vi "Beampointing_Multi_Pico3_HTT.vi"() -> ()   [LabVIEW 2020]
uses:
  Shared/GUI_Template/GUI_master/tcp_new_data_event.ctl
  Shared/GUI_Template/GUI_master/tcp new data cluster.ctl
  Ctrs/beam detection.ctl
  GUI_Beampointing_single_TRA/Ctrs/move.ctl
  General GUIs/Device GUIs/GUI_Cameras/Controls/Crosshair type def.ctl
  <vilib>/Utility/error.llb/DialogType.ctl
  <vilib>/Utility/file.llb/Read From Spreadsheet File (string).vi
  <userlib>/_OpenG.lib/array/array.llb/Filter 1D Array with Scalar (String)__ogtk.vi
  <userlib>/_OpenG.lib/array/array.llb/Filter 1D Array (String)__ogtk.vi
  <vilib>/Utility/file.llb/Write To Spreadsheet File (string).vi
  <vilib>/Analysis/NI_AALBase.lvlib
panel:
  out "x-y*floor(x/y)":dbl
  out "error out":errorcluster
  out "config path":string
  out "Array 3":bool[](array[boolean])
  out "Array 2":u16[](array[numeric])
  out "Array":u16[](array[numeric])
  out "Moving Y":string
  out "Moving X":string
  out "particles":T1(array[cluster])
  out "millisecond timer value":u32
  out "appended path":path
  out "millisecond timer 2":u32
  in  "GUIdevice 98":string="PicoPad_LCave"
  in  "Position.Axis 111::98":dbl=77.0 caption="Motor Axis 1" min=-999999.0 max=999999.0 format="%#_6f"
  in  "Position.Axis 112::98":dbl=77.0 caption="Motor Axis 1" min=-999999.0 max=999999.0 format="%#_6f"
  in  "Position.Axis 113::98":dbl=77.0 caption="Motor Axis 1" min=-999999.0 max=999999.0 format="%#_6f"
  in  "Position.Axis 121::98":dbl=77.0 caption="Motor Axis 1" min=-999999.0 max=999999.0 format="%#_6f"
  in  "Position.Axis 122::98":dbl=77.0 caption="Motor Axis 1" min=-999999.0 max=999999.0 format="%#_6f"
  in  "Position.Axis 123::98":dbl=77.0 caption="Motor Axis 1" min=-999999.0 max=999999.0 format="%#_6f"
  in  "Position.Axis 131::98":dbl=77.0 caption="Motor Axis 1" min=-999999.0 max=999999.0 format="%#_6f"
  in  "Position.Axis 132::98":dbl=77.0 caption="Motor Axis 1" min=-999999.0 max=999999.0 format="%#_6f"
  in  "Position.Axis 133::98":dbl=77.0 caption="Motor Axis 1" min=-999999.0 max=999999.0 format="%#_6f"
  in  "Position.Axis 141::98":dbl=77.0 caption="Motor Axis 1" min=-999999.0 max=999999.0 format="%#_6f"
  in  "Position.Axis 142::98":dbl=77.0 caption="Motor Axis 1" min=-999999.0 max=999999.0 format="%#_6f"
  in  "Position.Axis 143::98":dbl=77.0 caption="Motor Axis 1" min=-999999.0 max=999999.0 format="%#_6f"
  in  "Position.Axis 211::98":dbl=77.0 caption="Motor Axis 1" min=-999999.0 max=999999.0 format="%#_6f"
  in  "Position.Axis 212::98":dbl=77.0 caption="Motor Axis 1" min=-999999.0 max=999999.0 format="%#_6f"
  in  "Position.Axis 213::98":dbl=77.0 caption="Motor Axis 1" min=-999999.0 max=999999.0 format="%#_6f"
  in  "Position.Axis 221::98":dbl=77.0 caption="Motor Axis 1" min=-999999.0 max=999999.0 format="%#_6f"
  in  "Position.Axis 222::98":dbl=77.0 caption="Motor Axis 1" min=-999999.0 max=999999.0 format="%#_6f"
  in  "Position.Axis 223::98":dbl=77.0 caption="Motor Axis 1" min=-999999.0 max=999999.0 format="%#_6f"
  in  "Position.Axis 231::98":dbl=77.0 caption="Motor Axis 1" min=-999999.0 max=999999.0 format="%#_6f"
  in  "Position.Axis 232::98":dbl=77.0 caption="Motor Axis 1" min=-999999.0 max=999999.0 format="%#_6f"
  in  "Position.Axis 233::98":dbl=77.0 caption="Motor Axis 1" min=-999999.0 max=999999.0 format="%#_6f"
  in  "Position.Axis 241::98":dbl=77.0 caption="Motor Axis 1" min=-999999.0 max=999999.0 format="%#_6f"
  in  "Position.Axis 242::98":dbl=77.0 caption="Motor Axis 1" min=-999999.0 max=999999.0 format="%#_6f"
  in  "Position.Axis 243::98":dbl=77.0 caption="Motor Axis 1" min=-999999.0 max=999999.0 format="%#_6f"
  in  "Position.Axis 311::98":dbl=77.0 caption="Motor Axis 1" min=-999999.0 max=999999.0 format="%#_6f"
  in  "Position.Axis 312::98":dbl=77.0 caption="Motor Axis 1" min=-999999.0 max=999999.0 format="%#_6f"
  in  "Position.Axis 313::98":dbl=77.0 caption="Motor Axis 1" min=-999999.0 max=999999.0 format="%#_6f"
  in  "Position.Axis 321::98":dbl=77.0 caption="Motor Axis 1" min=-999999.0 max=999999.0 format="%#_6f"
  in  "Position.Axis 322::98":dbl=77.0 caption="Motor Axis 1" min=-999999.0 max=999999.0 format="%#_6f"
  in  "Position.Axis 323::98":dbl=77.0 caption="Motor Axis 1" min=-999999.0 max=999999.0 format="%#_6f"
  in  "Position.Axis 331::98":dbl=77.0 caption="Motor Axis 1" min=-999999.0 max=999999.0 format="%#_6f"
  in  "Position.Axis 332::98":dbl=77.0 caption="Motor Axis 1" min=-999999.0 max=999999.0 format="%#_6f"
  in  "Position.Axis 333::98":dbl=77.0 caption="Motor Axis 1" min=-999999.0 max=999999.0 format="%#_6f"
  in  "Position.Axis 341::98":dbl=77.0 caption="Motor Axis 1" min=-999999.0 max=999999.0 format="%#_6f"
  in  "Position.Axis 342::98":dbl=77.0 caption="Motor Axis 1" min=-999999.0 max=999999.0 format="%#_6f"
  in  "Position.Axis 343::98":dbl=77.0 caption="Motor Axis 1" min=-999999.0 max=999999.0 format="%#_6f"
  in  "Position.Axis 411::98":dbl=77.0 caption="Motor Axis 1" min=-999999.0 max=999999.0 format="%#_6f"
  in  "Position.Axis 412::98":dbl=77.0 caption="Motor Axis 1" min=-999999.0 max=999999.0 format="%#_6f"
  in  "Position.Axis 413::98":dbl=77.0 caption="Motor Axis 1" min=-999999.0 max=999999.0 format="%#_6f"
  in  "Position.Axis 421::98":dbl=77.0 caption="Motor Axis 1" min=-999999.0 max=999999.0 format="%#_6f"
  in  "Position.Axis 422::98":dbl=77.0 caption="Motor Axis 1" min=-999999.0 max=999999.0 format="%#_6f"
  in  "Position.Axis 423::98":dbl=77.0 caption="Motor Axis 1" min=-999999.0 max=999999.0 format="%#_6f"
  in  "Position.Axis 431::98":dbl=77.0 caption="Motor Axis 1" min=-999999.0 max=999999.0 format="%#_6f"
  in  "Position.Axis 432::98":dbl=77.0 caption="Motor Axis 1" min=-999999.0 max=999999.0 format="%#_6f"
  in  "Position.Axis 433::98":dbl=77.0 caption="Motor Axis 1" min=-999999.0 max=999999.0 format="%#_6f"
  in  "Position.Axis 441::98":dbl=77.0 caption="Motor Axis 1" min=-999999.0 max=999999.0 format="%#_6f"
  in  "Position.Axis 442::98":dbl=77.0 caption="Motor Axis 1" min=-999999.0 max=999999.0 format="%#_6f"
  in  "Position.Axis 443::98":dbl=77.0 caption="Motor Axis 1" min=-999999.0 max=999999.0 format="%#_6f"
  in  "Position.Axis 511::98":dbl=77.0 caption="Motor Axis 1" min=-999999.0 max=999999.0 format="%#_6f"
  in  "Position.Axis 512::98":dbl=77.0 caption="Motor Axis 1" min=-999999.0 max=999999.0 format="%#_6f"
  in  "Position.Axis 513::98":dbl=77.0 caption="Motor Axis 1" min=-999999.0 max=999999.0 format="%#_6f"
  in  "Position.Axis 521::98":dbl=77.0 caption="Motor Axis 1" min=-999999.0 max=999999.0 format="%#_6f"
  in  "Position.Axis 522::98":dbl=77.0 caption="Motor Axis 1" min=-999999.0 max=999999.0 format="%#_6f"
  in  "Position.Axis 523::98":dbl=77.0 caption="Motor Axis 1" min=-999999.0 max=999999.0 format="%#_6f"
  in  "Position.Axis 531::98":dbl=77.0 caption="Motor Axis 1" min=-999999.0 max=999999.0 format="%#_6f"
  in  "Position.Axis 532::98":dbl=77.0 caption="Motor Axis 1" min=-999999.0 max=999999.0 format="%#_6f"
  in  "Position.Axis 533::98":dbl=77.0 caption="Motor Axis 1" min=-999999.0 max=999999.0 format="%#_6f"
  in  "Position.Axis 541::98":dbl=77.0 caption="Motor Axis 1" min=-999999.0 max=999999.0 format="%#_6f"
  in  "Position.Axis 542::98":dbl=77.0 caption="Motor Axis 1" min=-999999.0 max=999999.0 format="%#_6f"
  in  "Position.Axis 543::98":dbl=77.0 caption="Motor Axis 1" min=-999999.0 max=999999.0 format="%#_6f"
  in  "Numeric":dbl
  out "Current State":string
  in  "output cluster 2":T5 {"detection para"."smal para"."Measurement Parameter" items=["Center of Mass X", "Center of Mass Y", "First Pixel X", "First Pixel Y", "Bounding Rect Left", "Bounding Rect Top", "Bounding Rect Right", "Bounding Rect Bottom", "Max Feret Diameter Start X", "Max Feret Diameter Start Y", "Max Feret Diameter End X", "Max Feret Diameter End Y", "Max Horiz. Segment Length Left", "Max Horiz. Segment Length Right", "Max Horiz. Segment Length Row", "-", "Bounding Rect Width", "Bounding Rect Height", "Bounding Rect Diagonal", "Perimeter", "Convex Hull Perimeter", "Holes' Perimeter", "Max Feret Diameter", "Equivalent Ellipse Major Axis", "Equivalent Ellipse Minor Axis", "Equivalent Ellipse Minor Axis (Feret)", "Equivalent Rect Long Side", "Equivalent Rect Short Side", "Equivalent Rect Diagonal", "Equivalent Rect Short Side (Feret)", "Average Horiz. Segment Length", "Average Vert. Segment Length", "Hydraulic Radius", "Waddel Disk Diameter", "-", "Area", "Holes' Area", "Particle & Holes' Area", "Convex Hull Area", "Image Area", "-", "Number of Holes", "Number of Horiz. Segments", "Number of Vert. Segments", "-", "Orientation", "Max Feret Diameter Orientation", "-", "% Area/Image Area", "% Area/(Particle & Holes' Area)", "Ratio of Equivalent Ellipse Axes", "Ratio of Equivalent Rect Sides", "-", "Elongation Factor", "Compactness Factor", "Heywood Circularity Factor", "Type Factor", "-", "Sum X", "Sum Y", "Sum XX", "Sum XY", "Sum YY", "Sum XXX", "Sum XXY", "Sum XYY", "Sum YYY", "-", "Moment of Inertia XX", "Moment of Inertia XY", "Moment of Inertia YY", "Moment of Inertia XXX", "Moment of Inertia XXY", "Moment of Inertia XYY", "Moment of Inertia YYY", "Norm. Moment of Inertia XX", "Norm. Moment of Inertia XY", "Norm. Moment of Inertia YY", "Norm. Moment of Inertia XXX", "Norm. Moment of Inertia XXY", "Norm. Moment of Inertia XYY", "Norm. Moment of Inertia YYY", "Hu Moment 1", "Hu Moment 2", "Hu Moment 3", "Hu Moment 4", "Hu Moment 5", "Hu Moment 6", "Hu Moment 7"]; "detection para"."smal para"."Range Lower Value" format="%.2f"; "detection para"."smal para"."Range Upper Value" format="%.2f"; "detection para"."detection method" items=["clustering", "entropy", "metric", "moments", "inter-class variance"]; "detection para"."Filter" items=["No Filter", "Median Filter", "Low Pass Filter"]}
  out "CCDs":string[](array[string])
  in  "GUIdevice 12":string
  in  "GUIdevice 11":string
  in  "GUIdevice 10":string
  in  "GUIdevice 9":string
  out "error out 2":errorcluster
  in  "active cams":string[](array[string])
  in  "Motor Y":dbl[][](array[numeric])
  in  "Motor X":dbl[][](array[numeric])
  out "Names":string[](array[string])
  in  "Offset X stats":dbl[][](array[numeric])
  in  "Offset Y stats":dbl[][](array[numeric])
  out "Box":T6(array[cluster])
  in  "Tab Control 2":enum32{"Config ", "Main", "History"}(tab)=enum."Main"
  out "Waveform Chart":u32(graph)
  in  "associated motors":T7 {"Motor CCD 12" items=["d1-frontend", "d2-amp2in", "d3-amp2out", "d4-amp3in", "d5-amp4in", "d6-amp4out", "s-input1", "s-input2", "d7-prepulse", "p1-probe", "Gaia S", "Gaia N", "s1-amp2in", "s2-amp2out", "s3-amp3in", "S4C4", "s4-sdelayout", "d9-compressor-out", "Gaia Scatter", "d8-telescope-in", "d1-frontend", "d2-amp2in", "d3-amp2out", "d4-amp3in", "d5-amp4in", "d6-amp4out", "s-input1", "s-input2", "d7-prepulse", "p1-probe", "Gaia S", "Gaia N", "s1-amp2in", "s2-amp2out", "s3-amp3in", "S4C4", "s4-sdelayout", "d9-compressor-out", "Gaia Scatter", "d8-telescope-in"]; "Motor CCD 11" items=["d1-frontend", "d2-amp2in", "d3-amp2out", "d4-amp3in", "d5-amp4in", "d6-amp4out", "s-input1", "s-input2", "d7-prepulse", "p1-probe", "Gaia S", "Gaia N", "s1-amp2in", "s2-amp2out", "s3-amp3in", "S4C4", "s4-sdelayout", "d9-compressor-out", "Gaia Scatter", "d8-telescope-in", "d1-frontend", "d2-amp2in", "d3-amp2out", "d4-amp3in", "d5-amp4in", "d6-amp4out", "s-input1", "s-input2", "d7-prepulse", "p1-probe", "Gaia S", "Gaia N", "s1-amp2in", "s2-amp2out", "s3-amp3in", "S4C4", "s4-sdelayout", "d9-compressor-out", "Gaia Scatter", "d8-telescope-in"]; "Motor CCD 10" items=["d1-frontend", "d2-amp2in", "d3-amp2out", "d4-amp3in", "d5-amp4in", "d6-amp4out", "s-input1", "s-input2", "d7-prepulse", "p1-probe", "Gaia S", "Gaia N", "s1-amp2in", "s2-amp2out", "s3-amp3in", "S4C4", "s4-sdelayout", "d9-compressor-out", "Gaia Scatter", "d8-telescope-in", "d1-frontend", "d2-amp2in", "d3-amp2out", "d4-amp3in", "d5-amp4in", "d6-amp4out", "s-input1", "s-input2", "d7-prepulse", "p1-probe", "Gaia S", "Gaia N", "s1-amp2in", "s2-amp2out", "s3-amp3in", "S4C4", "s4-sdelayout", "d9-compressor-out", "Gaia Scatter", "d8-telescope-in"]; "Motor CCD 9" items=["d1-frontend", "d2-amp2in", "d3-amp2out", "d4-amp3in", "d5-amp4in", "d6-amp4out", "s-input1", "s-input2", "d7-prepulse", "p1-probe", "Gaia S", "Gaia N", "s1-amp2in", "s2-amp2out", "s3-amp3in", "S4C4", "s4-sdelayout", "d9-compressor-out", "Gaia Scatter", "d8-telescope-in", "d1-frontend", "d2-amp2in", "d3-amp2out", "d4-amp3in", "d5-amp4in", "d6-amp4out", "s-input1", "s-input2", "d7-prepulse", "p1-probe", "Gaia S", "Gaia N", "s1-amp2in", "s2-amp2out", "s3-amp3in", "S4C4", "s4-sdelayout", "d9-compressor-out", "Gaia Scatter", "d8-telescope-in"]; "Motor CCD 8" items=["d1-frontend", "d2-amp2in", "d3-amp2out", "d4-amp3in", "d5-amp4in", "d6-amp4out", "s-input1", "s-input2", "d7-prepulse", "p1-probe", "Gaia S", "Gaia N", "s1-amp2in", "s2-amp2out", "s3-amp3in", "S4C4", "s4-sdelayout", "d9-compressor-out", "Gaia Scatter", "d8-telescope-in", "d1-frontend", "d2-amp2in", "d3-amp2out", "d4-amp3in", "d5-amp4in", "d6-amp4out", "s-input1", "s-input2", "d7-prepulse", "p1-probe", "Gaia S", "Gaia N", "s1-amp2in", "s2-amp2out", "s3-amp3in", "S4C4", "s4-sdelayout", "d9-compressor-out", "Gaia Scatter", "d8-telescope-in"]; "Motor CCD 7" items=["d1-frontend", "d2-amp2in", "d3-amp2out", "d4-amp3in", "d5-amp4in", "d6-amp4out", "s-input1", "s-input2", "d7-prepulse", "p1-probe", "Gaia S", "Gaia N", "s1-amp2in", "s2-amp2out", "s3-amp3in", "S4C4", "s4-sdelayout", "d9-compressor-out", "Gaia Scatter", "d8-telescope-in", "d1-frontend", "d2-amp2in", "d3-amp2out", "d4-amp3in", "d5-amp4in", "d6-amp4out", "s-input1", "s-input2", "d7-prepulse", "p1-probe", "Gaia S", "Gaia N", "s1-amp2in", "s2-amp2out", "s3-amp3in", "S4C4", "s4-sdelayout", "d9-compressor-out", "Gaia Scatter", "d8-telescope-in"]; "Motor CCD 6" items=["d1-frontend", "d2-amp2in", "d3-amp2out", "d4-amp3in", "d5-amp4in", "d6-amp4out", "s-input1", "s-input2", "d7-prepulse", "p1-probe", "Gaia S", "Gaia N", "s1-amp2in", "s2-amp2out", "s3-amp3in", "S4C4", "s4-sdelayout", "d9-compressor-out", "Gaia Scatter", "d8-telescope-in", "d1-frontend", "d2-amp2in", "d3-amp2out", "d4-amp3in", "d5-amp4in", "d6-amp4out", "s-input1", "s-input2", "d7-prepulse", "p1-probe", "Gaia S", "Gaia N", "s1-amp2in", "s2-amp2out", "s3-amp3in", "S4C4", "s4-sdelayout", "d9-compressor-out", "Gaia Scatter", "d8-telescope-in"]; "Motor CCD 5" items=["d1-frontend", "d2-amp2in", "d3-amp2out", "d4-amp3in", "d5-amp4in", "d6-amp4out", "s-input1", "s-input2", "d7-prepulse", "p1-probe", "Gaia S", "Gaia N", "s1-amp2in", "s2-amp2out", "s3-amp3in", "S4C4", "s4-sdelayout", "d9-compressor-out", "Gaia Scatter", "d8-telescope-in", "d1-frontend", "d2-amp2in", "d3-amp2out", "d4-amp3in", "d5-amp4in", "d6-amp4out", "s-input1", "s-input2", "d7-prepulse", "p1-probe", "Gaia S", "Gaia N", "s1-amp2in", "s2-amp2out", "s3-amp3in", "S4C4", "s4-sdelayout", "d9-compressor-out", "Gaia Scatter", "d8-telescope-in"]; "Motor CCD 4" items=["d1-frontend", "d2-amp2in", "d3-amp2out", "d4-amp3in", "d5-amp4in", "d6-amp4out", "s-input1", "s-input2", "d7-prepulse", "p1-probe", "Gaia S", "Gaia N", "s1-amp2in", "s2-amp2out", "s3-amp3in", "S4C4", "s4-sdelayout", "d9-compressor-out", "Gaia Scatter", "d8-telescope-in", "d1-frontend", "d2-amp2in", "d3-amp2out", "d4-amp3in", "d5-amp4in", "d6-amp4out", "s-input1", "s-input2", "d7-prepulse", "p1-probe", "Gaia S", "Gaia N", "s1-amp2in", "s2-amp2out", "s3-amp3in", "S4C4", "s4-sdelayout", "d9-compressor-out", "Gaia Scatter", "d8-telescope-in"]; "Motor CCD 3" items=["d1-frontend", "d2-amp2in", "d3-amp2out", "d4-amp3in", "d5-amp4in", "d6-amp4out", "s-input1", "s-input2", "d7-prepulse", "p1-probe", "Gaia S", "Gaia N", "s1-amp2in", "s2-amp2out", "s3-amp3in", "S4C4", "s4-sdelayout", "d9-compressor-out", "Gaia Scatter", "d8-telescope-in", "d1-frontend", "d2-amp2in", "d3-amp2out", "d4-amp3in", "d5-amp4in", "d6-amp4out", "s-input1", "s-input2", "d7-prepulse", "p1-probe", "Gaia S", "Gaia N", "s1-amp2in", "s2-amp2out", "s3-amp3in", "S4C4", "s4-sdelayout", "d9-compressor-out", "Gaia Scatter", "d8-telescope-in"]; "Motor CCD 2" items=["d1-frontend", "d2-amp2in", "d3-amp2out", "d4-amp3in", "d5-amp4in", "d6-amp4out", "s-input1", "s-input2", "d7-prepulse", "p1-probe", "Gaia S", "Gaia N", "s1-amp2in", "s2-amp2out", "s3-amp3in", "S4C4", "s4-sdelayout", "d9-compressor-out", "Gaia Scatter", "d8-telescope-in", "d1-frontend", "d2-amp2in", "d3-amp2out", "d4-amp3in", "d5-amp4in", "d6-amp4out", "s-input1", "s-input2", "d7-prepulse", "p1-probe", "Gaia S", "Gaia N", "s1-amp2in", "s2-amp2out", "s3-amp3in", "S4C4", "s4-sdelayout", "d9-compressor-out", "Gaia Scatter", "d8-telescope-in"]; "Motor CCD 1" items=["d1-frontend", "d2-amp2in", "d3-amp2out", "d4-amp3in", "d5-amp4in", "d6-amp4out", "s-input1", "s-input2", "d7-prepulse", "p1-probe", "Gaia S", "Gaia N", "s1-amp2in", "s2-amp2out", "s3-amp3in", "S4C4", "s4-sdelayout", "d9-compressor-out", "Gaia Scatter", "d8-telescope-in", "d1-frontend", "d2-amp2in", "d3-amp2out", "d4-amp3in", "d5-amp4in", "d6-amp4out", "s-input1", "s-input2", "d7-prepulse", "p1-probe", "Gaia S", "Gaia N", "s1-amp2in", "s2-amp2out", "s3-amp3in", "S4C4", "s4-sdelayout", "d9-compressor-out", "Gaia Scatter", "d8-telescope-in"]}
  out "Cameras":T8
  out "Status":cluster{i32, i32, "Centroid X":dbl[][]}(graph)
  in  "Exposure:12":dbl=0.095 min=0.0001 max=1.0 format="%#_6f"
  in  "Triggerdelay::12":dbl=0.003 min=0.0 max=0.09 format="%#_6f"
  in  "Exposure::11":dbl=0.095 min=0.0001 max=1.0 format="%#_6f"
  in  "Triggerdelay::11":dbl=0.003 min=0.0 max=0.09 format="%#_6f"
  in  "Exposure::10":dbl=0.095 min=0.0001 max=1.0 format="%#_6f"
  in  "Triggerdelay::10":dbl=0.003 min=0.0 max=0.09 format="%#_6f"
  in  "Exposure::9":dbl=0.095 min=0.0001 max=1.0 format="%#_6f"
  in  "Triggerdelay::9":dbl=0.003 min=0.0 max=0.09 format="%#_6f"
  in  "Trigger::9":bool
  in  "Trigger::10":bool caption="Trigger:10"
  in  "Trigger::11":bool
  in  "Trigger::12":bool
  in  "Target.Y::9":dbl=45.0 caption="T9y" min=0.0 max=2000.0 format="%#_6f"
  in  "Target.X::9":dbl=47.0 caption="Tx9" min=0.0 max=2000.0 format="%#_6f"
  in  "Target.Y::10":dbl=45.0 caption="T10y" min=0.0 max=2000.0 format="%#_6f"
  in  "Target.X::10":dbl=47.0 caption="T10x" min=0.0 max=2000.0 format="%#_6f"
  in  "Target.Y::11":dbl=45.0 caption="T11y" min=0.0 max=2000.0 format="%#_6f"
  in  "Target.X::11":dbl=47.0 caption="T11x" min=0.0 max=2000.0 format="%#_6f"
  in  "Target.Y::12":dbl=45.0 caption="T12y" min=0.0 max=2000.0 format="%#_6f"
  in  "Target.X::12":dbl=47.0 caption="T12x" min=0.0 max=2000.0 format="%#_6f"
  in  "Exposure::8":dbl=0.095 min=0.0001 max=1.0 format="%#_6f"
  in  "Triggerdelay::8":dbl=0.003 min=0.0 max=0.09 format="%#_6f"
  in  "Trigger::8":bool
  in  "Target.Y::8":dbl=45.0 caption="T8y" min=0.0 max=2000.0 format="%#_6f"
  in  "Target.X::8":dbl=47.0 caption="T8x" min=0.0 max=2000.0 format="%#_6f"
  in  "Target.Y::7":dbl=45.0 caption="T7x" min=0.0 max=2000.0 format="%#_6f"
  in  "Target.X::7":dbl=47.0 caption="T7y" min=0.0 max=2000.0 format="%#_6f"
  in  "Target.Y::6":dbl=45.0 caption="T6y" min=1.0 max=600.0 format="%#_6f"
  in  "Target.X::6":dbl=47.0 caption="T6x" min=1.0 max=800.0 format="%#_6f"
  in  "Target.Y::5":dbl=45.0 caption="T5y" min=0.0 max=2000.0 format="%#_6f"
  in  "Target.X::5":dbl=47.0 caption="T5x" min=0.0 max=2000.0 format="%#_6f"
  in  "Target.Y::4":dbl=45.0 caption="T4y" min=1.0 max=600.0 format="%#_6f"
  in  "Target.X::4":dbl=47.0 caption="T4x" min=1.0 max=800.0 format="%#_6f"
  in  "Target.Y::3":dbl=163.0 caption="T3y" min=0.0 max=2000.0 format="%#_6f"
  in  "Target.X::3":dbl=152.0 caption="T3x" min=0.0 max=2000.0 format="%#_6f"
  in  "Target.Y::2":dbl=74.0 caption="T2y" min=0.0 max=2000.0 format="%#_6f"
  in  "Target.X::2":dbl=75.0 caption="T2x" min=0.0 max=2000.0 format="%#_6f"
  in  "Target.Y::1":dbl=61.0 caption="T1y" min=0.0 max=2000.0 format="%#_6f"
  in  "Target.X::1":dbl=77.0 caption="T1x" min=0.0 max=2000.0 format="%#_6f"
  in  "Exposure::7":dbl=0.095 min=0.0001 max=1.0 format="%#_6f"
  in  "Triggerdelay::7":dbl=0.003 min=0.0 max=50000.0 format="%#_6f"
  in  "Trigger::7":bool
  in  "Exposure::6":dbl=0.095 min=0.0001 max=1.0 format="%#_6f"
  in  "Triggerdelay::6":dbl=0.003 min=0.0 max=0.09 format="%#_6f"
  in  "Trigger::6":bool
  in  "Exposure::5":dbl=0.095 min=1e-05 max=2.0 format="%#_6f"
  in  "Triggerdelay::5":dbl=0.003 min=0.0 max=100000.0 format="%#_6f"
  in  "Trigger::5":bool
  in  "Exposure::4":dbl=0.095 min=0.0001 max=1.0 format="%#_6f"
  in  "Triggerdelay::4":dbl=0.003 min=0.0 max=0.09 format="%#_6f"
  in  "Trigger::4":bool
  in  "Exposure::3":dbl=0.095 min=1.0 max=999999.0 format="%#_6f"
  in  "Triggerdelay::3":dbl=0.003 min=0.0 max=99999.0 format="%#_6f"
  in  "Trigger::3":bool
  in  "Exposure::2":dbl=0.095 min=0.0001 max=1000001.0 format="%#_6f"
  in  "Triggerdelay::2":dbl=0.003 min=0.0 max=100000.0 format="%#_6f"
  in  "Trigger::2":bool
  out "image::1":T9(plugin-control) caption="BellaCam46_2_Scatter_In_1"
  out "image::2":T9(plugin-control) caption="BellaCam32_3"
  out "image::3":T9(plugin-control)
  out "image::4":T9(plugin-control)
  out "image::5":T9(plugin-control)
  out "image::6":T9(plugin-control)
  out "image::7":T9(plugin-control)
  out "image::8":T9(plugin-control)
  in  "Exposure::1":dbl=0.095 caption="exposure" min=0.0 max=1.0 format="%#_6f"
  in  "Triggerdelay::1":dbl=0.003 caption="trig delay" min=0.0 max=1.0 format="%#_6f"
  in  "Trigger::1":bool
  in  "UDP error message":string
  out "required Y":bool[](array[boolean])
  out "required X":bool[](array[boolean])
  out "detected":bool[](array[boolean])
  out "name array":string[](array[string])
  out "image::9":T9(plugin-control)
  out "image::10":T9(plugin-control)
  out "image::11":T9(plugin-control)
  out "image::12":T9(plugin-control)
  out "speedmode X":bool[](array[boolean])
  out "speedmode Y":bool[](array[boolean])
  out "CCD 9":cluster{timestamp[], dbl[]}[](graph)
  out "CCD 10":cluster{timestamp[], dbl[]}[](graph)
  out "CCD 11":cluster{timestamp[], dbl[]}[](graph)
  out "CCD 12":cluster{timestamp[], dbl[]}[](graph)
  out "CCD 5":cluster{timestamp[], dbl[]}[](graph)
  out "CCD 6":cluster{timestamp[], dbl[]}[](graph)
  out "CCD 7":cluster{timestamp[], dbl[]}[](graph)
  out "CCD 8":cluster{timestamp[], dbl[]}[](graph)
  out "CCD 2":cluster{timestamp[], dbl[]}[](graph)
  out "CCD 1":cluster{timestamp[], dbl[]}[](graph)
  out "CCD 3":cluster{timestamp[], dbl[]}[](graph)
  out "CCD 4":cluster{timestamp[], dbl[]}[](graph)
  out "History index":i32
  in  "History Size":i32=500
  out "Particle Reports (Pixels)":T10(array[cluster])
  in  "Feedback Global":bool
  in  "detection para":T3[](array[typedef])=[{"Filter"=1, "Filter Para"={"X Size"=5, "Y Size"=5, "% Tolerance"=1}, "detection method"=4, "smal para"=[{"Measurement Parameter"=35, "Range Lower Value"=0.0, "Range Upper Value"=0.0, "Range"=TRUE, "Measurement Type"=FALSE}], "Remove small Objects"=TRUE, "Restrict to round Objects"=FALSE}, {"Filter"=1, "Filter Para"={"X Size"=5, "Y Size"=5, "% Tolerance"=1}, "detection method"=4, "smal para"=[{"Measurement Parameter"=35, "Range Lower Value"=0.0, "Range Upper Value"=500.0, "Range"=FALSE, "Measurement Type"=FALSE}], "Remove small Objects"=TRUE, "Restrict to round Objects"=FALSE}, {"Filter"=1, "Filter Para"={"X Size"=5, "Y Size"=5, "% Tolerance"=1}, "detection method"=4, "smal para"=[{"Measurement Parameter"=35, "Range Lower Value"=0.0, "Range Upper Value"=500.0, "Range"=TRUE, "Measurement Type"=FALSE}], "Remove small Objects"=TRUE, "Restrict to round Objects"=FALSE}, {"Filter"=1, "Filter Para"={"X Size"=5, "Y Size"=5, "% Tolerance"=1}, "detection method"=4, "smal para"=[{"Measurement Parameter"=35, "Range Lower Value"=0.0, "Range Upper Value"=500.0, "Range"=TRUE, "Measurement Type"=FALSE}], "Remove small Objects"=TRUE, "Restrict to round Objects"=FALSE}, {"Filter"=1, "Filter Para"={"X Size"=5, "Y Size"=5, "% Tolerance"=1}, "detection method"=4, "smal para"=[{"Measurement Parameter"=35, "Range Lower Value"=0.0, "Range Upper Value"=500.0, "Range"=TRUE, "Measurement Type"=FALSE}], "Remove small Objects"=TRUE, "Restrict to round Objects"=FALSE}, {"Filter"=1, "Filter Para"={"X Size"=5, "Y Size"=5, "% Tolerance"=1}, "detection method"=4, "smal para"=[{"Measurement Parameter"=35, "Range Lower Value"=0.0, "Range Upper Value"=500.0, "Range"=TRUE, "Measurement Type"=FALSE}], "Remove small Objects"=TRUE, "Restrict to round Objects"=FALSE}, {"Filter"=1, "Filter Para"={"X Size"=5, "Y Size"=5, "% Tolerance"=1}, "detection method"=4, "smal para"=[{"Measurement Parameter"=35, "Range Lower Value"=0.0, "Range Upper Value"=500.0, "Range"=TRUE, "Measurement Type"=FALSE}], "Remove small Objects"=TRUE, "Restrict to round Objects"=FALSE}, {"Filter"=1, "Filter Para"={"X Size"=5, "Y Size"=5, "% Tolerance"=1}, "detection method"=3, "smal para"=[{"Measurement Parameter"=35, "Range Lower Value"=0.0, "Range Upper Value"=0.0, "Range"=FALSE, "Measurement Type"=FALSE}], "Remove small Objects"=TRUE, "Restrict to round Objects"=FALSE}, {"Filter"=1, "Filter Para"={"X Size"=5, "Y Size"=5, "% Tolerance"=1}, "detection method"=4, "smal para"=[{"Measurement Parameter"=35, "Range Lower Value"=0.0, "Range Upper Value"=0.0, "Range"=FALSE, "Measurement Type"=FALSE}], "Remove small Objects"=TRUE, "Restrict to round Objects"=FALSE}, {"Filter"=1, "Filter Para"={"X Size"=5, "Y Size"=5, "% Tolerance"=1}, "detection method"=4, "smal para"=[{"Measurement Parameter"=35, "Range Lower Value"=0.0, "Range Upper Value"=500.0, "Range"=TRUE, "Measurement Type"=FALSE}], "Remove small Objects"=TRUE, "Restrict to round Objects"=FALSE}, {"Filter"=1, "Filter Para"={"X Size"=5, "Y Size"=5, "% Tolerance"=1}, "detection method"=4, "smal para"=[{"Measurement Parameter"=35, "Range Lower Value"=0.0, "Range Upper Value"=500.0, "Range"=TRUE, "Measurement Type"=FALSE}], "Remove small Objects"=TRUE, "Restrict to round Objects"=FALSE}, {"Filter"=1, "Filter Para"={"X Size"=5, "Y Size"=5, "% Tolerance"=1}, "detection method"=4, "smal para"=[{"Measurement Parameter"=35, "Range Lower Value"=0.0, "Range Upper Value"=500.0, "Range"=TRUE, "Measurement Type"=FALSE}], "Remove small Objects"=TRUE, "Restrict to round Objects"=FALSE}] {"smal para"."Measurement Parameter" items=["Center of Mass X", "Center of Mass Y", "First Pixel X", "First Pixel Y", "Bounding Rect Left", "Bounding Rect Top", "Bounding Rect Right", "Bounding Rect Bottom", "Max Feret Diameter Start X", "Max Feret Diameter Start Y", "Max Feret Diameter End X", "Max Feret Diameter End Y", "Max Horiz. Segment Length Left", "Max Horiz. Segment Length Right", "Max Horiz. Segment Length Row", "-", "Bounding Rect Width", "Bounding Rect Height", "Bounding Rect Diagonal", "Perimeter", "Convex Hull Perimeter", "Holes' Perimeter", "Max Feret Diameter", "Equivalent Ellipse Major Axis", "Equivalent Ellipse Minor Axis", "Equivalent Ellipse Minor Axis (Feret)", "Equivalent Rect Long Side", "Equivalent Rect Short Side", "Equivalent Rect Diagonal", "Equivalent Rect Short Side (Feret)", "Average Horiz. Segment Length", "Average Vert. Segment Length", "Hydraulic Radius", "Waddel Disk Diameter", "-", "Area", "Holes' Area", "Particle & Holes' Area", "Convex Hull Area", "Image Area", "-", "Number of Holes", "Number of Horiz. Segments", "Number of Vert. Segments", "-", "Orientation", "Max Feret Diameter Orientation", "-", "% Area/Image Area", "% Area/(Particle & Holes' Area)", "Ratio of Equivalent Ellipse Axes", "Ratio of Equivalent Rect Sides", "-", "Elongation Factor", "Compactness Factor", "Heywood Circularity Factor", "Type Factor", "-", "Sum X", "Sum Y", "Sum XX", "Sum XY", "Sum YY", "Sum XXX", "Sum XXY", "Sum XYY", "Sum YYY", "-", "Moment of Inertia XX", "Moment of Inertia XY", "Moment of Inertia YY", "Moment of Inertia XXX", "Moment of Inertia XXY", "Moment of Inertia XYY", "Moment of Inertia YYY", "Norm. Moment of Inertia XX", "Norm. Moment of Inertia XY", "Norm. Moment of Inertia YY", "Norm. Moment of Inertia XXX", "Norm. Moment of Inertia XXY", "Norm. Moment of Inertia XYY", "Norm. Moment of Inertia YYY", "Hu Moment 1", "Hu Moment 2", "Hu Moment 3", "Hu Moment 4", "Hu Moment 5", "Hu Moment 6", "Hu Moment 7"]; "smal para"."Range Lower Value" format="%.2f"; "smal para"."Range Upper Value" format="%.2f"; "detection method" items=["clustering", "entropy", "metric", "moments", "inter-class variance"]; "Filter" items=["No Filter", "Median Filter", "Low Pass Filter"]}
  in  "GUIdevice 8":string
  in  "Tab Control":T11(tab)
  in  "Center":bool
  in  "Save Stats":bool
  in  "Save Config":bool
  in  "Load Config":bool
  in  "update speed [ms]":i32=2000
  in  "Img to avg":i32=15 min=3 max=200
  in  "Reset History":bool
  in  "save path":path=path "W:/BP_DATA"
  in  "autodetect":bool
  in  "Detection Rate":dbl=0.8 min=0.001 max=1.0
  in  "new tdms":bool
  in  "Speedmode @":dbl=3.0 min=1.0 max=20.0
  in  "Align":bool
  in  "deivice ini":bool
  in  "beam detection para":T3={"Filter"=1, "Filter Para"={"X Size"=5, "Y Size"=5, "% Tolerance"=1}, "detection method"=4, "smal para"=[{"Measurement Parameter"=35, "Range Lower Value"=0.0, "Range Upper Value"=500.0, "Range"=FALSE, "Measurement Type"=FALSE}], "Remove small Objects"=TRUE, "Restrict to round Objects"=FALSE} {"smal para"."Measurement Parameter" items=["Center of Mass X", "Center of Mass Y", "First Pixel X", "First Pixel Y", "Bounding Rect Left", "Bounding Rect Top", "Bounding Rect Right", "Bounding Rect Bottom", "Max Feret Diameter Start X", "Max Feret Diameter Start Y", "Max Feret Diameter End X", "Max Feret Diameter End Y", "Max Horiz. Segment Length Left", "Max Horiz. Segment Length Right", "Max Horiz. Segment Length Row", "-", "Bounding Rect Width", "Bounding Rect Height", "Bounding Rect Diagonal", "Perimeter", "Convex Hull Perimeter", "Holes' Perimeter", "Max Feret Diameter", "Equivalent Ellipse Major Axis", "Equivalent Ellipse Minor Axis", "Equivalent Ellipse Minor Axis (Feret)", "Equivalent Rect Long Side", "Equivalent Rect Short Side", "Equivalent Rect Diagonal", "Equivalent Rect Short Side (Feret)", "Average Horiz. Segment Length", "Average Vert. Segment Length", "Hydraulic Radius", "Waddel Disk Diameter", "-", "Area", "Holes' Area", "Particle & Holes' Area", "Convex Hull Area", "Image Area", "-", "Number of Holes", "Number of Horiz. Segments", "Number of Vert. Segments", "-", "Orientation", "Max Feret Diameter Orientation", "-", "% Area/Image Area", "% Area/(Particle & Holes' Area)", "Ratio of Equivalent Ellipse Axes", "Ratio of Equivalent Rect Sides", "-", "Elongation Factor", "Compactness Factor", "Heywood Circularity Factor", "Type Factor", "-", "Sum X", "Sum Y", "Sum XX", "Sum XY", "Sum YY", "Sum XXX", "Sum XXY", "Sum XYY", "Sum YYY", "-", "Moment of Inertia XX", "Moment of Inertia XY", "Moment of Inertia YY", "Moment of Inertia XXX", "Moment of Inertia XXY", "Moment of Inertia XYY", "Moment of Inertia YYY", "Norm. Moment of Inertia XX", "Norm. Moment of Inertia XY", "Norm. Moment of Inertia YY", "Norm. Moment of Inertia XXX", "Norm. Moment of Inertia XXY", "Norm. Moment of Inertia XYY", "Norm. Moment of Inertia YYY", "Hu Moment 1", "Hu Moment 2", "Hu Moment 3", "Hu Moment 4", "Hu Moment 5", "Hu Moment 6", "Hu Moment 7"]; "smal para"."Range Lower Value" format="%.2f"; "smal para"."Range Upper Value" format="%.2f"; "detection method" items=["clustering", "entropy", "metric", "moments", "inter-class variance"]; "Filter" items=["No Filter", "Median Filter", "Low Pass Filter"]}
  in  "move config":T2={"Tolerance [%]"=0.1, "Stepsize"=0.0001, "Invert Axis"=TRUE, "Invert Direction X"=FALSE, "Invert Direction Y"=TRUE, "enable feedback"=FALSE, "Set Centriod Target"=FALSE}
  in  "ActiveMotor":u16(ring)=7 items=["d1-frontend", "d2-amp2in", "d3-amp2out", "d4-amp3in", "d5-amp4in", "d6-amp4out", "s-input1", "s-input2", "d7-prepulse", "p1-probe", "Gaia S", "Gaia N", "s1-amp2in", "s2-amp2out", "s3-amp3in", "S4C4", "s4-sdelayout", "d9-compressor-out", "Gaia Scatter", "d8-telescope-in"]
  in  "ActiveMotorName::99":string
  in  "RelativeMove.Axis 1.CCW::99":bool caption="RelativeMove.Axis 1.CCW::1"
  in  "RelativeMove.Axis 1.CW::99":bool caption="RelativeMove.Axis 1.CW::1"
  in  "RelativeMove.Axis 2.CCW::99":bool caption="RelativeMove.Axis. 2.CCW::1"
  in  "RelativeMove.Axis 2.CW::99":bool caption="RelativeMove.Axis 2.CW::1"
  in  "RelativeSettings.Axis 1.Position::99":dbl caption="Axis 1 Position" min=-999999.0 max=999999.0 format="%_4p"
  in  "RelativeSettings.Axis 2.Position::99":dbl caption="Axis 2 Position" min=-999999.0 max=999999.0 format="%_4p"
  in  "RelativeSettings.Axis 2.StepSize::99":dbl=50.0 caption="Axis 2 StepSize" min=0.0 max=999999.0 format="%_4p"
  in  "RelativeSettings.Axis 1.StepSize::99":dbl=50.0 caption="Axis 1 Stepsize" min=0.0 max=999999.0 format="%_4p"
  out "Arguments Y":string
  in  "active axis refs 2":T12(array[cluster])
  in  "active Axis ref":cluster{"Ref X":refnum<vi>, "Ref Y":refnum<vi>}
  in  "CCDs":u16(ring) items=["BellaCam46_2_Scatter_In_1", "BellaCam32_3", "", "", "", "", "", "", "", "", "", ""]
  out "motor refs":refnum<vi>[](array[refnum])
  in  "Position.Axis 511::99":dbl=77.0 caption="Motor Axis 1" min=-999999.0 max=999999.0 format="%#_6f"
  in  "Position.Axis 512::99":dbl=77.0 caption="Motor Axis 1" min=-999999.0 max=999999.0 format="%#_6f"
  in  "Position.Axis 513::99":dbl=77.0 caption="Motor Axis 1" min=-999999.0 max=999999.0 format="%#_6f"
  in  "Position.Axis 521::99":dbl=77.0 caption="Motor Axis 1" min=-999999.0 max=999999.0 format="%#_6f"
  in  "Position.Axis 522::99":dbl=77.0 caption="Motor Axis 1" min=-999999.0 max=999999.0 format="%#_6f"
  in  "Position.Axis 523::99":dbl=77.0 caption="Motor Axis 1" min=-999999.0 max=999999.0 format="%#_6f"
  in  "Position.Axis 531::99":dbl=77.0 caption="Motor Axis 1" min=-999999.0 max=999999.0 format="%#_6f"
  in  "Position.Axis 532::99":dbl=77.0 caption="Motor Axis 1" min=-999999.0 max=999999.0 format="%#_6f"
  in  "Position.Axis 533::99":dbl=77.0 caption="Motor Axis 1" min=-999999.0 max=999999.0 format="%#_6f"
  in  "Position.Axis 541::99":dbl=77.0 caption="Motor Axis 1" min=-999999.0 max=999999.0 format="%#_6f"
  in  "Position.Axis 542::99":dbl=77.0 caption="Motor Axis 1" min=-999999.0 max=999999.0 format="%#_6f"
  in  "Position.Axis 543::99":dbl=77.0 caption="Motor Axis 1" min=-999999.0 max=999999.0 format="%#_6f"
  in  "Position.Axis 411::99":dbl=77.0 caption="Motor Axis 1" min=-999999.0 max=999999.0 format="%#_6f"
  in  "Position.Axis 412::99":dbl=77.0 caption="Motor Axis 1" min=-999999.0 max=999999.0 format="%#_6f"
  in  "Position.Axis 413::99":dbl=77.0 caption="Motor Axis 1" min=-999999.0 max=999999.0 format="%#_6f"
  in  "Position.Axis 421::99":dbl=77.0 caption="Motor Axis 1" min=-999999.0 max=999999.0 format="%#_6f"
  in  "Position.Axis 422::99":dbl=77.0 caption="Motor Axis 1" min=-999999.0 max=999999.0 format="%#_6f"
  in  "Position.Axis 423::99":dbl=77.0 caption="Motor Axis 1" min=-999999.0 max=999999.0 format="%#_6f"
  in  "Position.Axis 431::99":dbl=77.0 caption="Motor Axis 1" min=-999999.0 max=999999.0 format="%#_6f"
  in  "Position.Axis 432::99":dbl=77.0 caption="Motor Axis 1" min=-999999.0 max=999999.0 format="%#_6f"
  in  "Position.Axis 433::99":dbl=77.0 caption="Motor Axis 1" min=-999999.0 max=999999.0 format="%#_6f"
  in  "Position.Axis 441::99":dbl=77.0 caption="Motor Axis 1" min=-999999.0 max=999999.0 format="%#_6f"
  in  "Position.Axis 442::99":dbl=77.0 caption="Motor Axis 1" min=-999999.0 max=999999.0 format="%#_6f"
  in  "Position.Axis 443::99":dbl=77.0 caption="Motor Axis 1" min=-999999.0 max=999999.0 format="%#_6f"
  in  "Position.Axis 311::99":dbl=77.0 caption="Motor Axis 1" min=-999999.0 max=999999.0 format="%#_6f"
  in  "Position.Axis 312::99":dbl=77.0 caption="Motor Axis 1" min=-999999.0 max=999999.0 format="%#_6f"
  in  "Position.Axis 313::99":dbl=77.0 caption="Motor Axis 1" min=-999999.0 max=999999.0 format="%#_6f"
  in  "Position.Axis 321::99":dbl=77.0 caption="Motor Axis 1" min=-999999.0 max=999999.0 format="%#_6f"
  in  "Position.Axis 322::99":dbl=77.0 caption="Motor Axis 1" min=-999999.0 max=999999.0 format="%#_6f"
  in  "Position.Axis 323::99":dbl=77.0 caption="Motor Axis 1" min=-999999.0 max=999999.0 format="%#_6f"
  in  "Position.Axis 331::99":dbl=77.0 caption="Motor Axis 1" min=-999999.0 max=999999.0 format="%#_6f"
  in  "Position.Axis 332::99":dbl=77.0 caption="Motor Axis 1" min=-999999.0 max=999999.0 format="%#_6f"
  in  "Position.Axis 333::99":dbl=77.0 caption="Motor Axis 1" min=-999999.0 max=999999.0 format="%#_6f"
  in  "Position.Axis 341::99":dbl=77.0 caption="Motor Axis 1" min=-999999.0 max=999999.0 format="%#_6f"
  in  "Position.Axis 342::99":dbl=77.0 caption="Motor Axis 1" min=-999999.0 max=999999.0 format="%#_6f"
  in  "Position.Axis 343::99":dbl=77.0 caption="Motor Axis 1" min=-999999.0 max=999999.0 format="%#_6f"
  in  "Position.Axis 241::99":dbl=77.0 caption="Motor Axis 1" min=-999999.0 max=999999.0 format="%#_6f"
  in  "Position.Axis 242::99":dbl=77.0 caption="Motor Axis 1" min=-999999.0 max=999999.0 format="%#_6f"
  in  "Position.Axis 243::99":dbl=77.0 caption="Motor Axis 1" min=-999999.0 max=999999.0 format="%#_6f"
  in  "Position.Axis 231::99":dbl=77.0 caption="Motor Axis 1" min=-999999.0 max=999999.0 format="%#_6f"
  in  "Position.Axis 232::99":dbl=77.0 caption="Motor Axis 1" min=-999999.0 max=999999.0 format="%#_6f"
  in  "Position.Axis 233::99":dbl=77.0 caption="Motor Axis 1" min=-999999.0 max=999999.0 format="%#_6f"
  in  "Position.Axis 221::99":dbl=77.0 caption="Motor Axis 1" min=-999999.0 max=999999.0 format="%#_6f"
  in  "Position.Axis 222::99":dbl=77.0 caption="Motor Axis 1" min=-999999.0 max=999999.0 format="%#_6f"
  in  "Position.Axis 223::99":dbl=77.0 caption="Motor Axis 1" min=-999999.0 max=999999.0 format="%#_6f"
  in  "Position.Axis 211::99":dbl=77.0 caption="Motor Axis 1" min=-999999.0 max=999999.0 format="%#_6f"
  in  "Position.Axis 212::99":dbl=77.0 caption="Motor Axis 1" min=-999999.0 max=999999.0 format="%#_6f"
  in  "Position.Axis 213::99":dbl=77.0 caption="Motor Axis 1" min=-999999.0 max=999999.0 format="%#_6f"
  in  "Position.Axis 141::99":dbl=77.0 caption="Motor Axis 1" min=-999999.0 max=999999.0 format="%#_6f"
  in  "Position.Axis 142::99":dbl=77.0 caption="Motor Axis 1" min=-999999.0 max=999999.0 format="%#_6f"
  in  "Position.Axis 143::99":dbl=77.0 caption="Motor Axis 1" min=-999999.0 max=999999.0 format="%#_6f"
  in  "Position.Axis 131::99":dbl=77.0 caption="Motor Axis 1" min=-999999.0 max=999999.0 format="%#_6f"
  in  "Position.Axis 132::99":dbl=77.0 caption="Motor Axis 1" min=-999999.0 max=999999.0 format="%#_6f"
  in  "Position.Axis 133::99":dbl=77.0 caption="Motor Axis 1" min=-999999.0 max=999999.0 format="%#_6f"
  in  "Position.Axis 121::99":dbl=77.0 caption="Motor Axis 1" min=-999999.0 max=999999.0 format="%#_6f"
  in  "Position.Axis 122::99":dbl=77.0 caption="Motor Axis 1" min=-999999.0 max=999999.0 format="%#_6f"
  in  "Position.Axis 123::99":dbl=77.0 caption="Motor Axis 1" min=-999999.0 max=999999.0 format="%#_6f"
  in  "Position.Axis 113::99":dbl=77.0 caption="Motor Axis 1" min=-999999.0 max=999999.0 format="%#_6f"
  in  "Position.Axis 112::99":dbl=77.0 caption="Motor Axis 1" min=-999999.0 max=999999.0 format="%#_6f"
  in  "Position.Axis 111::99":dbl=77.0 caption="Motor Axis 1" min=-999999.0 max=999999.0 format="%#_6f"
  out "Arguments X":string
  in  "GUIdevice 99":string="PicoPad_LCave"
  in  "move properties":T2[](array[typedef])=[{"Tolerance [%]"=0.1, "Stepsize"=0.0001, "Invert Axis"=TRUE, "Invert Direction X"=FALSE, "Invert Direction Y"=TRUE, "enable feedback"=FALSE, "Set Centriod Target"=FALSE}, {"Tolerance [%]"=0.1, "Stepsize"=0.0001, "Invert Axis"=TRUE, "Invert Direction X"=FALSE, "Invert Direction Y"=TRUE, "enable feedback"=FALSE, "Set Centriod Target"=FALSE}, {"Tolerance [%]"=0.1, "Stepsize"=0.0001, "Invert Axis"=TRUE, "Invert Direction X"=FALSE, "Invert Direction Y"=TRUE, "enable feedback"=FALSE, "Set Centriod Target"=FALSE}, {"Tolerance [%]"=0.1, "Stepsize"=0.0001, "Invert Axis"=TRUE, "Invert Direction X"=FALSE, "Invert Direction Y"=TRUE, "enable feedback"=FALSE, "Set Centriod Target"=FALSE}, {"Tolerance [%]"=0.1, "Stepsize"=0.0001, "Invert Axis"=TRUE, "Invert Direction X"=FALSE, "Invert Direction Y"=TRUE, "enable feedback"=FALSE, "Set Centriod Target"=FALSE}, {"Tolerance [%]"=0.1, "Stepsize"=0.0001, "Invert Axis"=TRUE, "Invert Direction X"=FALSE, "Invert Direction Y"=TRUE, "enable feedback"=FALSE, "Set Centriod Target"=FALSE}, {"Tolerance [%]"=0.1, "Stepsize"=0.0001, "Invert Axis"=TRUE, "Invert Direction X"=FALSE, "Invert Direction Y"=TRUE, "enable feedback"=FALSE, "Set Centriod Target"=FALSE}, {"Tolerance [%]"=0.1, "Stepsize"=0.0001, "Invert Axis"=TRUE, "Invert Direction X"=FALSE, "Invert Direction Y"=TRUE, "enable feedback"=FALSE, "Set Centriod Target"=FALSE}, {"Tolerance [%]"=0.1, "Stepsize"=0.0001, "Invert Axis"=TRUE, "Invert Direction X"=FALSE, "Invert Direction Y"=TRUE, "enable feedback"=FALSE, "Set Centriod Target"=FALSE}, {"Tolerance [%]"=0.1, "Stepsize"=0.0001, "Invert Axis"=TRUE, "Invert Direction X"=FALSE, "Invert Direction Y"=TRUE, "enable feedback"=FALSE, "Set Centriod Target"=FALSE}, {"Tolerance [%]"=0.1, "Stepsize"=0.0001, "Invert Axis"=TRUE, "Invert Direction X"=FALSE, "Invert Direction Y"=TRUE, "enable feedback"=FALSE, "Set Centriod Target"=FALSE}, {"Tolerance [%]"=0.1, "Stepsize"=0.0001, "Invert Axis"=TRUE, "Invert Direction X"=FALSE, "Invert Direction Y"=TRUE, "enable feedback"=FALSE, "Set Centriod Target"=FALSE}, {"Tolerance [%]"=0.1, "Stepsize"=0.0001, "Invert Axis"=TRUE, "Invert Direction X"=FALSE, "Invert Direction Y"=TRUE, "enable feedback"=FALSE, "Set Centriod Target"=FALSE}]
  in  "Time":timestamp[][](array[timestamp])
  in  "Mean Size":dbl[][](array[numeric])
  in  "Size":dbl[][](array[numeric])
  in  "active CCDs":i32(listbox)=1
  in  "Offset Y":dbl[][](array[numeric])
  in  "Offset X":dbl[][](array[numeric])
  in  "Mean Centroid X":dbl[][](array[numeric])
  in  "Mean Centroid Y":dbl[][](array[numeric])
  in  "Centroid Y":dbl[][](array[numeric])
  in  "Centroid X":dbl[][](array[numeric])
  in  "GUIdevice 7":string
  in  "GUIdevice 6":string
  in  "GUIdevice 5":string
  in  "GUIdevice 4":string
  in  "GUIdevice 3":string
  in  "GUIdevice 2":string="BellaCam46_2_Scatter_In_1"
  in  "insert tag":bool=TRUE
  in  "stop":bool
  in  "GUIdevice 1":string="BellaCam32_3"
  out "tcp data event":T13
  out "error IO 2":errorcluster
  # "x [Tolerance]"
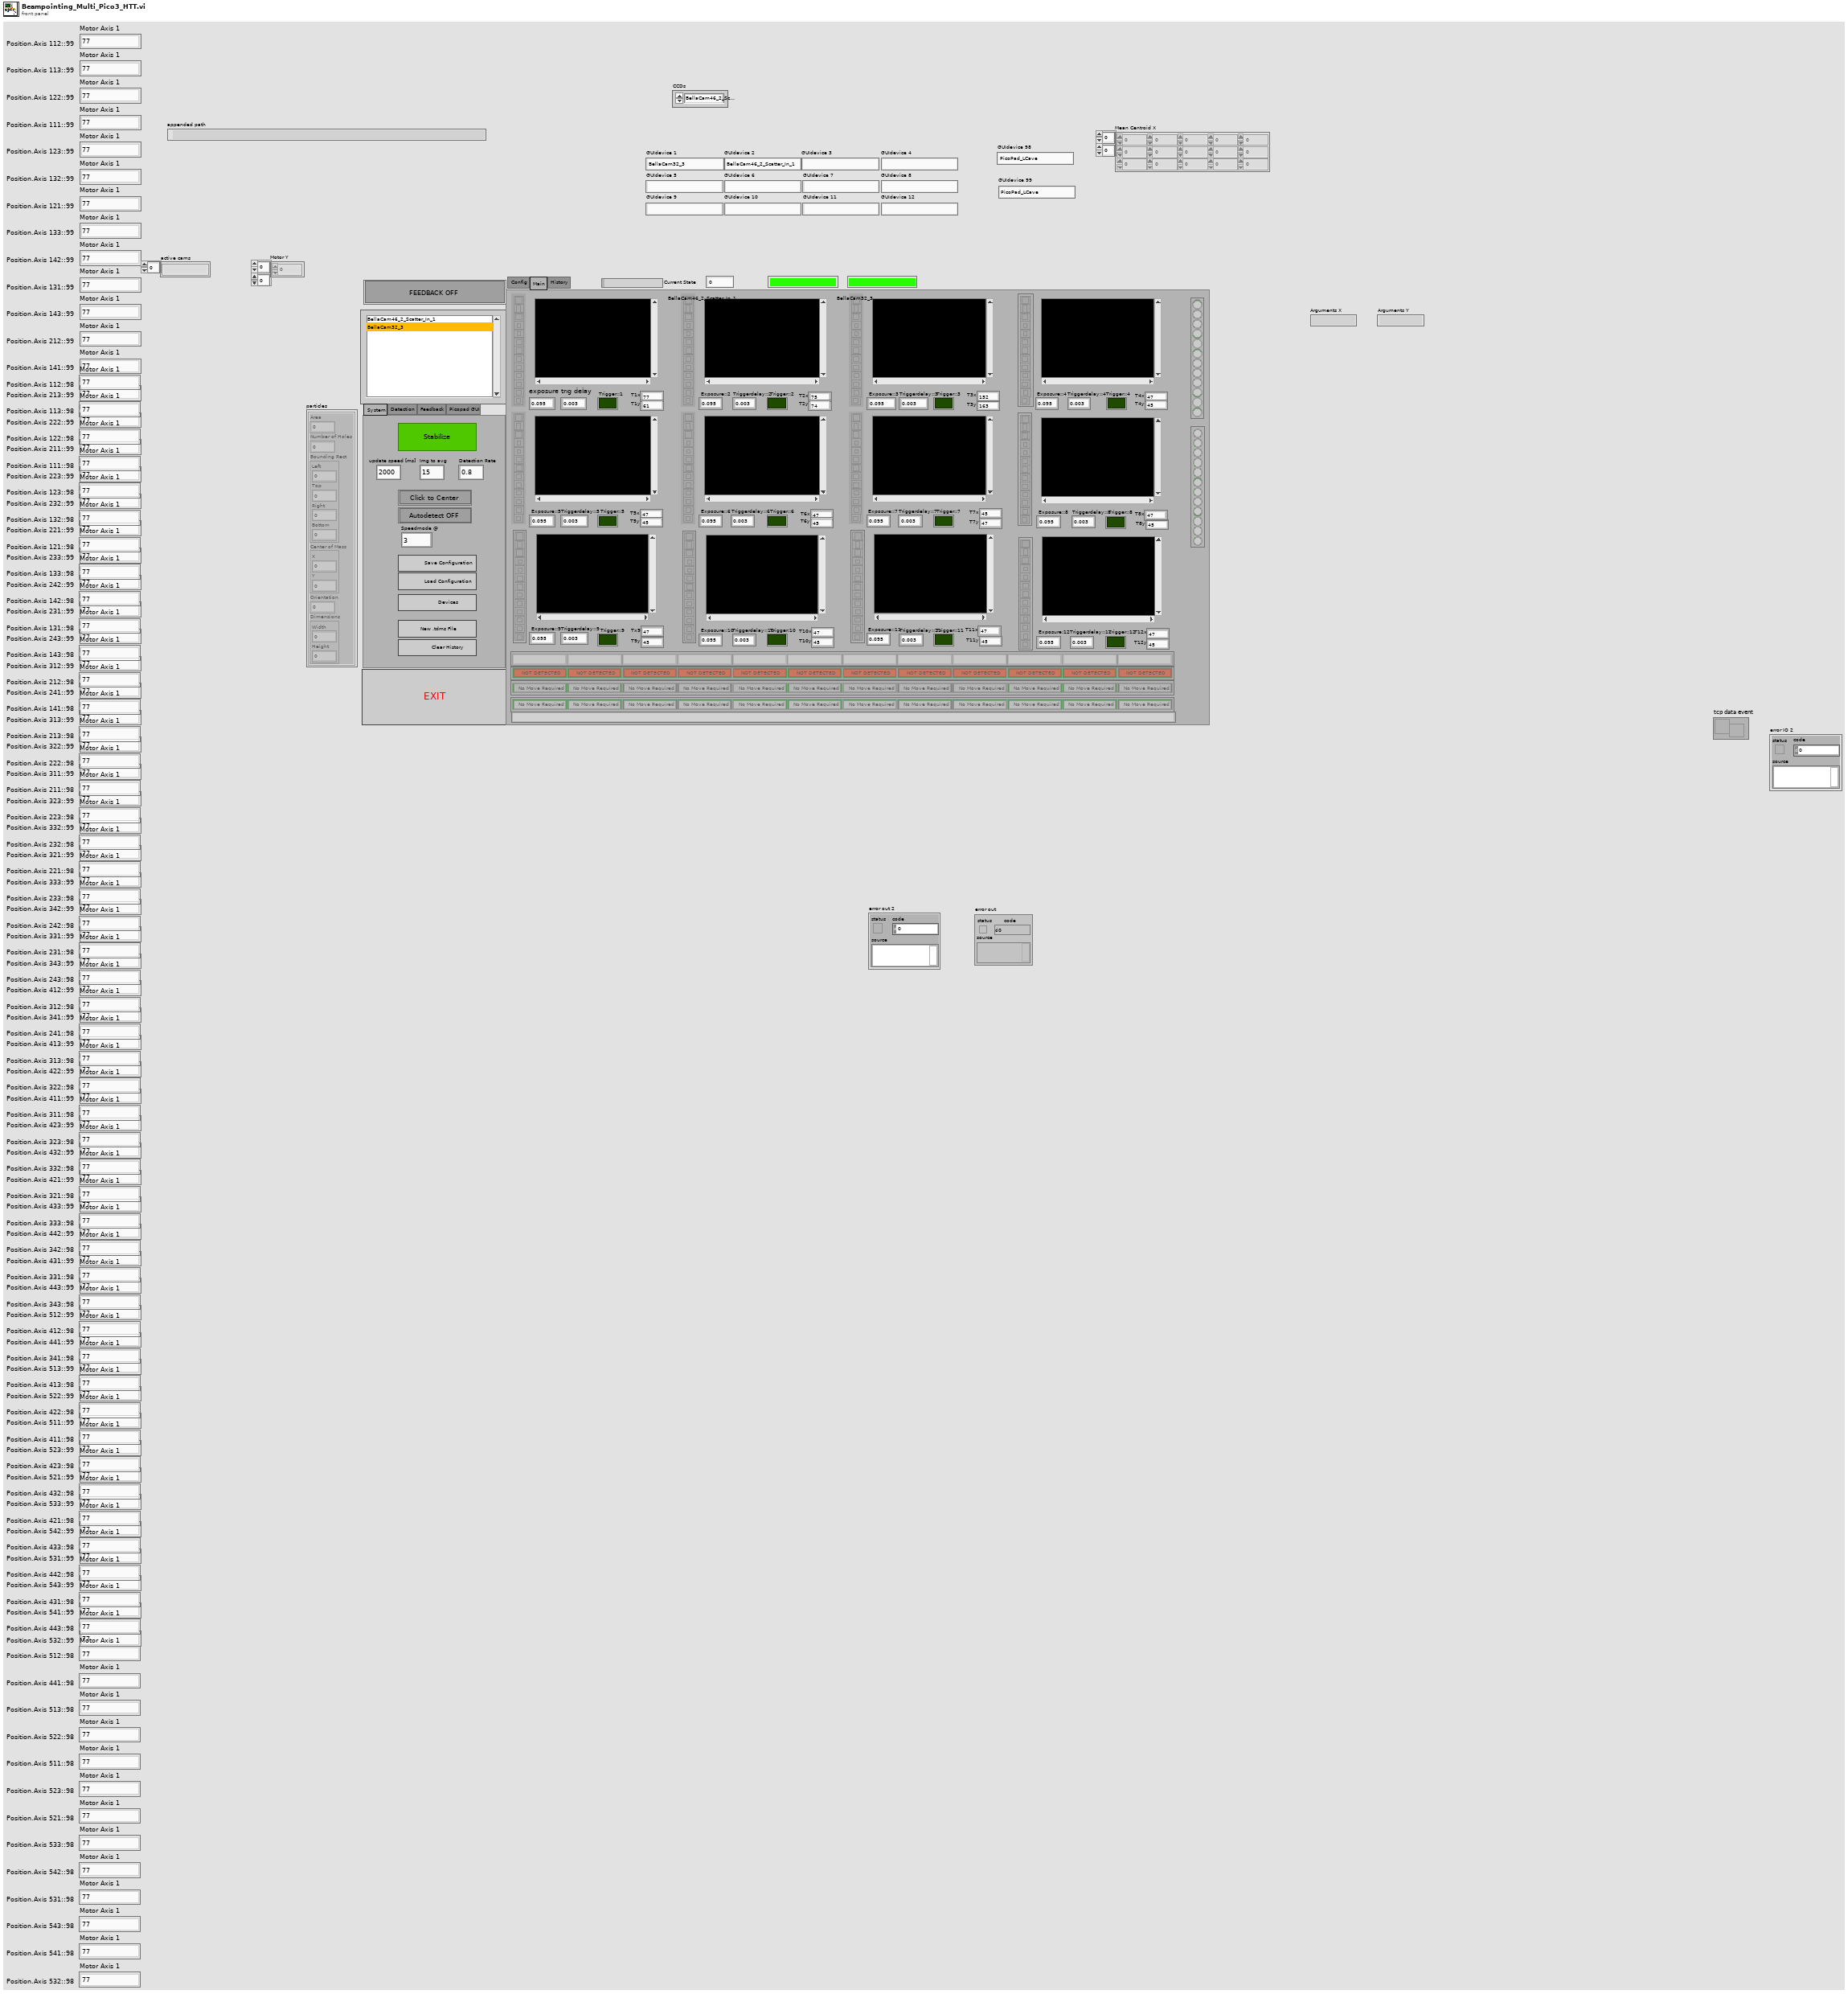
[diagram p1: front panel]
types:
  T1 = cluster{"Area":dbl, "Number of Holes":dbl, "Bounding Rect":cluster{"Left":dbl, "Top":dbl, "Right":dbl, "Bottom":dbl}, "Center of Mass":cluster{"X":dbl, "Y":dbl}, "Orientation":dbl, "Dimensions":cluster{"Width":dbl, "Height":dbl}}[]
  T2 = typedef "move.ctl" = cluster{"Tolerance [%]":dbl, "Stepsize":dbl, "Invert Axis":bool, "Invert Direction X":bool, "Invert Direction Y":bool, "enable feedback":bool, "Set Centriod Target":bool}
  T3 = typedef "beam detection.ctl" = cluster{"Filter":u16, "Filter Para":cluster{"X Size":i32, "Y Size":i32, "% Tolerance":i32}, "detection method":i32, "smal para":cluster{"Measurement Parameter":T4, "Range Lower Value":dbl, "Range Upper Value":dbl, "Range":bool, "Measurement Type":bool}[], "Remove small Objects":bool, "Restrict to round Objects":bool}
  T4 = typedef "Particle Parameters" = i32
  T5 = cluster{"CCDs":string[], "move properties":T2[], "detection para":T3[], "thresholds":cluster{"Lower value":sgl, "Upper value":sgl}[], "Value":cluster{"Motor CCD 1":u16, "Motor CCD 2":u16, "Motor CCD 3":u16, "Motor CCD 4":u16, "Motor CCD 5":u16, "Motor CCD 6":u16, "Motor CCD 7":u16, "Motor CCD 8":u16, "Motor CCD 9":u16, "Motor CCD 10":u16, "Motor CCD 11":u16, "Motor CCD 12":u16}}
  T6 = cluster{"Left":dbl, "Top":dbl, "Right":dbl, "Bottom":dbl}[]
  T7 = cluster{"Motor CCD 1":u16, "Motor CCD 2":u16, "Motor CCD 3":u16, "Motor CCD 4":u16, "Motor CCD 5":u16, "Motor CCD 6":u16, "Motor CCD 7":u16, "Motor CCD 8":u16, "Motor CCD 9":u16, "Motor CCD 10":u16, "Motor CCD 11":u16, "Motor CCD 12":u16}
  T8 = cluster{"[0]":string, "[1]":string, "[2]":string, "[3]":string, "[4]":string, "[5]":string, "[6]":string, "[7]":string, "[8]":string, "[8] 2":string, "[8] 3":string, "[8] 4":string}
  T9 = typedef "IMAQ Image.ctl" = refnum<image>
  T10 = cluster{"Area":dbl, "Number of Holes":dbl, "Bounding Rect":cluster{"Left":dbl, "Top":dbl, "Right":dbl, "Bottom":dbl}, "Center of Mass":cluster{"X":dbl, "Y":dbl}, "Orientation":dbl, "Dimensions":cluster{"Width":dbl, "Height":dbl}}[][]
  T11 = enum32{"System", "Detection", "Feedback", "Picopad GUI"}
  T12 = cluster{"Ref X":refnum<vi>, "Ref Y":refnum<vi>}[]
  T13 = typedef "tcp_new_data_event.ctl" = refnum<user-event>
  T14 = typedef "Crosshair type def.ctl" = cluster{"Draw":bool, "Target":cluster{"x":dbl, "y":dbl}, "Size":cluster{"x":dbl, "y":dbl}, "Angle":dbl, "Color":u32, "Thickness":u8, "CrosshairLabel":string}
  T15 = typedef "tcp new data cluster.ctl" = cluster{"EventEnum":enum16{"new data", "connection status update"}, "Device name":string}
  T16 = cluster{"Left":i32, "Top":i32, "Right":i32, "Bottom":i32}
  T17 = enum32{"invalid app kind", "Development System", "Run Time System", "Student Edition", "Embedded LabVIEW", "Evaluation", "Custom"}
  T18 = enum16{"open", "open or create", "create or replace", "create", "open (read-only)"}
  T19 = enum32{"Invalid", "Standard", "Closed", "Hidden", "Minimized", "Maximized"}
  T20 = enum16{"open", "replace", "create", "open or create", "replace or create", "replace or create with confirmation"}
  T21 = typedef "Image Type" = u32
  T22 = cluster{"[0]":string, "[1]":string, "[2]":string, "[3]":string, "[4]":string, "[5]":string, "[6]":string, "[7]":string, "[8]":string, "[9]":string, "[10]":string, "[11]":string}
  T23 = cluster{"Target.X::1":refnum<vi>, "Target.Y::1":refnum<vi>}
  T24 = cluster{"Target.X::2":refnum<vi>, "Target.Y::2":refnum<vi>}
  T25 = cluster{"Target.X::3":refnum<vi>, "Target.Y::3":refnum<vi>}
  T26 = cluster{"Target.X::4":refnum<vi>, "Target.Y::4":refnum<vi>}
  T27 = cluster{"Target.X::5":refnum<vi>, "Target.Y::5":refnum<vi>}
  T28 = cluster{"Target.X::6":refnum<vi>, "Target.Y::6":refnum<vi>}
  T29 = cluster{"Target.X::7":refnum<vi>, "Target.Y::7":refnum<vi>}
  T30 = cluster{"Target.X::8":refnum<vi>, "Target.Y::8":refnum<vi>}
  T31 = cluster{"Target.X::12":refnum<vi>, "Target.Y::12":refnum<vi>}
  T32 = cluster{"Target.X::9":refnum<vi>, "Target.Y::9":refnum<vi>}
  T33 = cluster{"Target.X::10":refnum<vi>, "Target.Y::10":refnum<vi>}
  T34 = cluster{"Target.X::11":refnum<vi>, "Target.Y::11":refnum<vi>}
  T35 = cluster{"Target.X::12":refnum<vi>, "Target.Y::12":refnum<vi>}[]
  T36 = cluster{"Left":dbl, "Top":dbl, "Right":dbl, "Bottom":dbl}
  T37 = cluster{"Core":cluster{"Current VI Reference":refnum<vi>, "Close Panel on Exit?":bool}, "detection para":T3[], "thresholds":cluster{"Lower value":sgl, "Upper value":sgl}[], "Centroid X":dbl[][], "Centroid Y":dbl[][], "img to avg":i32, "Mean Centroid X":dbl[][], "Mean Centroid Y":dbl[][], "Offset X":dbl[][], "Offset Y":dbl[][], "Offset X stats ":dbl[][], "Offset Y stats ":dbl[][], "Size":dbl[][], "Mean Size":dbl[][], "Time":timestamp[][], "move properties":T2[], "active axis refs 2":cluster{"Ref X":refnum<vi>, "Ref Y":refnum<vi>}[], "active ccd":i32, "Feedback global":bool, "Motor X":dbl[][], "Motor Y":dbl[][], "active cams":string[], "Data Value Reference out":refnum<k34>, "detected":bool[], "speedmode X":bool[], "speedmode Y":bool[]}
  T38 = typedef "DialogType.ctl" = u16
  T39 = cluster{"Current VI Reference":refnum<vi>, "Close Panel on Exit?":bool}
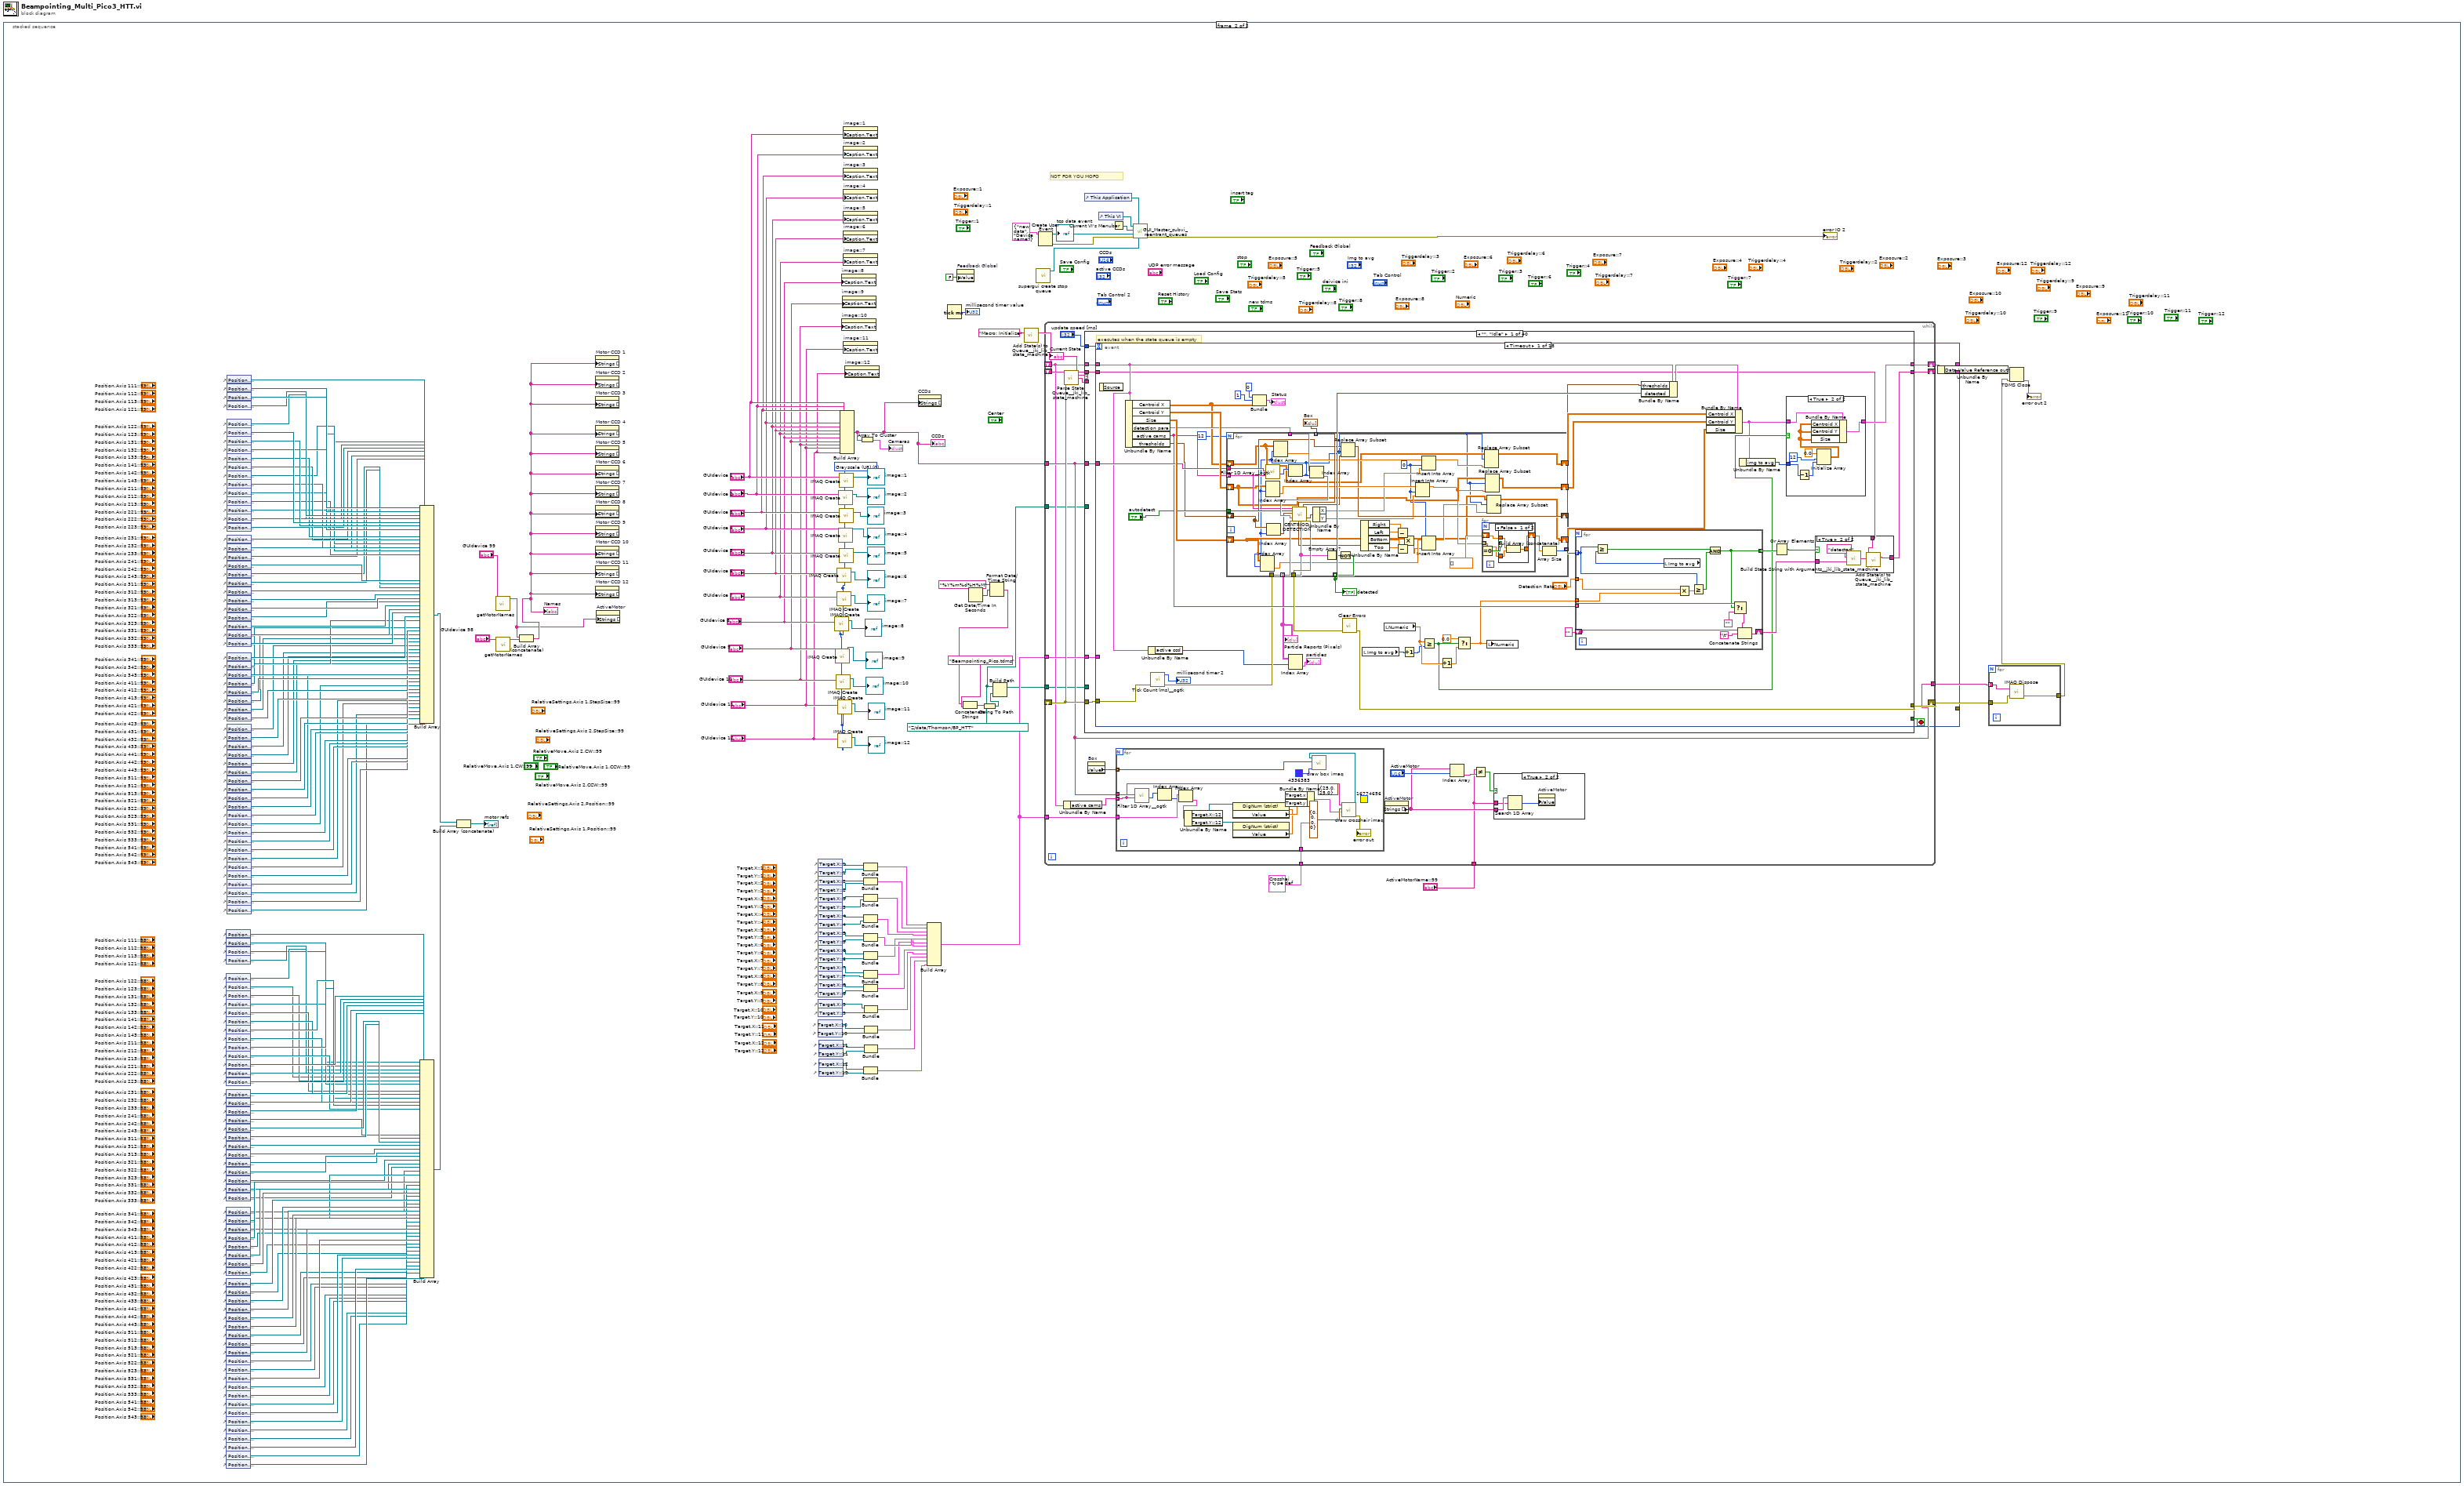
[diagram p0: block diagram]
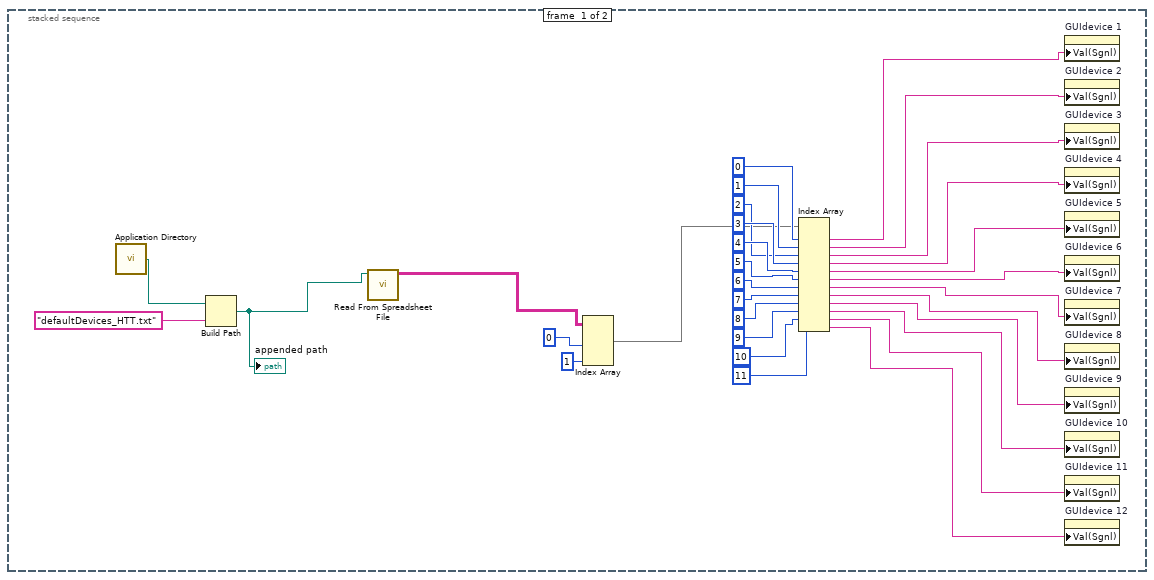
[diagram p2: hidden frame]
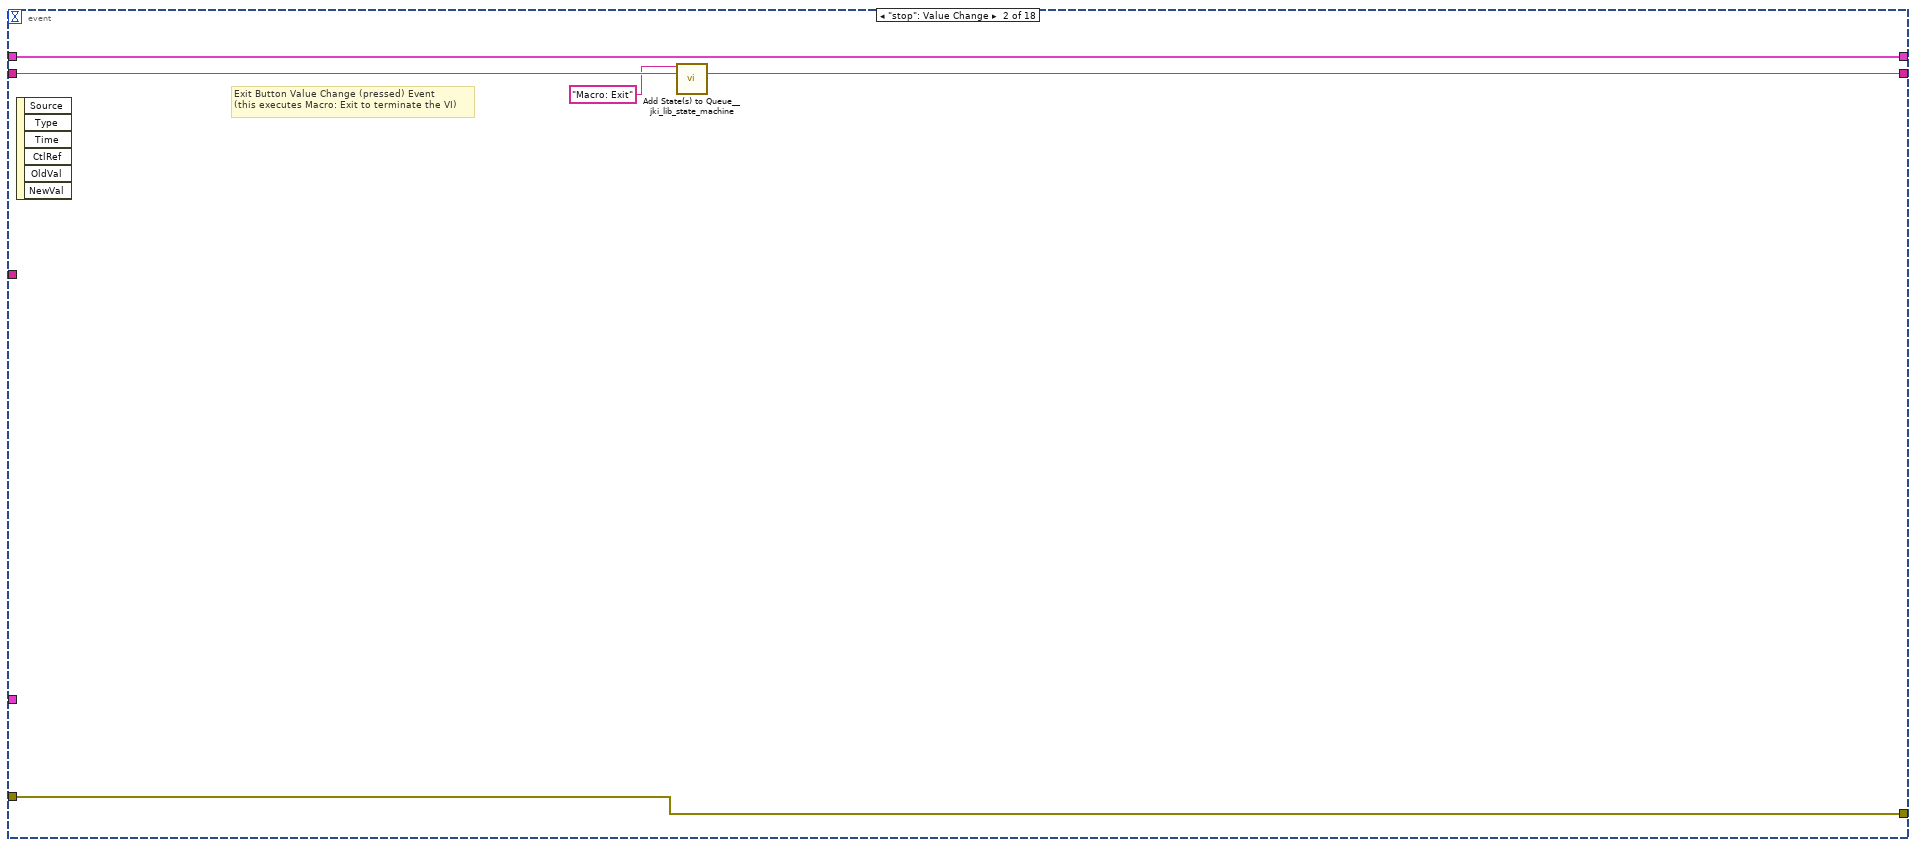
[diagram p7: hidden frame]
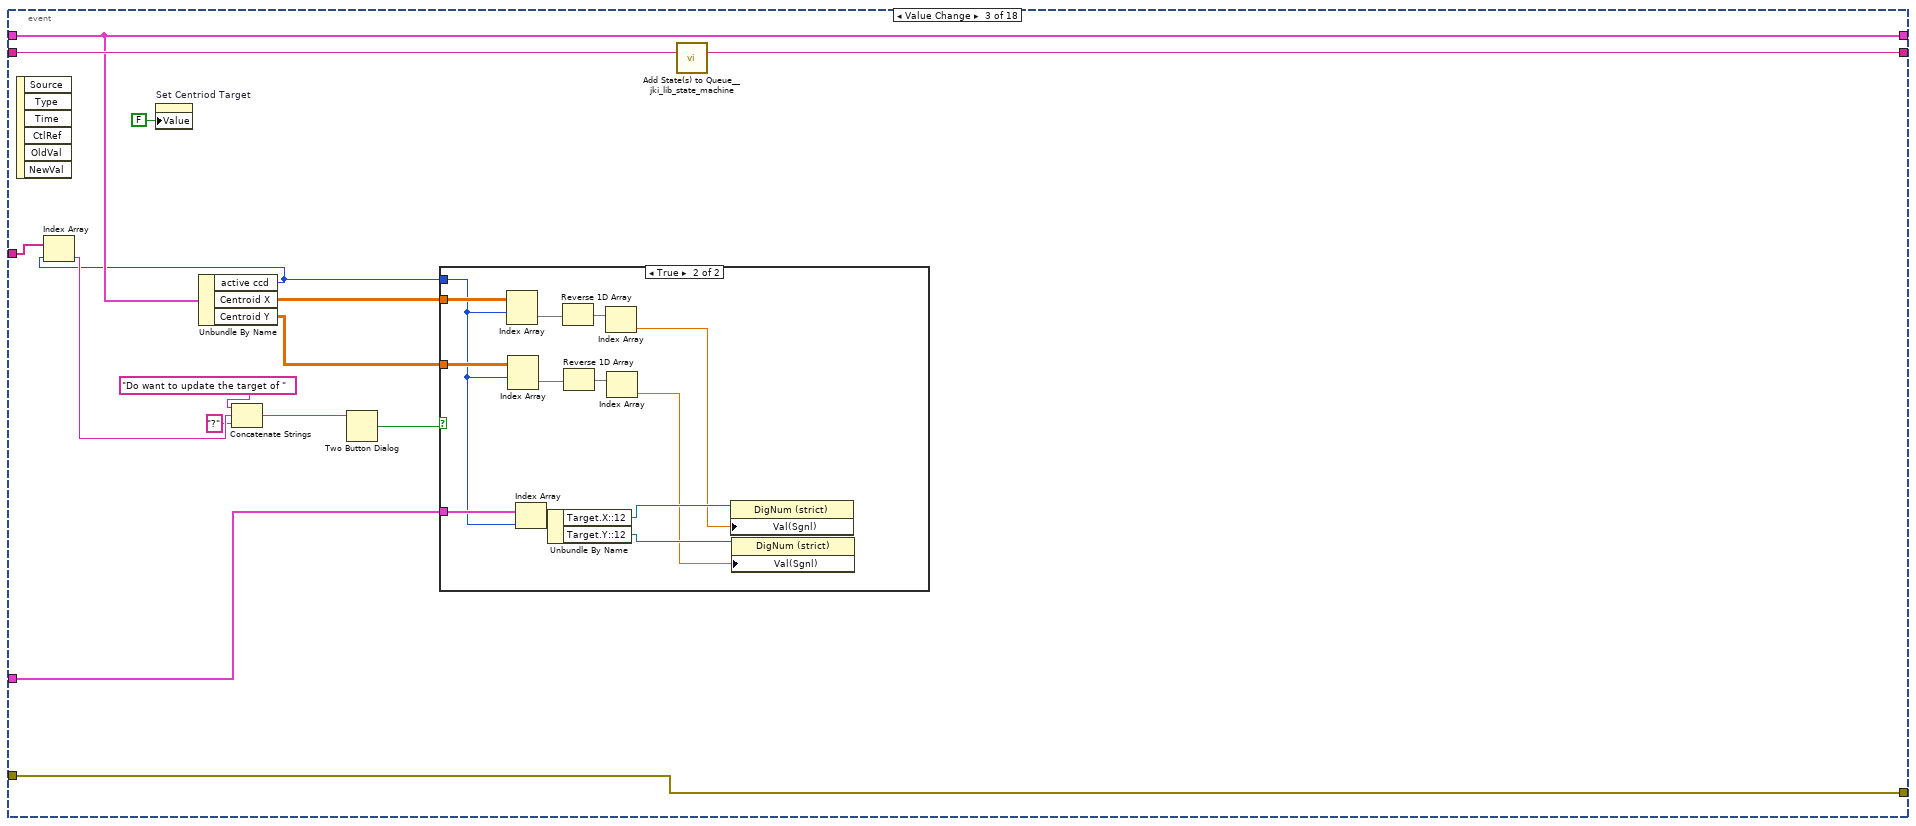
[diagram p8: hidden frame]
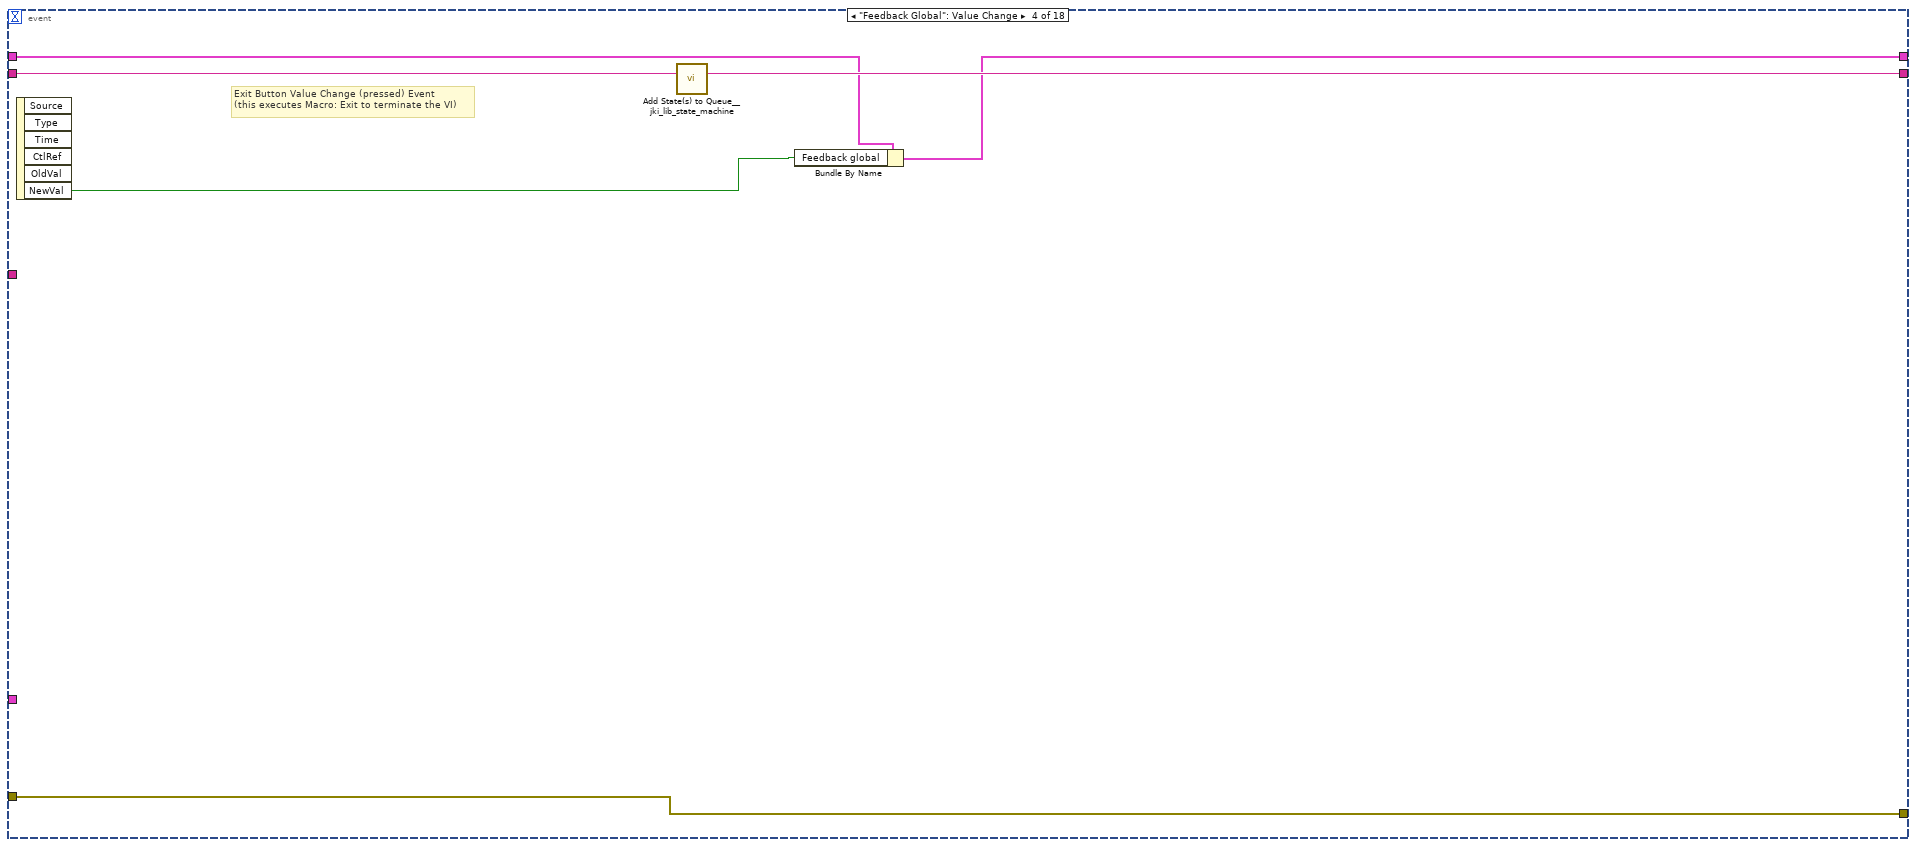
[diagram p10: hidden frame]
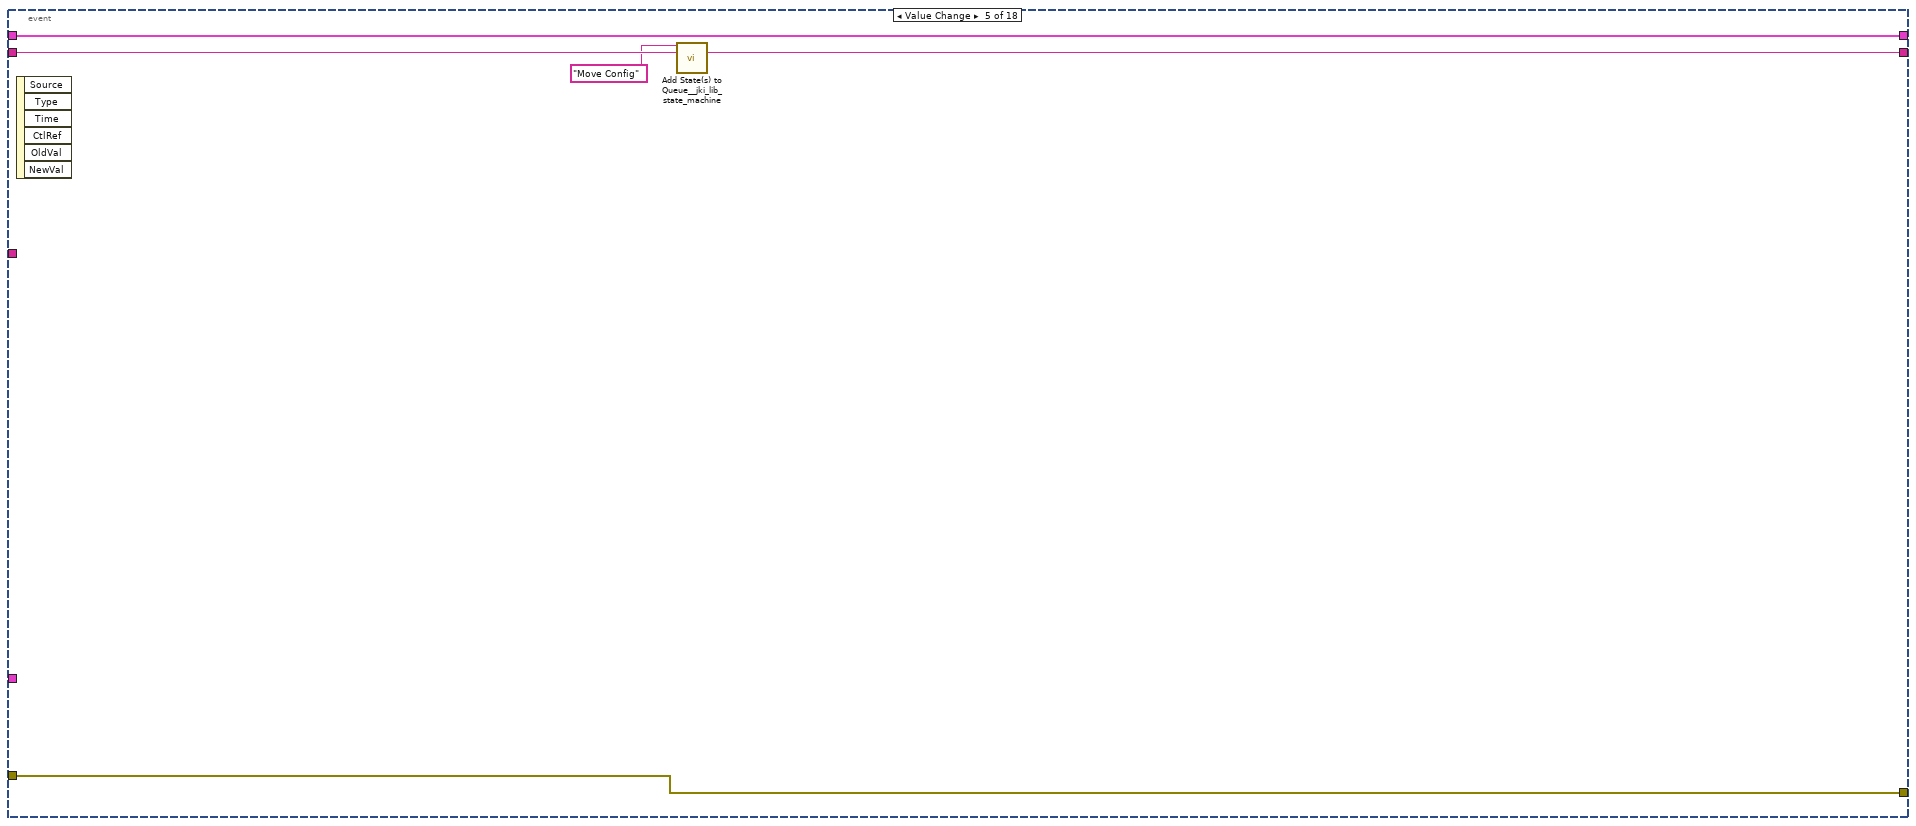
[diagram p11: hidden frame]
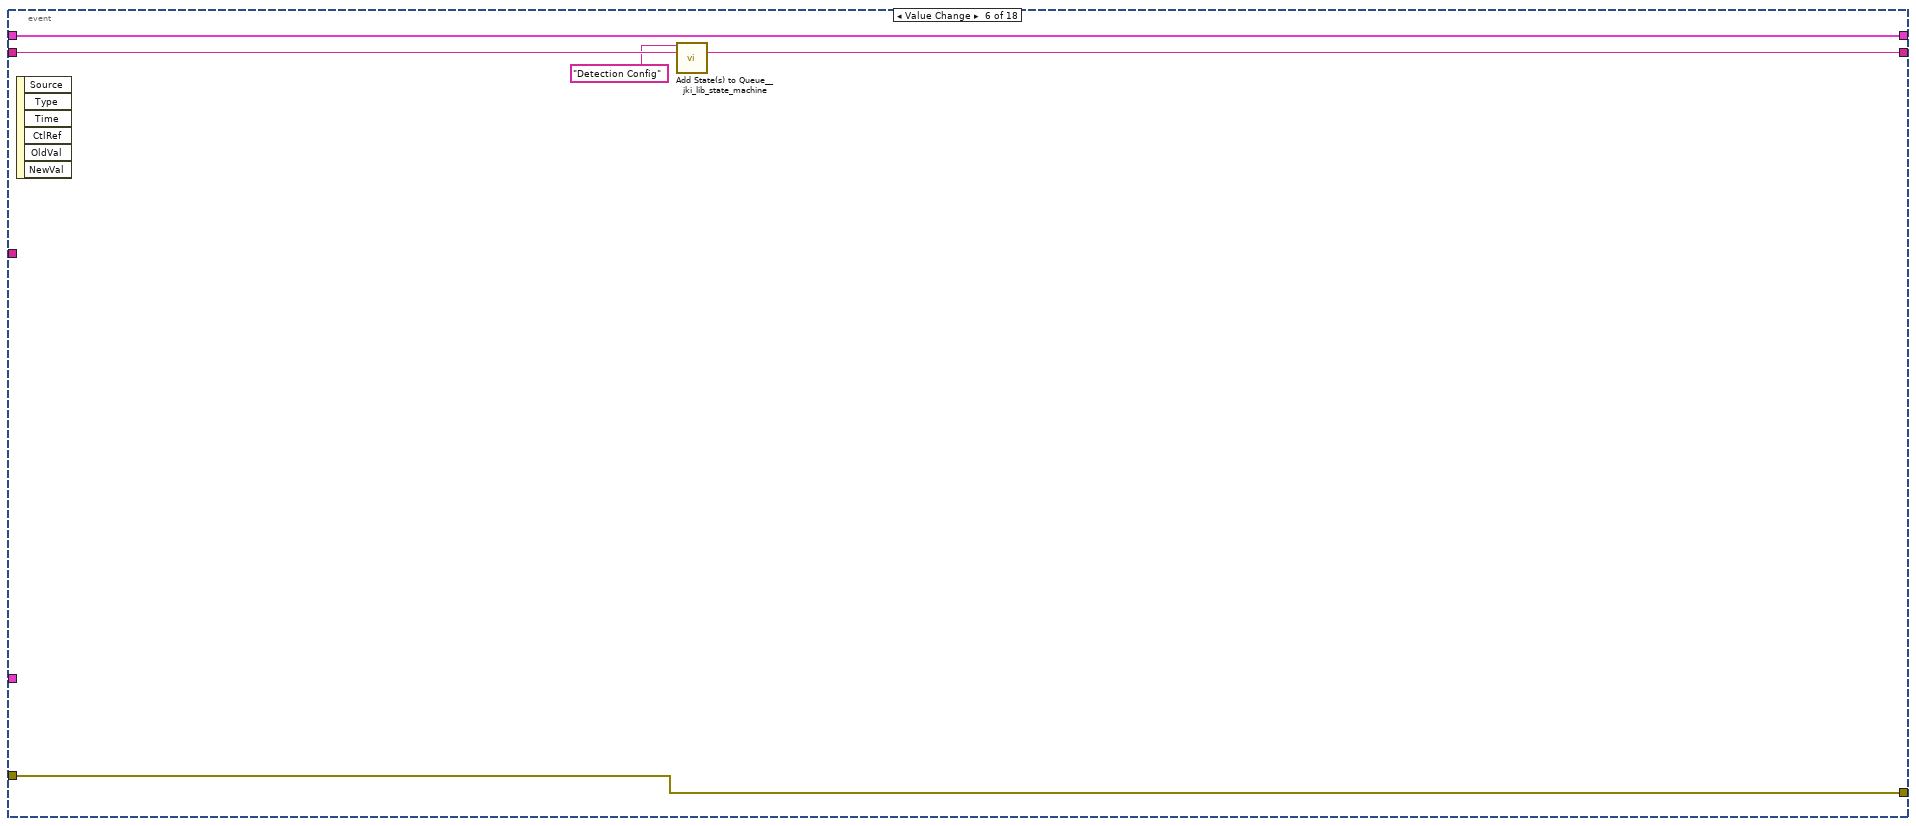
[diagram p12: hidden frame]
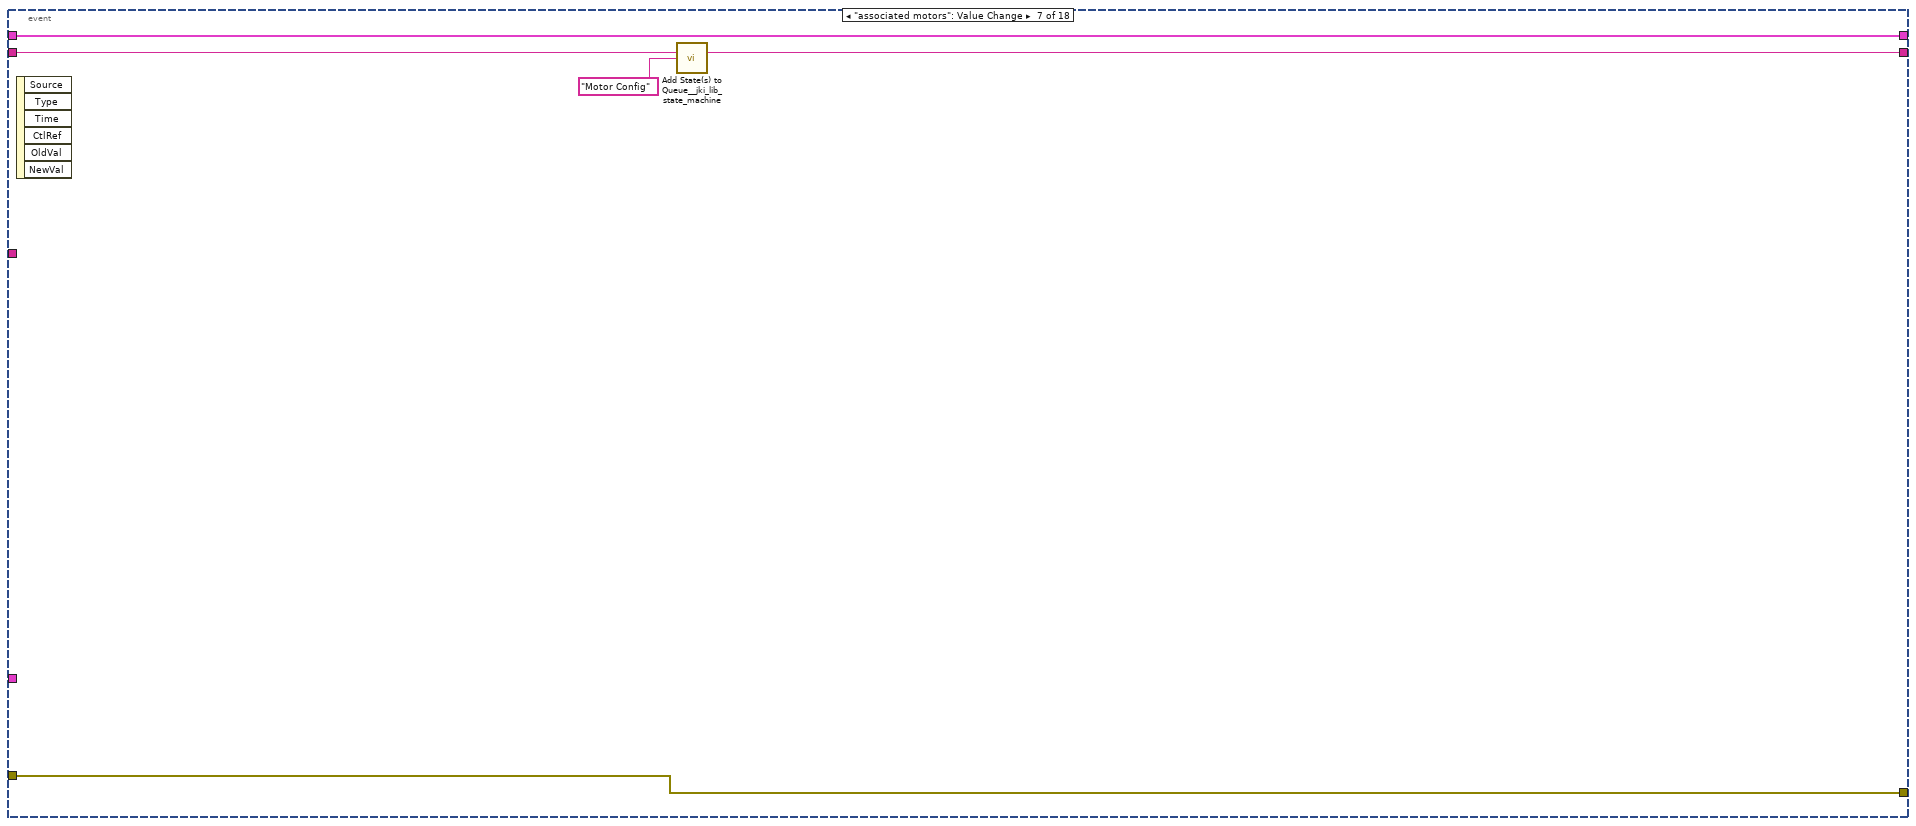
[diagram p13: hidden frame]
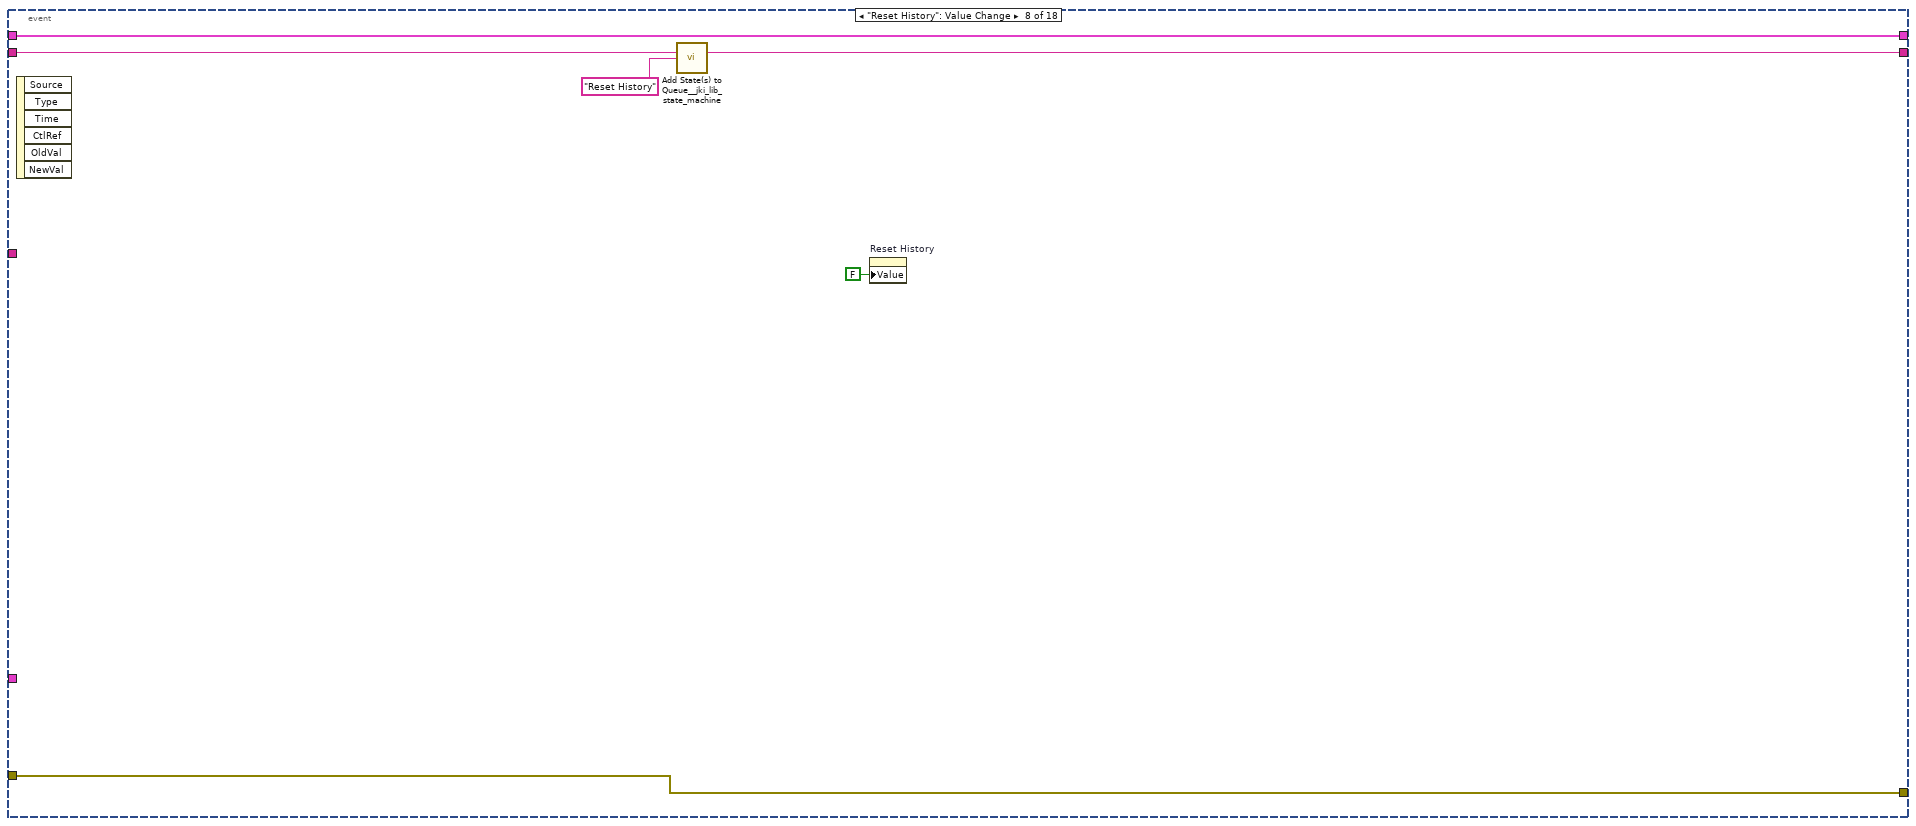
[diagram p14: hidden frame]
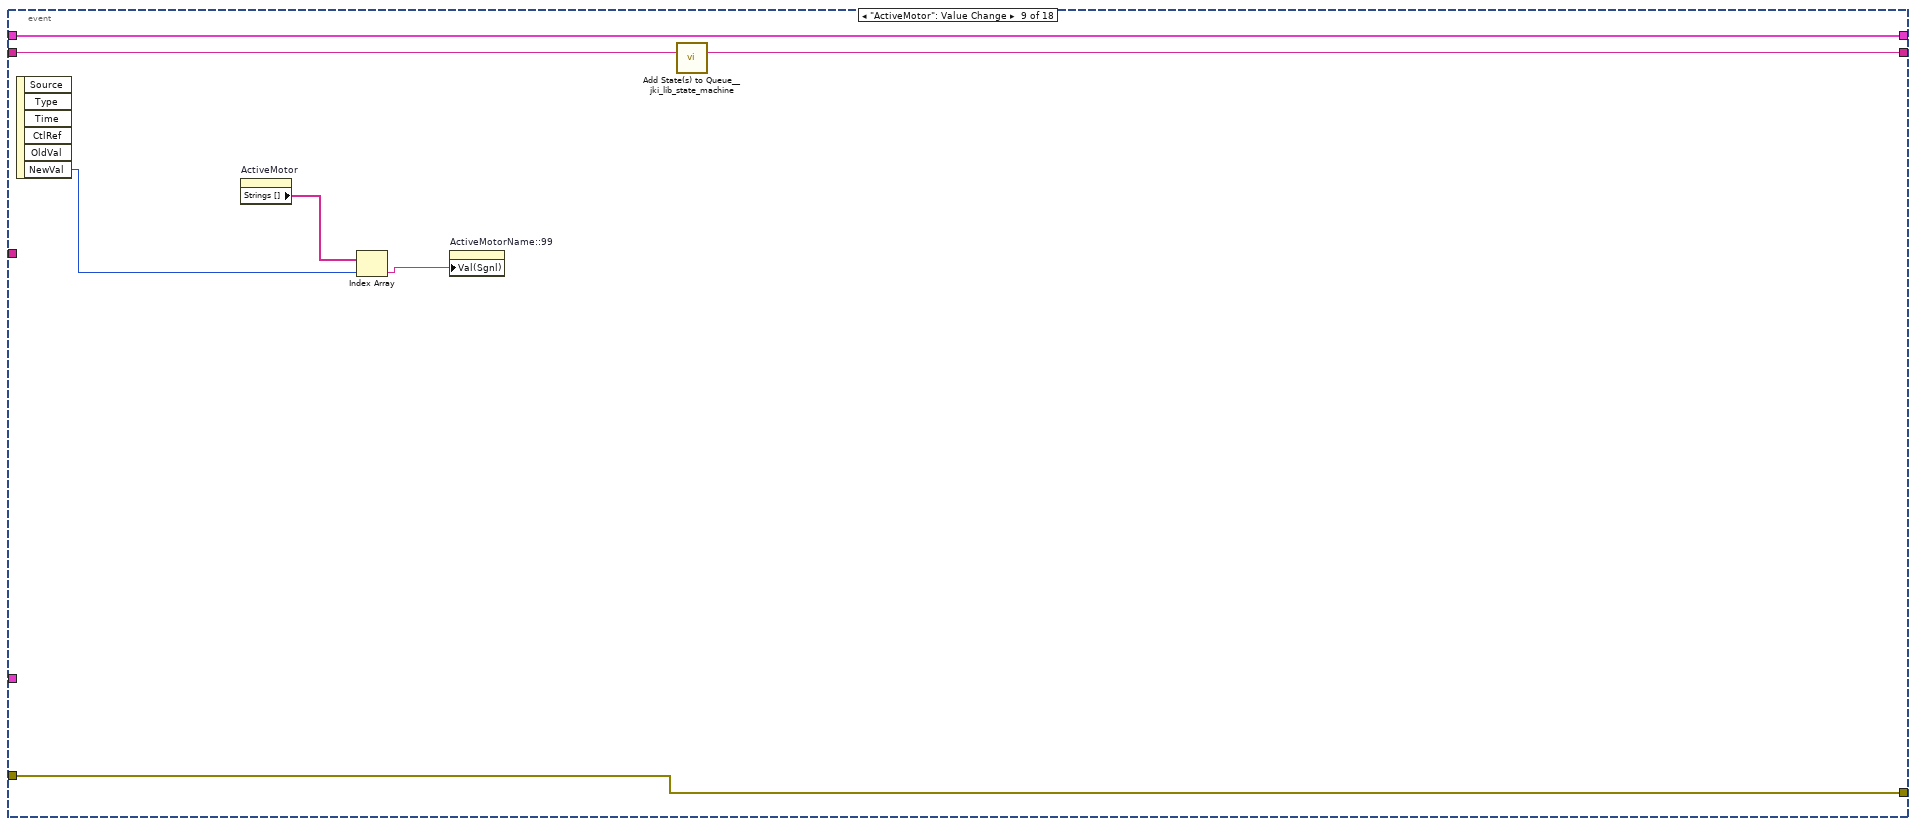
[diagram p15: hidden frame]
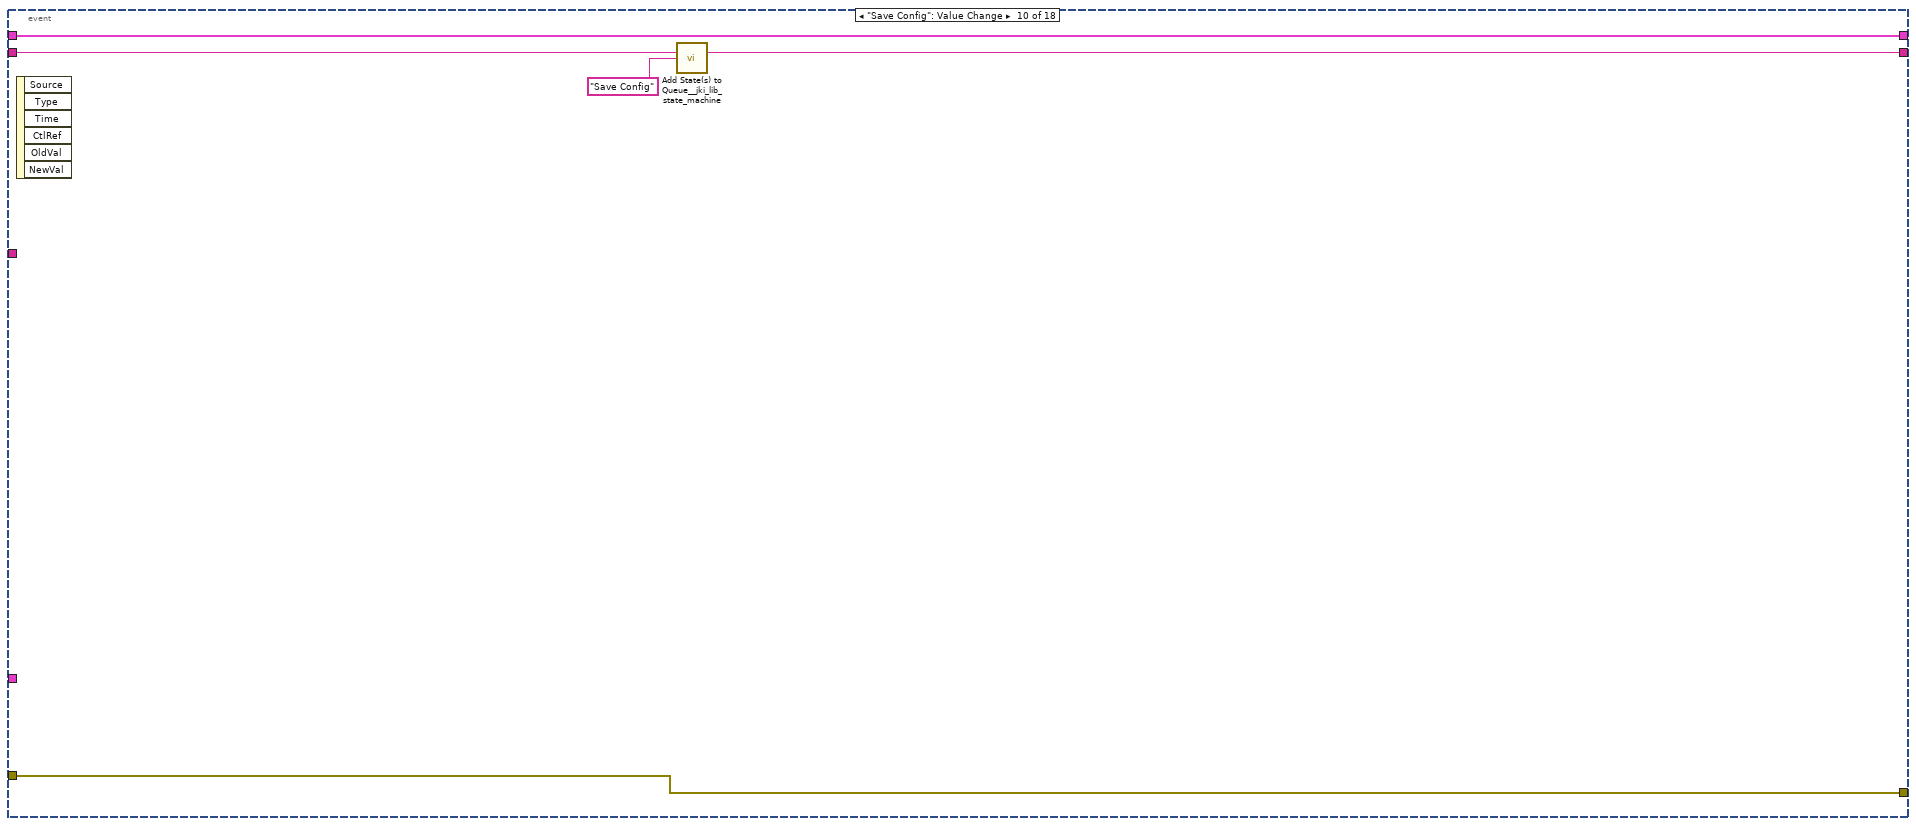
[diagram p16: hidden frame]
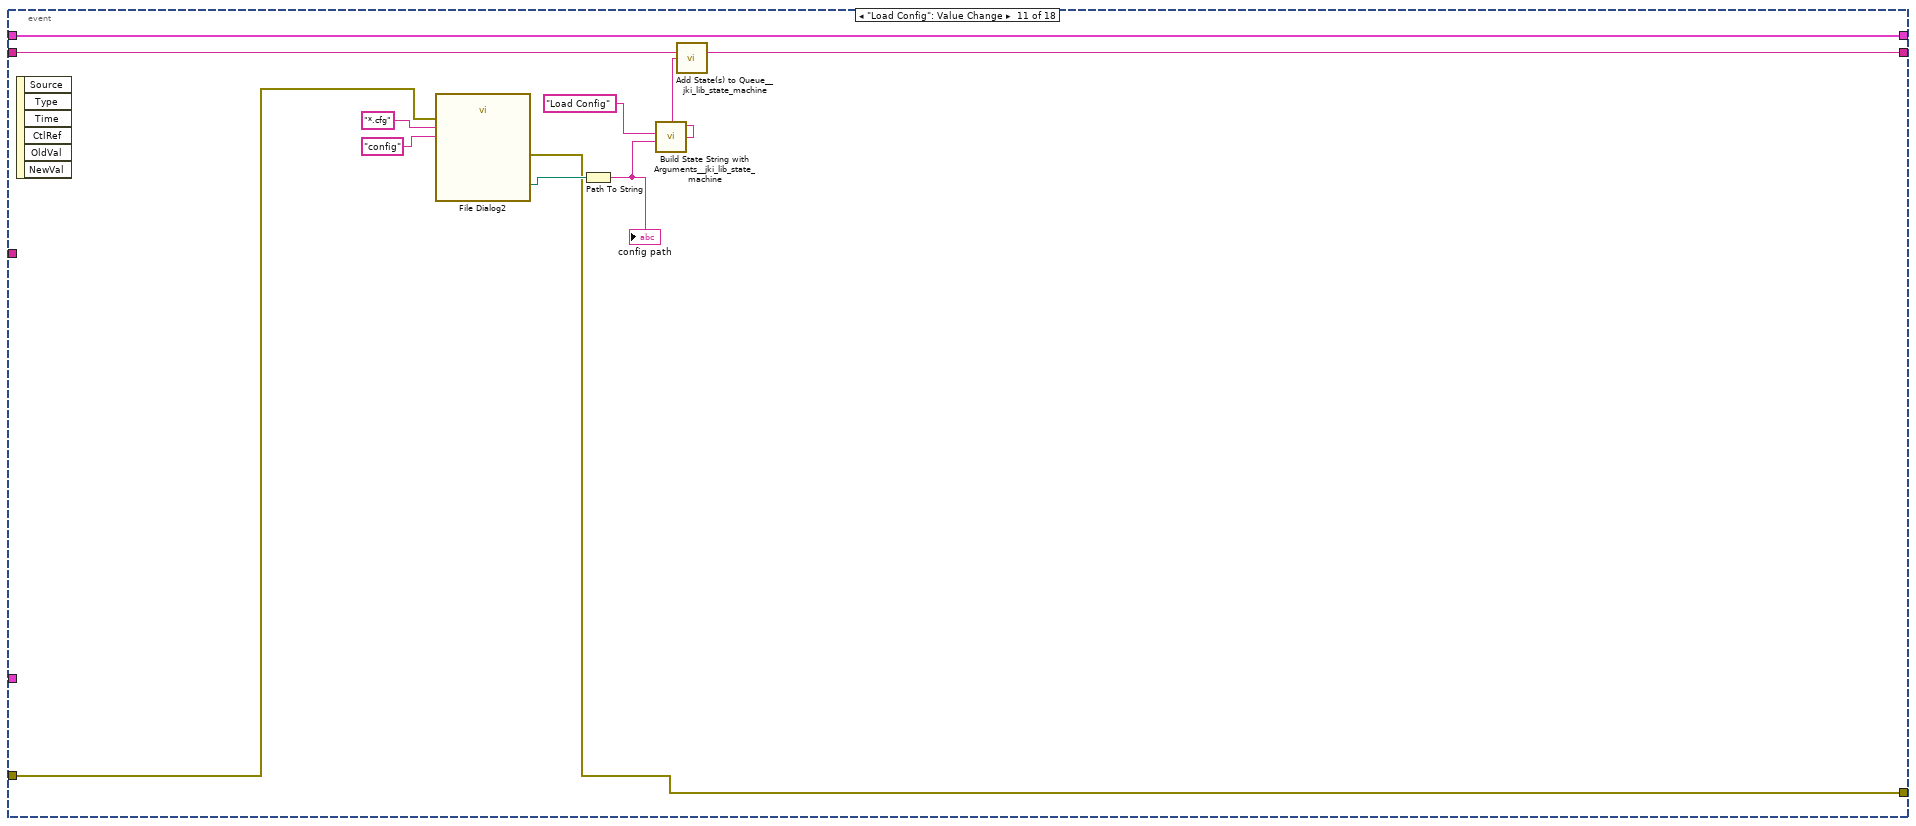
[diagram p17: hidden frame]
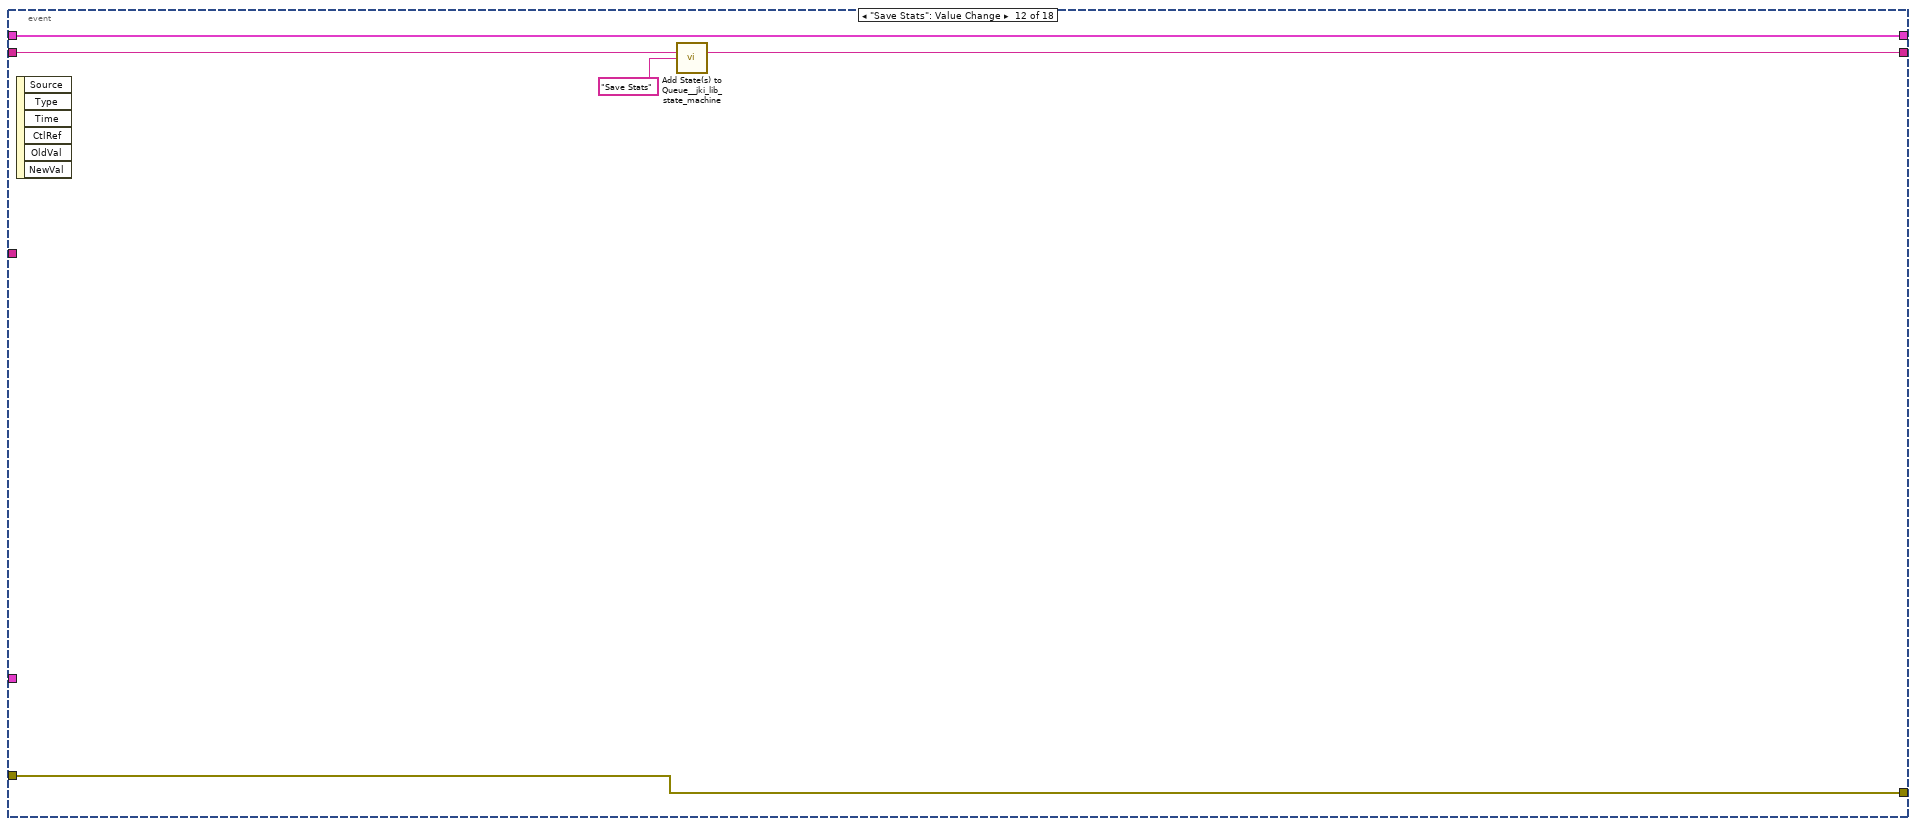
[diagram p18: hidden frame]
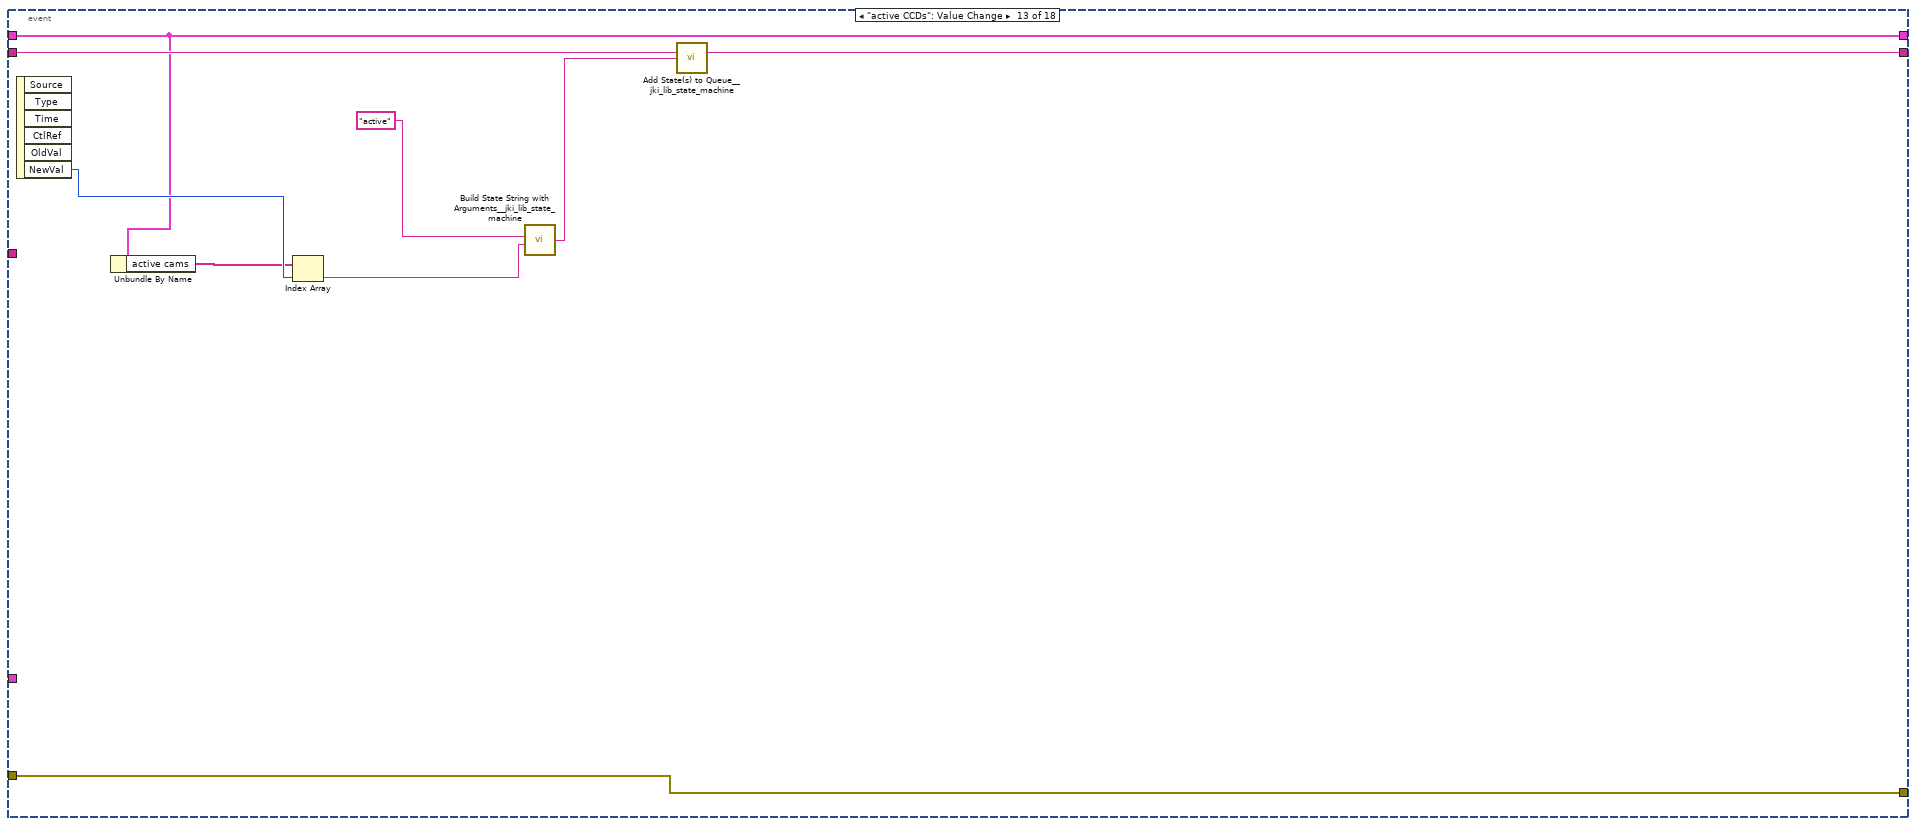
[diagram p19: hidden frame]
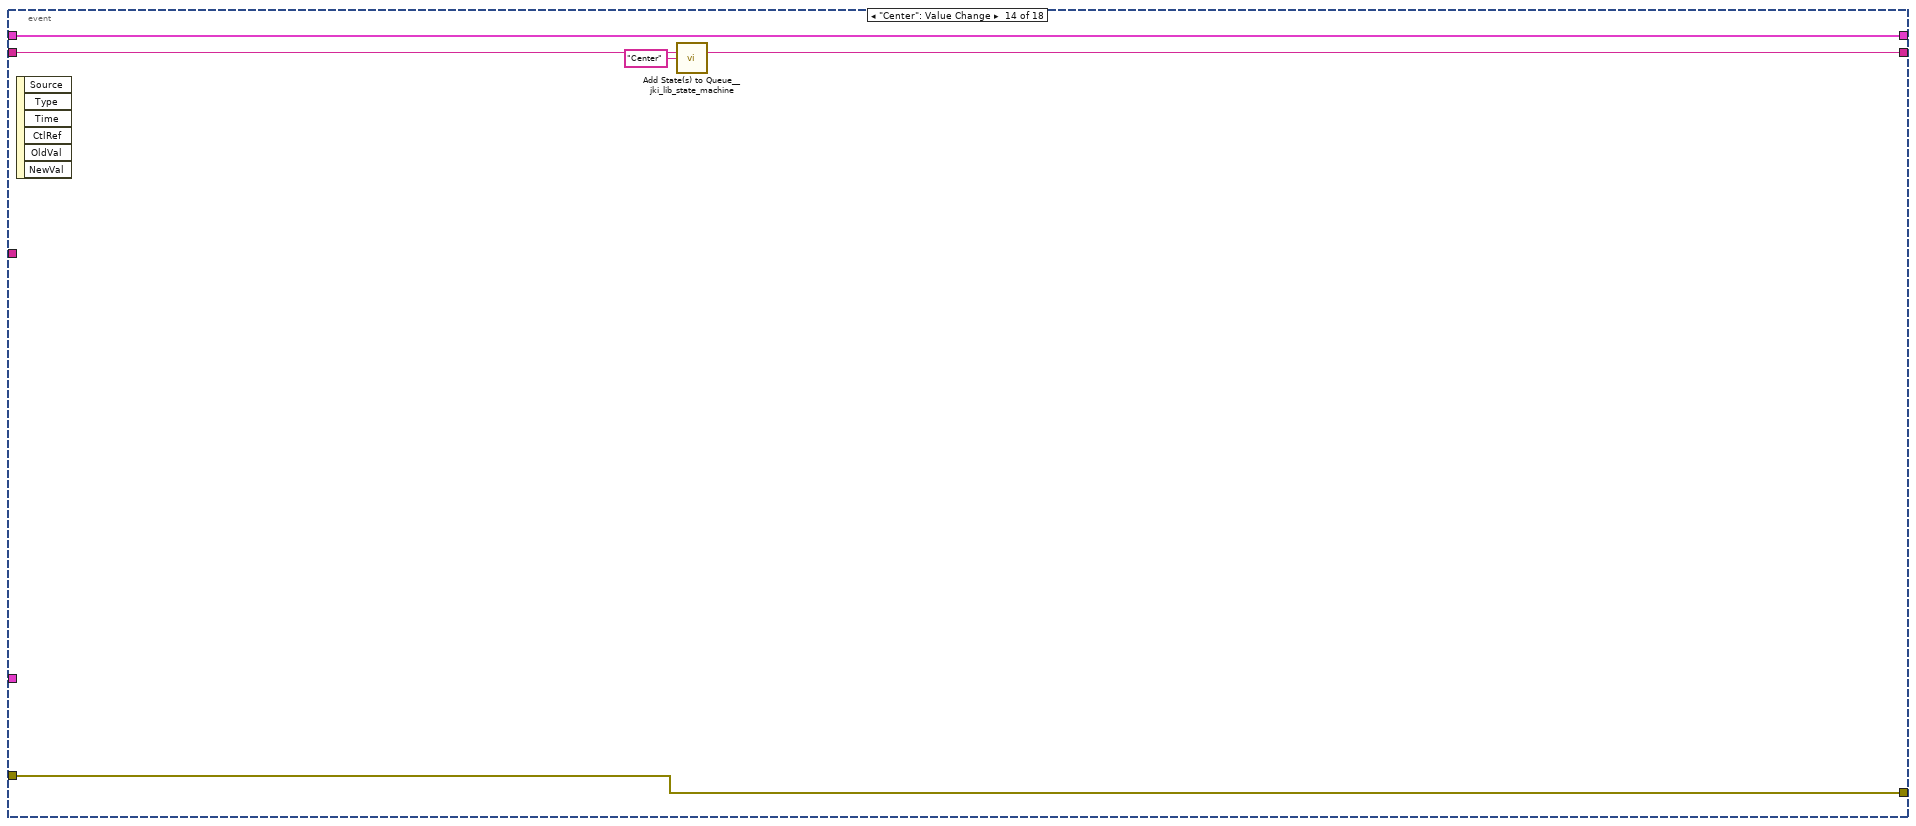
[diagram p20: hidden frame]
diagram:
  n1 = stacked-sequence {
    frame #0 {
      n2 = call <vilib>:"Application Directory.vi"() -> ("Application Directory"=w13:path)
      n3 = Build Path(base path=w13, name or relative path="defaultDevices_HTT.txt") -> (appended path=w15:path)
      "appended path" <- w15
      n4 = call-poly <vilib>:"Read From Spreadsheet File.vi"("file path (dialog if empty)"=w15) -> ("all rows"=w16:string[][])  [unwired: 6 in, 4 out]
      n5 = Index Array(array=w16, index (col) #1=0 ("disabled index (col)"), index (col) #2=1 ("index (col)")) -> (element #1=w19:string[])  [unwired: 2 in, 1 out]
      n6 = Index Array(array=w19, index #1=0 ("index"), index #2=1 ("index"), index #3=2 ("index"), index #4=3 ("index"), index #5=4 ("index"), index #6=5 ("index"), index #7=6 ("index"), index #8=7 ("index"), index #9=8 ("index"), index #10=9 ("index"), index #11=10 ("index"), index #12=11 ("index")) -> (element #1=w12:string, element #2=w11:string, element #3=w10:string, element #4=w9:string, element #5=w8:string, element #6=w7:string, element #7=w6:string, element #8=w5:string, element #9=w4:string, element #10=w3:string, element #11=w2:string, element #12=w1:string)
      n7 = property on="GUIdevice 1" class="Str"("Val(Sgnl)"=w12) -> ()  [unwired: 2 in, 2 out]
      n8 = property on="GUIdevice 2" class="Str"("Val(Sgnl)"=w11) -> ()  [unwired: 2 in, 2 out]
      n9 = property on="GUIdevice 3" class="Str"("Val(Sgnl)"=w10) -> ()  [unwired: 2 in, 2 out]
      n10 = property on="GUIdevice 4" class="Str"("Val(Sgnl)"=w9) -> ()  [unwired: 2 in, 2 out]
      n11 = property on="GUIdevice 5" class="Str"("Val(Sgnl)"=w8) -> ()  [unwired: 2 in, 2 out]
      n12 = property on="GUIdevice 6" class="Str"("Val(Sgnl)"=w7) -> ()  [unwired: 2 in, 2 out]
      n13 = property on="GUIdevice 7" class="Str"("Val(Sgnl)"=w6) -> ()  [unwired: 2 in, 2 out]
      n14 = property on="GUIdevice 8" class="Str"("Val(Sgnl)"=w5) -> ()  [unwired: 2 in, 2 out]
      n15 = property on="GUIdevice 9" class="Str"("Val(Sgnl)"=w4) -> ()  [unwired: 2 in, 2 out]
      n16 = property on="GUIdevice 10" class="Str"("Val(Sgnl)"=w3) -> ()  [unwired: 2 in, 2 out]
      n17 = property on="GUIdevice 11" class="Str"("Val(Sgnl)"=w2) -> ()  [unwired: 2 in, 2 out]
      n18 = property on="GUIdevice 12" class="Str"("Val(Sgnl)"=w1) -> ()  [unwired: 2 in, 2 out]
    }
    frame #1 {
      w35 = path "Z:/data/Thomson/BP_HTT" ("base path")
      w107 = T21 0 items=["Grayscale (U8)", "Grayscale (I16)", "Grayscale (SGL)", "Complex (CSG)", "RGB (U32)", "HSL (U32)", "RGB (U64)", "Grayscale (U16)"] ("Image Type")
      # "NOT FOR YOU MOFO"
      n19 = control-ref of="Position.Axis 111::98"() -> (w44:refnum<vi>)
      n20 = control-ref of="Position.Axis 112::98"() -> (w45:refnum<vi>)
      n21 = control-ref of="Position.Axis 113::98"() -> (w46:refnum<vi>)
      n22 = control-ref of="Position.Axis 121::98"() -> (w47:refnum<vi>)
      n23 = control-ref of="Position.Axis 122::98"() -> (w48:refnum<vi>)
      n24 = control-ref of="Position.Axis 123::98"() -> (w49:refnum<vi>)
      n25 = control-ref of="Position.Axis 131::98"() -> (w50:refnum<vi>)
      n26 = control-ref of="Position.Axis 132::98"() -> (w51:refnum<vi>)
      n27 = control-ref of="Position.Axis 133::98"() -> (w52:refnum<vi>)
      n28 = control-ref of="Position.Axis 141::98"() -> (w53:refnum<vi>)
      n29 = control-ref of="Position.Axis 142::98"() -> (w54:refnum<vi>)
      n30 = control-ref of="Position.Axis 143::98"() -> (w55:refnum<vi>)
      n31 = control-ref of="Position.Axis 211::98"() -> (w56:refnum<vi>)
      n32 = control-ref of="Position.Axis 212::98"() -> (w57:refnum<vi>)
      n33 = control-ref of="Position.Axis 213::98"() -> (w58:refnum<vi>)
      n34 = control-ref of="Position.Axis 221::98"() -> (w59:refnum<vi>)
      n35 = control-ref of="Position.Axis 222::98"() -> (w60:refnum<vi>)
      n36 = control-ref of="Position.Axis 223::98"() -> (w61:refnum<vi>)
      n37 = control-ref of="Position.Axis 231::98"() -> (w62:refnum<vi>)
      n38 = control-ref of="Position.Axis 232::98"() -> (w63:refnum<vi>)
      n39 = control-ref of="Position.Axis 233::98"() -> (w64:refnum<vi>)
      n40 = control-ref of="Position.Axis 241::98"() -> (w65:refnum<vi>)
      n41 = control-ref of="Position.Axis 242::98"() -> (w66:refnum<vi>)
      n42 = control-ref of="Position.Axis 243::98"() -> (w67:refnum<vi>)
      n43 = control-ref of="Position.Axis 311::98"() -> (w68:refnum<vi>)
      n44 = control-ref of="Position.Axis 312::98"() -> (w69:refnum<vi>)
      n45 = control-ref of="Position.Axis 313::98"() -> (w70:refnum<vi>)
      n46 = control-ref of="Position.Axis 321::98"() -> (w71:refnum<vi>)
      n47 = control-ref of="Position.Axis 322::98"() -> (w72:refnum<vi>)
      n48 = control-ref of="Position.Axis 323::98"() -> (w73:refnum<vi>)
      n49 = control-ref of="Position.Axis 331::98"() -> (w74:refnum<vi>)
      n50 = control-ref of="Position.Axis 332::98"() -> (w75:refnum<vi>)
      n51 = control-ref of="Position.Axis 333::98"() -> (w76:refnum<vi>)
      n52 = control-ref of="Position.Axis 341::98"() -> (w77:refnum<vi>)
      n53 = control-ref of="Position.Axis 342::98"() -> (w78:refnum<vi>)
      n54 = control-ref of="Position.Axis 343::98"() -> (w79:refnum<vi>)
      n55 = control-ref of="Position.Axis 411::98"() -> (w80:refnum<vi>)
      n56 = control-ref of="Position.Axis 412::98"() -> (w81:refnum<vi>)
      n57 = control-ref of="Position.Axis 413::98"() -> (w82:refnum<vi>)
      n58 = control-ref of="Position.Axis 421::98"() -> (w83:refnum<vi>)
      n59 = control-ref of="Position.Axis 422::98"() -> (w84:refnum<vi>)
      n60 = control-ref of="Position.Axis 423::98"() -> (w85:refnum<vi>)
      n61 = control-ref of="Position.Axis 431::98"() -> (w86:refnum<vi>)
      n62 = control-ref of="Position.Axis 432::98"() -> (w87:refnum<vi>)
      n63 = control-ref of="Position.Axis 433::98"() -> (w88:refnum<vi>)
      n64 = control-ref of="Position.Axis 441::98"() -> (w89:refnum<vi>)
      n65 = control-ref of="Position.Axis 442::98"() -> (w90:refnum<vi>)
      n66 = control-ref of="Position.Axis 443::98"() -> (w91:refnum<vi>)
      n67 = control-ref of="Position.Axis 511::98"() -> (w92:refnum<vi>)
      n68 = control-ref of="Position.Axis 512::98"() -> (w93:refnum<vi>)
      n69 = control-ref of="Position.Axis 513::98"() -> (w94:refnum<vi>)
      n70 = control-ref of="Position.Axis 521::98"() -> (w95:refnum<vi>)
      n71 = control-ref of="Position.Axis 522::98"() -> (w96:refnum<vi>)
      n72 = control-ref of="Position.Axis 523::98"() -> (w97:refnum<vi>)
      n73 = control-ref of="Position.Axis 531::98"() -> (w98:refnum<vi>)
      n74 = control-ref of="Position.Axis 532::98"() -> (w99:refnum<vi>)
      n75 = control-ref of="Position.Axis 533::98"() -> (w100:refnum<vi>)
      n76 = control-ref of="Position.Axis 541::98"() -> (w101:refnum<vi>)
      n77 = control-ref of="Position.Axis 542::98"() -> (w102:refnum<vi>)
      n78 = control-ref of="Position.Axis 543::98"() -> (w103:refnum<vi>)
      n79 = control-ref of="Position.Axis 111::99"() -> (w235:refnum<vi>)
      n80 = control-ref of="Position.Axis 112::99"() -> (w234:refnum<vi>)
      n81 = control-ref of="Position.Axis 113::99"() -> (w233:refnum<vi>)
      n82 = control-ref of="Position.Axis 121::99"() -> (w232:refnum<vi>)
      n83 = control-ref of="Position.Axis 122::99"() -> (w231:refnum<vi>)
      n84 = control-ref of="Position.Axis 123::99"() -> (w230:refnum<vi>)
      n85 = control-ref of="Position.Axis 131::99"() -> (w229:refnum<vi>)
      n86 = control-ref of="Position.Axis 132::99"() -> (w228:refnum<vi>)
      n87 = control-ref of="Position.Axis 133::99"() -> (w227:refnum<vi>)
      n88 = control-ref of="Position.Axis 141::99"() -> (w226:refnum<vi>)
      n89 = control-ref of="Position.Axis 142::99"() -> (w225:refnum<vi>)
      n90 = control-ref of="Position.Axis 143::99"() -> (w224:refnum<vi>)
      n91 = control-ref of="Position.Axis 211::99"() -> (w223:refnum<vi>)
      n92 = control-ref of="Position.Axis 212::99"() -> (w222:refnum<vi>)
      n93 = control-ref of="Position.Axis 213::99"() -> (w221:refnum<vi>)
      n94 = control-ref of="Position.Axis 221::99"() -> (w220:refnum<vi>)
      n95 = control-ref of="Position.Axis 222::99"() -> (w219:refnum<vi>)
      n96 = control-ref of="Position.Axis 223::99"() -> (w218:refnum<vi>)
      n97 = control-ref of="Position.Axis 231::99"() -> (w217:refnum<vi>)
      n98 = control-ref of="Position.Axis 232::99"() -> (w216:refnum<vi>)
      n99 = control-ref of="Position.Axis 233::99"() -> (w215:refnum<vi>)
      n100 = control-ref of="Position.Axis 241::99"() -> (w214:refnum<vi>)
      n101 = control-ref of="Position.Axis 242::99"() -> (w213:refnum<vi>)
      n102 = control-ref of="Position.Axis 243::99"() -> (w212:refnum<vi>)
      n103 = control-ref of="Position.Axis 311::99"() -> (w211:refnum<vi>)
      n104 = control-ref of="Position.Axis 312::99"() -> (w210:refnum<vi>)
      n105 = control-ref of="Position.Axis 313::99"() -> (w209:refnum<vi>)
      n106 = control-ref of="Position.Axis 321::99"() -> (w208:refnum<vi>)
      n107 = control-ref of="Position.Axis 322::99"() -> (w207:refnum<vi>)
      n108 = control-ref of="Position.Axis 323::99"() -> (w206:refnum<vi>)
      n109 = control-ref of="Position.Axis 331::99"() -> (w205:refnum<vi>)
      n110 = control-ref of="Position.Axis 332::99"() -> (w204:refnum<vi>)
      n111 = control-ref of="Position.Axis 333::99"() -> (w203:refnum<vi>)
      n112 = control-ref of="Position.Axis 341::99"() -> (w202:refnum<vi>)
      n113 = control-ref of="Position.Axis 342::99"() -> (w201:refnum<vi>)
      n114 = control-ref of="Position.Axis 343::99"() -> (w200:refnum<vi>)
      n115 = control-ref of="Position.Axis 411::99"() -> (w199:refnum<vi>)
      n116 = control-ref of="Position.Axis 412::99"() -> (w198:refnum<vi>)
      n117 = control-ref of="Position.Axis 413::99"() -> (w197:refnum<vi>)
      n118 = control-ref of="Position.Axis 421::99"() -> (w196:refnum<vi>)
      n119 = control-ref of="Position.Axis 422::99"() -> (w195:refnum<vi>)
      n120 = control-ref of="Position.Axis 423::99"() -> (w194:refnum<vi>)
      n121 = control-ref of="Position.Axis 431::99"() -> (w193:refnum<vi>)
      n122 = control-ref of="Position.Axis 432::99"() -> (w192:refnum<vi>)
      n123 = control-ref of="Position.Axis 433::99"() -> (w191:refnum<vi>)
      n124 = control-ref of="Position.Axis 441::99"() -> (w190:refnum<vi>)
      n125 = control-ref of="Position.Axis 442::99"() -> (w189:refnum<vi>)
      n126 = control-ref of="Position.Axis 443::99"() -> (w188:refnum<vi>)
      n127 = control-ref of="Position.Axis 511::99"() -> (w187:refnum<vi>)
      n128 = control-ref of="Position.Axis 512::99"() -> (w186:refnum<vi>)
      n129 = control-ref of="Position.Axis 513::99"() -> (w185:refnum<vi>)
      n130 = control-ref of="Position.Axis 521::99"() -> (w184:refnum<vi>)
      n131 = control-ref of="Position.Axis 522::99"() -> (w183:refnum<vi>)
      n132 = control-ref of="Position.Axis 523::99"() -> (w182:refnum<vi>)
      n133 = control-ref of="Position.Axis 531::99"() -> (w181:refnum<vi>)
      n134 = control-ref of="Position.Axis 532::99"() -> (w180:refnum<vi>)
      n135 = control-ref of="Position.Axis 533::99"() -> (w179:refnum<vi>)
      n136 = control-ref of="Position.Axis 541::99"() -> (w178:refnum<vi>)
      n137 = control-ref of="Position.Axis 542::99"() -> (w177:refnum<vi>)
      n138 = control-ref of="Position.Axis 543::99"() -> (w176:refnum<vi>)
      n139 = Build Array(w44, w45, w46, w47, w48, w49, w50, w51, w52, w53, w54, w55, w56, w57, w58, w59, w60, w61, w62, w63, w64, w65, w66, w67, w68, w69, w70, w71, w72, w73, w74, w75, w76, w77, w78, w79, w80, w81, w82, w83, w84, w85, w86, w87, w88, w89, w90, w91, w92, w93, w94, w95, w96, w97, w98, w99, w100, w101, w102, w103) -> (w41:refnum<vi>[])
      n140 = Build Array(w235, w234, w233, w232, w231, w230, w229, w228, w227, w226, w225, w224, w223, w222, w221, w220, w219, w218, w217, w216, w215, w214, w213, w212, w211, w210, w209, w208, w207, w206, w205, w204, w203, w202, w201, w200, w199, w198, w197, w196, w195, w194, w193, w192, w191, w190, w189, w188, w187, w186, w185, w184, w183, w182, w181, w180, w179, w178, w177, w176) -> (w40:refnum<vi>[])
      n141 = Build Array (concatenate)(w40, w41) -> (→"motor refs":refnum<vi>[])
      n142 = call "getMotorNames.vi"("DeviceName"="GUIdevice 99") -> ("elements"=w38:string[])  [unwired: 10 in]
      n143 = call "getMotorNames.vi"("DeviceName"="GUIdevice 98") -> ("elements"=w37:string[])  [unwired: 10 in]
      n144 = Build Array (concatenate)(w38, w37) -> (w42:string[])
      "Names" <- w42
      n145 = property on="Motor CCD 1" class="Ring (strict)"("Strings []"=w42) -> ()  [unwired: 2 in, 2 out]
      n146 = property on="Motor CCD 2" class="Ring (strict)"("Strings []"=w42) -> ()  [unwired: 2 in, 2 out]
      n147 = property on="Motor CCD 3" class="Ring (strict)"("Strings []"=w42) -> ()  [unwired: 2 in, 2 out]
      n148 = property on="Motor CCD 4" class="Ring (strict)"("Strings []"=w42) -> ()  [unwired: 2 in, 2 out]
      n149 = property on="Motor CCD 5" class="Ring (strict)"("Strings []"=w42) -> ()  [unwired: 2 in, 2 out]
      n150 = property on="Motor CCD 6" class="Ring (strict)"("Strings []"=w42) -> ()  [unwired: 2 in, 2 out]
      n151 = property on="Motor CCD 7" class="Ring (strict)"("Strings []"=w42) -> ()  [unwired: 2 in, 2 out]
      n152 = property on="Motor CCD 8" class="Ring (strict)"("Strings []"=w42) -> ()  [unwired: 2 in, 2 out]
      n153 = property on="Motor CCD 9" class="Ring (strict)"("Strings []"=w42) -> ()  [unwired: 2 in, 2 out]
      n154 = property on="Motor CCD 10" class="Ring (strict)"("Strings []"=w42) -> ()  [unwired: 2 in, 2 out]
      n155 = property on="Motor CCD 11" class="Ring (strict)"("Strings []"=w42) -> ()  [unwired: 2 in, 2 out]
      n156 = property on="Motor CCD 12" class="Ring (strict)"("Strings []"=w42) -> ()  [unwired: 2 in, 2 out]
      n157 = property on="ActiveMotor" class="Ring (strict)"("Strings []"=w38) -> ()  [unwired: 2 in, 2 out]
      n158 = control-ref of="Target.X::1"() -> (w162:refnum<vi>)
      n159 = control-ref of="Target.Y::1"() -> (w161:refnum<vi>)
      n160 = control-ref of="Target.X::2"() -> (w160:refnum<vi>)
      n161 = control-ref of="Target.Y::2"() -> (w159:refnum<vi>)
      n162 = control-ref of="Target.X::3"() -> (w158:refnum<vi>)
      n163 = control-ref of="Target.Y::3"() -> (w157:refnum<vi>)
      n164 = control-ref of="Target.X::4"() -> (w156:refnum<vi>)
      n165 = control-ref of="Target.Y::4"() -> (w155:refnum<vi>)
      n166 = control-ref of="Target.X::5"() -> (w154:refnum<vi>)
      n167 = control-ref of="Target.Y::5"() -> (w153:refnum<vi>)
      n168 = control-ref of="Target.X::6"() -> (w152:refnum<vi>)
      n169 = control-ref of="Target.Y::6"() -> (w151:refnum<vi>)
      n170 = control-ref of="Target.X::7"() -> (w150:refnum<vi>)
      n171 = control-ref of="Target.Y::7"() -> (w149:refnum<vi>)
      n172 = control-ref of="Target.X::8"() -> (w148:refnum<vi>)
      n173 = control-ref of="Target.Y::8"() -> (w147:refnum<vi>)
      n174 = control-ref of="Target.X::9"() -> (w124:refnum<vi>)
      n175 = control-ref of="Target.Y::9"() -> (w123:refnum<vi>)
      n176 = control-ref of="Target.X::10"() -> (w122:refnum<vi>)
      n177 = control-ref of="Target.Y::10"() -> (w121:refnum<vi>)
      n178 = control-ref of="Target.X::11"() -> (w120:refnum<vi>)
      n179 = control-ref of="Target.Y::11"() -> (w119:refnum<vi>)
      n180 = control-ref of="Target.X::12"() -> (w118:refnum<vi>)
      n181 = control-ref of="Target.Y::12"() -> (w117:refnum<vi>)
      n182 = call "IMAQ Create"("Image Name"="GUIdevice 8", "Image Type"=w107) -> ("New Image"=→"image::8":T9)  [unwired: 3 in, 1 out]
      n183 = call "IMAQ Create"("Image Name"="GUIdevice 9", "Image Type"=w107) -> ("New Image"=→"image::9":T9)  [unwired: 3 in, 1 out]
      n184 = call "IMAQ Create"("Image Name"="GUIdevice 10", "Image Type"=w107) -> ("New Image"=→"image::10":T9)  [unwired: 3 in, 1 out]
      n185 = call "IMAQ Create"("Image Name"="GUIdevice 6", "Image Type"=w107) -> ("New Image"=→"image::6":T9)  [unwired: 3 in, 1 out]
      n186 = call "IMAQ Create"("Image Name"="GUIdevice 7", "Image Type"=w107) -> ("New Image"=→"image::7":T9)  [unwired: 3 in, 1 out]
      n187 = call "IMAQ Create"("Image Name"="GUIdevice 11", "Image Type"=w107) -> ("New Image"=→"image::11":T9)  [unwired: 3 in, 1 out]
      n188 = call "IMAQ Create"("Image Name"="GUIdevice 12", "Image Type"=w107) -> ("New Image"=→"image::12":T9)  [unwired: 3 in, 1 out]
      n189 = call "IMAQ Create"("Image Name"="GUIdevice 2") -> ("New Image"=→"image::2":T9)  [unwired: 4 in, 1 out]
      n190 = call "IMAQ Create"("Image Name"="GUIdevice 4", "Image Type"=w107) -> ("New Image"=→"image::4":T9)  [unwired: 3 in, 1 out]
      n191 = call "IMAQ Create"("Image Name"="GUIdevice 1", "Image Type"=w107) -> ("New Image"=→"image::1":T9)  [unwired: 3 in, 1 out]
      n192 = call "IMAQ Create"("Image Name"="GUIdevice 3", "Image Type"=w107) -> ("New Image"=→"image::3":T9)  [unwired: 3 in, 1 out]
      n193 = call "IMAQ Create"("Image Name"="GUIdevice 5", "Image Type"=w107) -> ("New Image"=→"image::5":T9)  [unwired: 3 in, 1 out]
      n194 = Build Array("GUIdevice 1", "GUIdevice 2", "GUIdevice 3", "GUIdevice 4", "GUIdevice 5", "GUIdevice 6", "GUIdevice 7", "GUIdevice 8", "GUIdevice 9", "GUIdevice 10", "GUIdevice 11", "GUIdevice 12") -> (w136:string[])
      "CCDs" <- w136
      n195 = property on="image::8" class="ImageControl"("Caption.Text"="GUIdevice 8") -> ()  [unwired: 2 in, 2 out]
      n196 = property on="image::10" class="ImageControl"("Caption.Text"="GUIdevice 10") -> ()  [unwired: 2 in, 2 out]
      n197 = property on="image::9" class="ImageControl"("Caption.Text"="GUIdevice 9") -> ()  [unwired: 2 in, 2 out]
      n198 = property on="image::1" class="ImageControl"("Caption.Text"="GUIdevice 1") -> ()  [unwired: 2 in, 2 out]
      n199 = property on="image::2" class="ImageControl"("Caption.Text"="GUIdevice 2") -> ()  [unwired: 2 in, 2 out]
      n200 = property on="image::3" class="ImageControl"("Caption.Text"="GUIdevice 3") -> ()  [unwired: 2 in, 2 out]
      n201 = property on="image::4" class="ImageControl"("Caption.Text"="GUIdevice 4") -> ()  [unwired: 2 in, 2 out]
      n202 = property on="image::5" class="ImageControl"("Caption.Text"="GUIdevice 5") -> ()  [unwired: 2 in, 2 out]
      n203 = property on="image::6" class="ImageControl"("Caption.Text"="GUIdevice 6") -> ()  [unwired: 2 in, 2 out]
      n204 = property on="image::7" class="ImageControl"("Caption.Text"="GUIdevice 7") -> ()  [unwired: 2 in, 2 out]
      n205 = property on="image::11" class="ImageControl"("Caption.Text"="GUIdevice 11") -> ()  [unwired: 2 in, 2 out]
      n206 = property on="image::12" class="ImageControl"("Caption.Text"="GUIdevice 12") -> ()  [unwired: 2 in, 2 out]
      n207 = Array To Cluster(array=w136) -> (cluster=→"Cameras":T22)
      n208 = Bundle("Target.X::1"=w162, "Target.Y::1"=w161) -> (w146:T23)  [unwired: 1 in]
      n209 = Bundle("Target.X::2"=w160, "Target.Y::2"=w159) -> (w145:T24)  [unwired: 1 in]
      n210 = Bundle("Target.X::3"=w158, "Target.Y::3"=w157) -> (w144:T25)  [unwired: 1 in]
      n211 = Bundle("Target.X::4"=w156, "Target.Y::4"=w155) -> (w137:T26)  [unwired: 1 in]
      n212 = Bundle("Target.X::5"=w154, "Target.Y::5"=w153) -> (w143:T27)  [unwired: 1 in]
      n213 = Bundle("Target.X::6"=w152, "Target.Y::6"=w151) -> (w142:T28)  [unwired: 1 in]
      n214 = Bundle("Target.X::7"=w150, "Target.Y::7"=w149) -> (w141:T29)  [unwired: 1 in]
      n215 = Bundle("Target.X::8"=w148, "Target.Y::8"=w147) -> (w140:T30)  [unwired: 1 in]
      n216 = Bundle("Target.X::12"=w118, "Target.Y::12"=w117) -> (w113:T31)  [unwired: 1 in]
      n217 = Bundle("Target.X::9"=w124, "Target.Y::9"=w123) -> (w116:T32)  [unwired: 1 in]
      n218 = Bundle("Target.X::10"=w122, "Target.Y::10"=w121) -> (w115:T33)  [unwired: 1 in]
      n219 = Bundle("Target.X::11"=w120, "Target.Y::11"=w119) -> (w114:T34)  [unwired: 1 in]
      n220 = property on="CCDs" class="Ring (strict)"("Strings []"=w136) -> ()  [unwired: 2 in, 2 out]
      n221 = Build Array(w146, w145, w144, w137, w143, w142, w141, w140, w116, w115, w114, w113) -> (w139:T35)
      n222 = Tick Count (ms)() -> (millisecond timer value=→"millisecond timer value":u32)
      n223 = property on="Feedback Global" class="Bool (strict)"("Value"=FALSE ("Feedback Global")) -> ()  [unwired: 2 in, 2 out]
      n224 = Get Date/Time In Seconds() -> (seconds since 1Jan1904=w126:timestamp)
      n225 = Format Date/Time String(time format string (%c)="%Y%m%d%H%M", seconds (now)=w126) -> (date/time string=w125:string)  [unwired: 1 in]
      n226 = Concatenate Strings(w125, "Beampointing_Pico.tdms" ("string")) -> (w129:string)
      n227 = String To Path(string=w129) -> (path=w128:path)
      n228 = Build Path(base path=w35, name or relative path=w128) -> (appended path=w131:path)
      n229 = call <vilib>:"Add State(s) to Queue__jki_lib_state_machine.vi"("State(s) in (\"\")"="Macro: Initialize") -> ("States Out"=w237:string)  [unwired: 14 in]
      n230 = call "supergui create stop queue.vi"() -> ("STOP Queue out"=w33:refnum<queue>)  [unwired: 11 in]
      n231 = Create User Event(user event datatype=T15 {"EventEnum"=enum."new data", "Device name"="Device name"} ("New Event")) -> (user event=w245:refnum<user-event>, error out=w247:errorcluster)  [unwired: 1 in]
      "tcp data event" <- w245
      n232 = while "JKI - String-Based Queued State Machine (Basic) v1.0" {
        shift-right: [w271] -> w135
        shift-left: _ -> [w260]
        shift-right: [w274] -> w163
        shift-left: _ -> [w270]
        shift-right: [w273] -> _
        shift-left: w237 -> [w275]
        tunnel: w139 -> [w268]
        tunnel: w136 -> [w266]
        tunnel: [w266] -> w164
        tunnel: w139 -> [w267]
        tunnel: w131 -> [w258]
        tunnel: w35 -> [w257]
        tunnel: T14 {"Draw"=TRUE, "Target"={"x"=25.0, "y"=25.0}, "Size"={"x"=25.0, "y"=25.0}, "Angle"=0.0, "Color"=8322834, "Thickness"=1, "CrosshairLabel"="xhair"} ("Crosshair") -> [w256]
        tunnel: "ActiveMotorName::99" -> [w255]
        stop <- w272 stop-if-true
        n233 = Unbundle By Name(w260) -> ("active cams"=w259:string[])
        n234 = call <vilib>:"Parse State Queue__jki_lib_state_machine.vi"("State Queue"=w275, "Error In (no error)"=w270) -> ("Remaining States"=w277:string, "Current State"=w278:string, "Arguments"=w276:string)  [unwired: 11 in]
        "Current State" <- w278
        n235 = case shown="\"\", \"Idle\"" w278 {
          selector: w278 -> [_ _ w565 _ _ _ _ _ _ _ _ _ _ _ _ _ _ _ _ _ _ _ _ _ _ _ _ _ _ _ _ _ _ _ _ _ _ _ _ _]
          tunnel: w277 -> [w307 w564 w569 w587 w594 w599 w603 w640 w658 w662 w666 w672 w683 w707 w717 w727 w731 w753 w855 w908 w921 w930 w957 w978 w982 w1001 w1140 w1294 w1385 w1451 w1489 w1509 w1524 w1613 w1665 w1675 w1682 w1715 w1741 w1768]
          tunnel: w276 -> [_ _ _ _ _ _ _ _ _ _ _ w667 w678 _ _ _ _ w748 w806 _ w918 _ _ _ _ w1003 _ w1272 w1362 _ _ _ _ _ _ _ w1679 _ _ _]
          tunnel: w260 -> [w305 w561 w567 w577 w591 w597 w600 _ w654 w659 w664 w670 w677 w704 w715 w719 w728 w745 w807 w906 w913 w926 w949 w971 w979 w985 w1134 w1287 w1378 w1448 w1460 w1506 w1521 w1587 w1662 w1672 w1678 w1703 w1738 w1759]
          tunnel: [w304 w562 w571 w585 errorcluster {"status"=FALSE, "code"=0, "source"=""} ("error out") w596 w601 w612 w651 w660 w663 w668 w680 w705 w716 w725 w729 w749 w811 w898 w919 w928 w955 w976 w980 w1005 w1164 w1292 w1383 w1449 w1487 w1507 w1522 w1572 w1663 w1673 w1680 w1685 w1739 w1766] -> w274
          tunnel: w270 -> [w303 w562 w570 w585 w590 w596 w601 w618 w656 w660 w663 w669 w681 w705 w716 w725 w729 w749 w809 w889 w919 w928 w955 w976 w980 w1005 w1164 w1292 w1383 w1449 w1487 w1507 w1522 w1608 w1663 w1673 w1680 w1701 w1739 w1766]
          tunnel: [w306 w563 w568 w586 w593 w598 w602 w639 w657 w661 w665 w671 w682 w706 w708 w726 w730 w739 w854 w907 w920 w929 w956 w977 w981 w1008 w1165 w1293 w1384 w1450 w1488 w1508 w1523 w1575 w1664 w1674 w1681 w1714 w1740 w1767] -> w273
          tunnel: [_ _ _ _ _ TRUE _ _ _ _ _ _ _ _ _ _ _ _ _ _ _ _ _ _ _ _ _ _ _ _ _ _ _ _ _ _ _ _ _ _] -> w272
          tunnel: [w300 w561 w567 w576 w591 w597 w600 w606 w654 w659 w664 w670 w677 w704 w715 w719 w728 w750 w844 w906 w912 w925 w948 w970 w979 w1030 w1133 w1287 w1378 w1447 w1460 w1506 w1521 w1587 w1661 w1672 w1677 w1704 w1738 w1758] -> w271
          tunnel: "update speed [ms]" -> [w302 _ _ _ _ _ _ _ _ _ _ _ _ _ _ _ _ _ _ _ _ _ _ _ _ _ _ _ _ _ _ _ _ _ _ _ _ _ _ _]
          tunnel: w268 -> [w299 _ _ _ _ _ _ _ _ _ _ _ _ _ _ _ _ _ _ _ _ _ _ _ _ w1028 _ _ _ _ _ _ _ _ _ _ _ _ w1722 _]
          tunnel: w266 -> [w301 _ _ _ _ _ _ w611 _ _ _ _ _ _ _ _ _ w752 w808 _ w914 _ _ _ _ w993 w1130 w1291 w1382 _ w1461 _ w1510 w1611 _ _ _ _ _ _]
          tunnel: w258 -> [_ _ _ _ _ _ _ w616 _ _ _ _ _ _ _ _ _ _ _ _ _ _ _ _ _ _ _ _ _ _ _ _ _ _ _ _ _ _ _ _]
          tunnel: w257 -> [_ _ _ _ _ _ _ _ _ _ _ _ _ _ _ _ _ _ _ _ _ _ _ _ _ _ _ _ _ _ _ _ _ _ _ _ _ w1694 _ _]
          frame "", "Idle" {
            # "executes when the state queue is empty"
            n236 = event shown="[0] Timeout" {
              selector: _ -> [_ _ _ _ _ _ _ _ _ _ _ _ _ _ _ _ _ _]
              dyn-events: _ -> [_ _ _ _ _ _ _ _ _ _ _ _ _ _ _ _ _ _]
              timeout: w302 -> [_ _ _ _ _ _ _ _ _ _ _ _ _ _ _ _ _ _]
              tunnel: w307 -> [w310 w437 w452 w471 w476 w481 w486 w492 w499 w504 w515 w520 w529 w534 w540 w546 w554 w560]
              tunnel: [w325 w436 w451 w470 w475 w480 w485 w491 w498 w503 w514 w519 w528 w533 w539 w545 w553 w559] -> w306
              tunnel: w305 -> [w315 w434 w448 w467 w473 w478 w483 w489 w496 w501 w513 w517 w522 w531 w537 w543 w551 w557]
              tunnel: [w319 w435 w450 w469 w474 w479 w484 w490 w497 w502 w505 w518 w527 w532 w538 w544 w552 w558] -> w304
              tunnel: w303 -> [w322 w435 w450 w469 w474 w479 w484 w490 w497 w502 w506 w518 w527 w532 w538 w544 w552 w558]
              tunnel: [w324 w434 w448 w466 w473 w478 w483 w489 w496 w501 w513 w517 w522 w531 w537 w543 w551 w557] -> w300
              tunnel: w301 -> [w342 _ w444 _ _ _ _ _ _ _ _ _ _ _ _ _ _ _]
              tunnel: w299 -> [_ _ w446 _ _ _ _ _ _ _ _ _ _ _ _ _ _ _]
              event Timeout {
                n237 = event-data() -> ()  [unwired: 1 in, 1 out]
                n238 = Unbundle By Name(w315) -> ("Centroid X"=w312:dbl[][], "Centroid Y"=w352:dbl[][], "Size"=w345:dbl[][], "detection para"=w341:T3[], "active cams"=w336:string[], "thresholds"=w333:cluster{"Lower value":sgl, "Upper value":sgl}[])
                n239 = Unbundle By Name(w315) -> ("active ccd"=w314:i32)
                n240 = call <userlib>:"Tick Count (ms)__ogtk.vi"("error in (no error)"=w322) -> ("error out"=w321:errorcluster, "millisecond timer value"=→"millisecond timer 2":u32)  [unwired: 9 in]
                n241 = for {
                  N: 12 ("Numeric 2") -> [_]
                  tunnel: w336 -> [w397] mode=indexing
                  tunnel: [w398] -> w350 mode=indexing
                  tunnel: w342 -> [w421]
                  tunnel: w341 -> [w419]
                  tunnel: [w417] -> w318 mode=indexing
                  tunnel: [w416] -> w316 mode=indexing
                  tunnel: [w414] -> w337 mode=indexing
                  tunnel: "autodetect" -> [w408]
                  tunnel: w321 -> [w422]
                  tunnel: [w423] -> w343
                  shift-right: [w405] -> w313
                  shift-left: w333 -> [w407]
                  shift-right: [w392] -> w351
                  shift-left: w312 -> [w394]
                  shift-right: [w388] -> w353
                  shift-left: w352 -> [w390]
                  shift-right: [w382] -> w344
                  shift-left: w345 -> [w384]
                  w386 = 0 ("index")
                  n242 = call-poly <userlib>:"Filter 1D Array__ogtk.vi"("items to filter"=w397, "array"=w421) -> ("filtered item indices"=w420:i32[])  [unwired: 4 in, 1 out]
                  n243 = Index Array(array=w420) -> (element=w383:i32)  [unwired: 1 in]
                  n244 = Index Array(array=w384, index (row)=w383) -> (element=w412:dbl[])  [unwired: 1 in]
                  n245 = Index Array(array=w390, index (row)=w383) -> (element=w413:dbl[])  [unwired: 1 in]
                  n246 = Index Array(array=w407, index=w383) -> (element=w411:cluster{"Lower value":sgl, "Upper value":sgl})
                  n247 = Index Array(array=w394, index (row)=w383) -> (element=w396:dbl[])  [unwired: 1 in]
                  n248 = Index Array(array=w419, index=w383) -> (element=w415:T3)
                  n249 = call "CENTRIOD DETECTION.vi"("Refnum in"=w397, "auto threshold"=w408, "Threshold Range In"=w411, "beam detection para"=w415, "error in (no error)"=w422) -> ("Bounding Rect"=w414:T36, "Particle Reports (Pixels)"=w416:T1, "Threshold Range Out"=w406:cluster{"Lower value":sgl, "Upper value":sgl}, "Centriod"=w424:cluster{"X":dbl, "Y":dbl}, "error out"=w423:errorcluster)  [unwired: 7 in, 3 out]
                  n250 = Unbundle By Name(w424) -> ("X"=w395:dbl, "Y"=w391:dbl)
                  n251 = Empty Array?(array=w416) -> (empty?=w418:bool)
                  n252 = Not(x=w418) -> (.not. x?=w417:bool)
                  n253 = Replace Array Subset(array=w407, new element=w406, index=w383) -> (w405:cluster{"Lower value":sgl, "Upper value":sgl}[])
                  n254 = Unbundle By Name(w414) -> ("Right"=w404:dbl, "Left"=w403:dbl, "Bottom"=w402:dbl, "Top"=w401:dbl)
                  n255 = Subtract(x=w404, y=w403) -> (x-y=w399:dbl)
                  n256 = Subtract(x=w402, y=w401) -> (x-y=w400:dbl)
                  n257 = Multiply(x=w399, y=w400) -> (x*y=w387:dbl)
                  n258 = Insert Into Array(array=w413, index=w386, new element=w391) -> (w389:dbl[])
                  n259 = Insert Into Array(array=w412, index=w386, new element=w387) -> (w385:dbl[])
                  n260 = Insert Into Array(array=w396, index=w386, new element=w395) -> (w393:dbl[])
                  n261 = for {
                    shift-right: [w425] -> w409
                    shift-left: dbl[] [] ("Array 4") -> [w428]
                    tunnel: w389 -> [w426] mode=indexing
                    n262 = Equal To 0?(x=w426) -> (x = 0?=w427:bool)
                    n263 = case shown="False" w427 {
                      tunnel: w428 -> [w431 w432]
                      tunnel: w426 -> [w430 _]
                      tunnel: [w429 w432] -> w425
                      frame False {
                        n264 = Build Array (concatenate)(w431, w430) -> (w429:dbl[])
                      }
                      frame True {
                      }
                    }
                  }
                  n265 = Replace Array Subset(array=w394, new element=w393, index (row)=w383) -> (w392:dbl[][])  [unwired: 1 in]
                  n266 = Replace Array Subset(array=w390, new element=w389, index (row)=w383) -> (w388:dbl[][])  [unwired: 1 in]
                  n267 = Replace Array Subset(array=w384, new element=w385, index (row)=w383) -> (w382:dbl[][])  [unwired: 1 in]
                  n268 = Array Size(array=w409) -> (size(s)=w398:i32)
                }
                "detected" <- w318
                "Particle Reports (Pixels)" <- w316
                "Box" <- w337
                n269 = Bundle(0, 1, "Centroid X"=w312) -> (→"Status":cluster{i32, i32, "Centroid X":dbl[][]})  [unwired: 1 in]
                n270 = Index Array(array=w316, index (row)=w314) -> (element=→"particles":T1)  [unwired: 1 in]
                n271 = call <vilib>:"Clear Errors.vi"("error in (no error)"=w343) -> ("error out"=w319:errorcluster)  [unwired: 5 in, 1 out]
                n272 = local read "Img to avg"() -> (w327:i32)
                n273 = local read "Numeric"() -> (w330:dbl)
                n274 = Increment(x=w327) -> (x+1=w326:i32)
                n275 = Greater Or Equal?(x=w330, y=w326) -> (x >= y?=w323:bool)
                n276 = Increment(x=w330) -> (x+1=w329:dbl)
                n277 = Select(t=0.0, s=w323, f=w329) -> (s? t:f=w328:dbl)
                n278 = local write "Numeric"(w328) -> ()
                n279 = for {
                  tunnel: w350 -> [w374] mode=indexing
                  tunnel: w336 -> [w381] mode=indexing
                  shift-right: [w376] -> w346
                  shift-left: "" ("GUIdevice 7") -> [w379]
                  tunnel: [w369] -> w348 mode=indexing
                  tunnel: "Detection Rate" -> [w373]
                  tunnel: w328 -> [w371]
                  n280 = local read "Img to avg"() -> (w375:i32)
                  n281 = Greater Or Equal?(x=w374, y=w375) -> (x >= y?=w370:bool)
                  n282 = Multiply(x=w373, y=w371) -> (x*y=w372:dbl)
                  n283 = Greater Or Equal?(x=w374, y=w372) -> (x >= y?=w368:bool)
                  n284 = And(x=w370, y=w368) -> (x .and. y?=w369:bool)
                  n285 = Select(t=w381, s=w369, f="") -> (s? t:f=w377:string)
                  n286 = Concatenate Strings(w379, "\t", w377) -> (w376:string)
                }
                n287 = Bundle By Name(cluster=w315, "thresholds"=w313, "detected"=w318) -> (w334:T37)
                n288 = Bundle By Name(cluster=w334, "Centroid X"=w351, "Centroid Y"=w353, "Size"=w344) -> (w309:T37)
                n289 = Unbundle By Name(w309) -> ("img to avg"=w308:i32)
                n290 = Or Array Elements(Boolean array=w348) -> (logical OR=w347:bool)
                n291 = case shown="True" w323 {
                  tunnel: w309 -> [w354 w361]
                  tunnel: [w354 w360] -> w324
                  tunnel: w308 -> [_ w356]
                  frame False {
                  }
                  frame True {
                    n292 = Decrement(x=w356) -> (x-1=w355:i32)
                    n293 = Initialize Array(0.0 ("element"), 12 ("dimension size"), w355) -> (w357:dbl[][])
                    n294 = Bundle By Name(cluster=w361, "Centroid X"=w357, "Centroid Y"=w357, "Size"=w357) -> (w360:T37)
                  }
                }
                n295 = case shown="True" w347 {
                  tunnel: w346 -> [_ w366]
                  tunnel: w310 -> [w362 w364]
                  tunnel: [w362 w363] -> w325
                  frame False {
                  }
                  frame True {
                    n296 = call <vilib>:"Build State String with Arguments__jki_lib_state_machine.vi"("Arguments (\"\")"=w366, "State"="detected") -> ("State with Arguments"=w365:string)  [unwired: 4 in]
                    n297 = call <vilib>:"Add State(s) to Queue__jki_lib_state_machine.vi"("State(s) in (\"\")"=w364, "State(s) at Back (\"\")"=w365) -> ("States Out"=w363:string)  [unwired: 13 in]
                  }
                }
              }
              event "stop": Value Change {
                # "Exit Button Value Change (pressed) Event\n(this executes Macro: Exit to terminate the VI)"
                n298 = event-data() -> ()  [unwired: 1 in, 6 out]
                n299 = call <vilib>:"Add State(s) to Queue__jki_lib_state_machine.vi"("State(s) in Front (\"\")"="Macro: Exit", "State(s) in (\"\")"=w437) -> ("States Out"=w436:string)  [unwired: 13 in]
              }
              event Value Change {
                n300 = event-data() -> ()  [unwired: 1 in, 6 out]
                n301 = property on="Set Centriod Target" class="Bool (strict)"("Value"=FALSE) -> ()  [unwired: 2 in, 2 out]
                n302 = Unbundle By Name(w448) -> ("active ccd"=w440:i32, "Centroid X"=w439:dbl[][], "Centroid Y"=w438:dbl[][])
                n303 = Index Array(array=w444, index=w440) -> (element=w443:string)
                n304 = Concatenate Strings("Do want to update the target of " ("message"), w443, "?" ("string")) -> (w441:string)
                n305 = Two Button Dialog(message=w441) -> (T button?=w447:bool)  [unwired: 2 in]
                n306 = case shown="True" w447 {
                  tunnel: w446 -> [_ w459]
                  tunnel: w440 -> [_ w458]
                  tunnel: w439 -> [_ w465]
                  tunnel: w438 -> [_ w460]
                  frame False {
                  }
                  frame True {
                    n307 = Index Array(array=w465, index (row)=w458) -> (element=w464:dbl[])  [unwired: 1 in]
                    n308 = Index Array(array=w460, index (row)=w458) -> (element=w461:dbl[])  [unwired: 1 in]
                    n309 = Index Array(array=w459, index=w458) -> (element=w457:T31)
                    n310 = Unbundle By Name(w457) -> ("Target.X::12"=w456:refnum<vi>, "Target.Y::12"=w454:refnum<vi>)
                    n311 = Reverse 1D Array(array=w464) -> (reversed array=w463:dbl[])
                    n312 = Reverse 1D Array(array=w461) -> (reversed array=w462:dbl[])
                    n313 = Index Array(array=w463) -> (element=w455:dbl)  [unwired: 1 in]
                    n314 = Index Array(array=w462) -> (element=w453:dbl)  [unwired: 1 in]
                    n315 = property class="DigNum (strict)"(reference=w456, "Val(Sgnl)"=w455) -> ()  [unwired: 1 in, 2 out]
                    n316 = property class="DigNum (strict)"(reference=w454, "Val(Sgnl)"=w453) -> ()  [unwired: 1 in, 2 out]
                  }
                }
                n317 = call <vilib>:"Add State(s) to Queue__jki_lib_state_machine.vi"("State(s) in (\"\")"=w452) -> ("States Out"=w451:string)  [unwired: 14 in]
              }
              event "Feedback Global": Value Change {
                # "Exit Button Value Change (pressed) Event\n(this executes Macro: Exit to terminate the VI)"
                n318 = event-data() -> ("NewVal"=w468:bool)  [unwired: 1 in, 5 out]
                n319 = call <vilib>:"Add State(s) to Queue__jki_lib_state_machine.vi"("State(s) in (\"\")"=w471) -> ("States Out"=w470:string)  [unwired: 14 in]
                n320 = Bundle By Name(cluster=w467, "Feedback global"=w468) -> (w466:T37)
              }
              event Value Change {
                n321 = event-data() -> ()  [unwired: 1 in, 6 out]
                n322 = call <vilib>:"Add State(s) to Queue__jki_lib_state_machine.vi"("State(s) in Front (\"\")"="Move Config", "State(s) in (\"\")"=w476) -> ("States Out"=w475:string)  [unwired: 13 in]
              }
              event Value Change {
                n323 = event-data() -> ()  [unwired: 1 in, 6 out]
                n324 = call <vilib>:"Add State(s) to Queue__jki_lib_state_machine.vi"("State(s) in Front (\"\")"="Detection Config", "State(s) in (\"\")"=w481) -> ("States Out"=w480:string)  [unwired: 13 in]
              }
              event "associated motors": Value Change {
                n325 = event-data() -> ()  [unwired: 1 in, 6 out]
                n326 = call <vilib>:"Add State(s) to Queue__jki_lib_state_machine.vi"("State(s) in (\"\")"=w486, "State(s) at Back (\"\")"="Motor Config" ("State(s) at Back (\"\")")) -> ("States Out"=w485:string)  [unwired: 13 in]
              }
              event "Reset History": Value Change {
                n327 = event-data() -> ()  [unwired: 1 in, 6 out]
                n328 = call <vilib>:"Add State(s) to Queue__jki_lib_state_machine.vi"("State(s) in (\"\")"=w492, "State(s) at Back (\"\")"="Reset History" ("State(s) at Back (\"\")")) -> ("States Out"=w491:string)  [unwired: 13 in]
                n329 = property on="Reset History" class="Bool (strict)"("Value"=FALSE ("Reset History")) -> ()  [unwired: 2 in, 2 out]
              }
              event "ActiveMotor": Value Change {
                n330 = event-data() -> ("NewVal"=w494:u16)  [unwired: 1 in, 5 out]
                n331 = property on="ActiveMotor" class="Ring (strict)"() -> ("Strings []"=w495:string[])  [unwired: 2 in, 2 out]
                n332 = Index Array(array=w495, index=w494) -> (element=w493:string)
                n333 = property on="ActiveMotorName::99" class="Str"("Val(Sgnl)"=w493) -> ()  [unwired: 2 in, 2 out]
                n334 = call <vilib>:"Add State(s) to Queue__jki_lib_state_machine.vi"("State(s) in (\"\")"=w499) -> ("States Out"=w498:string)  [unwired: 14 in]
              }
              event "Save Config": Value Change {
                n335 = event-data() -> ()  [unwired: 1 in, 6 out]
                n336 = call <vilib>:"Add State(s) to Queue__jki_lib_state_machine.vi"("State(s) in (\"\")"=w504, "State(s) at Back (\"\")"="Save Config" ("State(s) at Back (\"\")")) -> ("States Out"=w503:string)  [unwired: 13 in]
              }
              event "Load Config": Value Change {
                n337 = event-data() -> ()  [unwired: 1 in, 6 out]
                n338 = call "File Dialog2"("error in"=w506, "pattern (all files)"="*.cfg", "pattern label"="config") -> ("selected path"=w510:path, "error out"=w505:errorcluster)  [unwired: 9 in, 2 out]
                n339 = Path To String(path=w510) -> (string=w508:string)
                "config path" <- w508
                n340 = call <vilib>:"Build State String with Arguments__jki_lib_state_machine.vi"("Arguments (\"\")"=w508, "State"="Load Config" ("State(s) at Back (\"\")")) -> ("State with Arguments"=w507:string)  [unwired: 4 in]
                n341 = call <vilib>:"Add State(s) to Queue__jki_lib_state_machine.vi"("State(s) in (\"\")"=w515, "State(s) at Back (\"\")"=w507) -> ("States Out"=w514:string)  [unwired: 13 in]
              }
              event "Save Stats": Value Change {
                n342 = event-data() -> ()  [unwired: 1 in, 6 out]
                n343 = call <vilib>:"Add State(s) to Queue__jki_lib_state_machine.vi"("State(s) in (\"\")"=w520, "State(s) at Back (\"\")"="Save Stats" ("State(s) at Back (\"\")")) -> ("States Out"=w519:string)  [unwired: 13 in]
              }
              event "active CCDs": Value Change {
                n344 = event-data() -> ("NewVal"=w526:i32)  [unwired: 1 in, 5 out]
                n345 = Unbundle By Name(w522) -> ("active cams"=w521:string[])
                n346 = Index Array(array=w521, index=w526) -> (element=w524:string)
                n347 = call <vilib>:"Build State String with Arguments__jki_lib_state_machine.vi"("Arguments (\"\")"=w524, "State"="active" ("State(s) at Back (\"\")")) -> ("State with Arguments"=w523:string)  [unwired: 4 in]
                n348 = call <vilib>:"Add State(s) to Queue__jki_lib_state_machine.vi"("State(s) in (\"\")"=w529, "State(s) at Back (\"\")"=w523) -> ("States Out"=w528:string)  [unwired: 13 in]
              }
              event "Center": Value Change {
                n349 = event-data() -> ()  [unwired: 1 in, 6 out]
                n350 = call <vilib>:"Add State(s) to Queue__jki_lib_state_machine.vi"("State(s) in (\"\")"=w534, "State(s) at Back (\"\")"="Center" ("State(s) at Back (\"\")")) -> ("States Out"=w533:string)  [unwired: 13 in]
              }
              event "new tdms": Value Change {
                n351 = event-data() -> ()  [unwired: 1 in, 6 out]
                n352 = property on="new tdms" class="Bool (strict)"("Value"=FALSE ("new tdms")) -> ()  [unwired: 2 in, 2 out]
                n353 = call <vilib>:"Add State(s) to Queue__jki_lib_state_machine.vi"("State(s) in (\"\")"=w540, "State(s) at Back (\"\")"="newtdms" ("State(s) at Back (\"\")")) -> ("States Out"=w539:string)  [unwired: 13 in]
              }
              event "deivice ini": Value Change {
                n354 = event-data() -> ()  [unwired: 1 in, 6 out]
                n355 = property on="deivice ini" class="Bool (strict)"("Value"=FALSE ("new tdms")) -> ()  [unwired: 2 in, 2 out]
                n356 = call <vilib>:"Add State(s) to Queue__jki_lib_state_machine.vi"("State(s) in (\"\")"=w546, "State(s) at Back (\"\")"="Device Ini" ("State(s) at Back (\"\")")) -> ("States Out"=w545:string)  [unwired: 13 in]
              }
              event "Img to avg": Value Change {
                n357 = event-data() -> ()  [unwired: 1 in, 6 out]
                n358 = property on="Img to avg" class="DigNum (strict)"() -> ("Value"=w549:i32)  [unwired: 2 in, 2 out]
                n359 = Number To Decimal String(number=w549) -> (decimal integer string=w548:string)  [unwired: 1 in]
                n360 = call <vilib>:"Build State String with Arguments__jki_lib_state_machine.vi"("Arguments (\"\")"=w548, "State"="ImgToAvg" ("State(s) at Back (\"\")")) -> ("State with Arguments"=w547:string)  [unwired: 4 in]
                n361 = call <vilib>:"Add State(s) to Queue__jki_lib_state_machine.vi"("State(s) in (\"\")"=w554, "State(s) at Back (\"\")"=w547) -> ("States Out"=w553:string)  [unwired: 13 in]
              }
              event Panel Close? {
                # "Discard the event because we'll close the front panel ourselves in Macro: Exit"
                # "Close Panel button (pressed) Event\n(this executes Macro: Exit to terminate the VI)"
                n362 = event-data() -> ()  [unwired: 1 in, 1 out]
                n363 = call <vilib>:"Add State(s) to Queue__jki_lib_state_machine.vi"("State(s) in Front (\"\")"="Macro: Exit", "State(s) in (\"\")"=w560) -> ("States Out"=w559:string)  [unwired: 13 in]
                n364 = event-data("Discard?"=TRUE) -> ()  [unwired: 1 in, 1 out]
              }
            }
          }
          frame "---------- Core ----------" {
            # "Do not put any code in this frame.\n(it is a separator no-op)"
            n365 = call <vilib>:"Add State(s) to Queue__jki_lib_state_machine.vi"("State(s) in (\"\")"=w564) -> ("States Out"=w563:string)  [unwired: 14 in]
          }
          frame Default {
            w574 = 42 items=["No error", "Argument error", "Memory is full", "Out of zone", "End of file", "File already open", "Generic file I/O error", "File not found", "File permission error", "Disk is full", "Duplicate path", "Too many files open", "System feature not enabled", "Resource file not found", "Cannot add resource", "Resource not found", "Image not found", "Image memory error", "Pen does not exist", "Config type invalid", "Config token not found", "Config parse error", "Config memory error", "Bad external code format", "Bad external code offset", "External code not present", "Null window", "Destroy window error", "Null menu", "Print aborted", "Bad print record", "Print driver error", "Windows error during printing", "Memory error during printing", "Print dialog error", "Generic print error", "Invalid device refnum", "Device not found", "Device parameter error", "Device unit error", "Cannot open device", "Device call aborted", "Generic error", "Cancelled by user", "Object ID too low", "Object ID too high", "Object not in heap", "Unknown heap", "Unknown object (invalid DefProc)", "Unknown object (DefProc not in table)", "Message out of range", "Invalid (null) method", "Unknown message", "Manager call not supported", "Bad address", "Network operation in progress", "Network operation timed out", "Connection is busy", "Network attribute not supported", "Network error", "Address in use", "System out of memory", "Connection aborted", "Connection refused", "Not connected", "Already connected", "Connection closed", "Initialization error (interapplication manager)", "Bad occurrence", "Wait on unbound occurrence handler", "Occurrence queue overflow", "Datalog type conflict", "Unused", "Unrecognized type (interapplication manager)", "Memory corrupt", "Failed to make temporary DLL", "Old CIN version", "Drag socket not found", "Failed to load drop-object", "Failed to register OLE object", "Failed to release OLE object", "Format specifier type mismatch", "Unknown format specifier", "Too few format specifiers", "Too many format specifiers", "Scan failed", "Newer CIN version", "Error converting to variant", "Runtime menu error", "Password tampered", "Variant attribute not found", "Incompatible variant data type", "Event data is not available", "Event Store is not present", "Occurrence is not found", "Event Queue is not created", "Event info is not available", "Refnum passed is NULL", "Error retrieving Class GUID", "Error retrieving CoClass GUID", "Error retrieving TypeLib GUID.", "Bad built application magic bytes.", "Specific driver is different from the specific driver associated with the Logical Name.", "There is no session opened to the class driver.", "Max Error", "MAX - Error with config objects", "MAX - Error loading configuration", "MAX - Group not supported"]
            # "Current State"
            # "Do not delete, rename, or modify this frame.\n(this is used to capture unhandled states and typos)"
            # "Handle mistyped state name (developer tool)"
            n366 = Format Into String(format string="Software Exception: Unhandled State \"%s\"." ("message"), error in=w570, w565) -> (resulting string=w573:string, error out=w572:errorcluster)  [unwired: 1 in]
            n367 = call <vilib>:"Error Cluster From Error Code.vi"("show call chain? (False)"=TRUE, "error in (no error)"=w572, "error message (\"\")"=w573, "error code (0)"=w574) -> ("error out"=w571:errorcluster)  [unwired: 5 in]
            n368 = call <vilib>:"Add State(s) to Queue__jki_lib_state_machine.vi"("State(s) in (\"\")"=w569) -> ("States Out"=w568:string)  [unwired: 14 in]
          }
          frame "Initialize Core Data" {
            # "Do not delete, rename, or modify this frame.\n(this is used to determine panel behavior on exit)"
            # "originally closed?"
            # "exe?"
            # "If panel starts closed or is an EXE, then close it when we exit"
            n369 = property class="VI"() -> ("Front Panel.Open"=w584:bool)  [unwired: 2 in, 2 out]
            n370 = property class="App"() -> ("App.Kind"=w583:T17)  [unwired: 2 in, 2 out]
            n371 = control-ref of="Current VI Reference"() -> (w578:refnum<vi>)
            n372 = Not(x=w584) -> (.not. x?=w581:bool)
            n373 = Equal?(x=w583, y=T17."Run Time System" ("Application:Kind")) -> (x = y?=w580:bool)
            n374 = Or(x=w581, y=w580) -> (x .or. y?=w579:bool)
            n375 = Bundle By Name(cluster=w577, "Core.Current VI Reference"=w578, "Core.Close Panel on Exit?"=w579) -> (w576:T37)
            n376 = call <vilib>:"Add State(s) to Queue__jki_lib_state_machine.vi"("State(s) in (\"\")"=w587) -> ("States Out"=w586:string)  [unwired: 14 in]
          }
          frame "Error Handler" {
            w588 = T38 0 items=["no dialog", "OK message", "continue or stop message", "OK message + warnings", "continue/stop + warnings"] ("type of dialog (OK msg:1)")
            # "Unhandled Error -- Display it"
            # "Handle any errors here.\nYou can also output any states to clean-up after errors occur"
            # "Clear error"
            n377 = call <vilib>:"General Error Handler.vi"("type of dialog (OK msg:1)"=w588, "error in (no error)"=w590) -> ()  [unwired: 9 in, 5 out]
            n378 = call <vilib>:"Add State(s) to Queue__jki_lib_state_machine.vi"("State(s) in Front (\"\")"="/* Post Error States", "State(s) in (\"\")"=w594) -> ("States Out"=w593:string)  [unwired: 13 in]
          }
          frame "Exit" {
            # "Do not put any code in this frame.\n(No errors that occur here will be handled.)"
            n379 = call <vilib>:"Add State(s) to Queue__jki_lib_state_machine.vi"("State(s) in (\"\")"=w599) -> ("States Out"=w598:string)  [unwired: 14 in]
          }
          frame "---------- Data ----------" {
            # "Do not put any code in this frame.\n(It is a separator no-op. You can make a copy of this frame to create a new Data frame)"
            n380 = call <vilib>:"Add State(s) to Queue__jki_lib_state_machine.vi"("State(s) in (\"\")"=w603) -> ("States Out"=w602:string)  [unwired: 14 in]
          }
          frame "Data: Initialize" {
            w613 = bool[] [FALSE, FALSE, FALSE, FALSE, FALSE, FALSE, FALSE, FALSE, FALSE, FALSE, FALSE, TRUE]  # speedmode Y
            w614 = bool[] [FALSE, FALSE, FALSE, FALSE, FALSE, FALSE, FALSE, FALSE, FALSE, FALSE, FALSE, TRUE]  # speedmode X
            w615 = bool[] [FALSE, FALSE, FALSE, FALSE, TRUE, TRUE, TRUE, FALSE, FALSE, FALSE, FALSE, FALSE]  # detected
            w617 = cluster{"Lower value":sgl, "Upper value":sgl}[] [{"Lower value"=93.0, "Upper value"=255.0}, {"Lower value"=105.0, "Upper value"=255.0}, {"Lower value"=0.0, "Upper value"=255.0}, {"Lower value"=127.0, "Upper value"=255.0}, {"Lower value"=0.0, "Upper value"=255.0}, {"Lower value"=0.0, "Upper value"=255.0}, {"Lower value"=0.0, "Upper value"=255.0}, {"Lower value"=0.0, "Upper value"=255.0}, {"Lower value"=0.0, "Upper value"=255.0}, {"Lower value"=0.0, "Upper value"=255.0}, {"Lower value"=0.0, "Upper value"=255.0}, {"Lower value"=0.0, "Upper value"=255.0}]  # thresholds
            w625 = FALSE  # Feedback global
            w627 = 0  # active ccd
            w605 = 2  # img to avg
            w638 = T39 {"Current VI Reference"=refnum, "Close Panel on Exit?"=FALSE}  # Core
            # "Initialize the shift-register data, here.\n(data names are defined by what you wire into the bundle function)"
            n381 = disable-structure shown="Disabled" {
              disable-tunnel: w618 -> [w646 w650]
              disable-tunnel: w616 -> [w645 _]
              disable-tunnel: [w643 w650] -> w612
              disable-tunnel: w611 -> [w641 _]
              frame Disabled {
                n382 = TDMS Open(6:FALSE ("disable buffering (T)"), 7:enum16{"1.0", "2.0"}."2.0" ("file format version (2.0)"), 8:w646, 10:T18."create or replace" ("operation"), 11:w645) -> (0:w644:errorcluster, 3:w642:refnum<k34>)  [unwired: 2 in]
                n383 = call "TDMSbuffersize.vi"("error in (no error)"=w644, "group names"=w641, "Data Value Reference in"=w642) -> ("error out"=w643:errorcluster)  [unwired: 7 in, 1 out]
              }
              frame Enabled {
              }
            }
            n384 = call <vilib>:"Add State(s) to Queue__jki_lib_state_machine.vi"("State(s) in (\"\")"=w640) -> ("States Out"=w639:string)  [unwired: 14 in]
            n385 = Bundle("Core"=w638, "detection para"="detection para", "thresholds"=w617, "Centroid X"="Centroid X", "Centroid Y"="Centroid Y", "img to avg"=w605, "Mean Centroid X"="Mean Centroid X", "Mean Centroid Y"="Mean Centroid Y", "Offset X"="Offset X", "Offset Y"="Offset Y", "Offset X stats"="Offset X stats", "Offset Y stats"="Offset Y stats", "Size"="Size", "Mean Size"="Mean Size", "Time"="Time", "move properties"="move properties", "active axis refs 2"="active axis refs 2", "active ccd"=w627, "Feedback global"=w625, "Motor X"="Motor X", "Motor Y"="Motor Y", "active cams"="active cams", "Data Value Reference out"=refnum<k34> refnum, "detected"=w615, "speedmode X"=w614, "speedmode Y"=w613) -> (w607:T37)  [unwired: 1 in]
            n386 = Initialize Array(0.0 ("element"), 12 ("dimension size"), w605) -> (w608:dbl[][])
            n387 = Bundle By Name(cluster=w607, "Centroid X"=w608, "Centroid Y"=w608, "Size"=w608) -> (w606:T37)
          }
          frame "Data: Cleanup" {
            # "Cleanup any data and references, here.\n(this is called automatically, by the Macro: Exit)"
            n388 = Unbundle By Name(w654) -> ("Core.Current VI Reference"=w655:refnum<vi>)
            n389 = Close Reference(reference=w655, error in (no error)=w656) -> (error out=w652:errorcluster)
            n390 = Unbundle By Name(w654) -> ("Data Value Reference out"=w653:refnum<k34>)
            n391 = TDMS Close(8:w652, 11:w653) -> (0:w651:errorcluster)  [unwired: 1 out]
            n392 = call <vilib>:"Add State(s) to Queue__jki_lib_state_machine.vi"("State(s) in (\"\")"=w658) -> ("States Out"=w657:string)  [unwired: 14 in]
          }
          frame "---------- UI ----------" {
            # "Do not put any code in this frame.\n(It is a separator no-op. You can make a copy of this frame to create a new UI frame)"
            n393 = call <vilib>:"Add State(s) to Queue__jki_lib_state_machine.vi"("State(s) in (\"\")"=w662) -> ("States Out"=w661:string)  [unwired: 14 in]
          }
          frame "UI: Initialize" {
            # "Initialize the User Interface, here.\n(this is called automatically, by the Macro: Init)"
            n394 = call <vilib>:"Add State(s) to Queue__jki_lib_state_machine.vi"("State(s) in (\"\")"=w666) -> ("States Out"=w665:string)  [unwired: 14 in]
          }
          frame "UI: Cursor Set" {
            # "Argument"
            # "Set and Unset Cursor Busy.\n(Usage: \"UI: Cursor Set >> Busy|Idle\")"
            n395 = case shown="\"Idle\", Default" w667 {
              tunnel: w669 -> [w674 w676]
              tunnel: [w673 w675] -> w668
              frame "Idle", Default {
                n396 = call <vilib>:"Unset Busy.vi"("error in (no error)"=w674) -> ("error out"=w673:errorcluster)  [unwired: 10 in]
              }
              frame "Busy" {
                n397 = call <vilib>:"Set Busy.vi"("error in (no error)"=w676) -> ("error out"=w675:errorcluster)  [unwired: 9 in, 1 out]
              }
            }
            n398 = call <vilib>:"Add State(s) to Queue__jki_lib_state_machine.vi"("State(s) in (\"\")"=w672) -> ("States Out"=w671:string)  [unwired: 14 in]
          }
          frame "UI: Front Panel State" {
            # "Argument"
            # "Set Front Panel Open or Closed\n(Usage: \"UI: Front Panel State >> Open|Close\")"
            n399 = Unbundle By Name(w677) -> ("Core.Current VI Reference"=w679:refnum<vi>)
            n400 = case shown="\"Open\", Default" w678 {
              tunnel: w681 -> [w687 w698]
              tunnel: [w688 w699] -> w680
              tunnel: w679 -> [_ _]
              frame "Open", Default {
                n401 = property class="VI"(error in=w687) -> (reference out=w685:refnum<vi>, error out=w686:errorcluster, "Front Panel.Open"=w684:bool)  [unwired: 1 in]
                n402 = case shown="False" w684 {
                  tunnel: [w691 w694] -> w688
                  tunnel: w686 -> [w690 w694]
                  tunnel: w685 -> [w689 _]
                  frame False {
                    n403 = invoke class="VI" method="FP.Open"(reference=w689, error in=w690, "Activate"=TRUE, "State"=T19."Standard") -> (error out=w691:errorcluster)  [unwired: 1 in, 4 out]
                  }
                  frame True {
                  }
                }
              }
              frame "Close" {
                n404 = property class="VI"(error in=w698) -> (reference out=w696:refnum<vi>, error out=w697:errorcluster, "Front Panel.Open"=w695:bool)  [unwired: 1 in]
                n405 = case shown="True" w695 {
                  tunnel: [w700 w703] -> w699
                  tunnel: w697 -> [w700 w702]
                  tunnel: w696 -> [_ w701]
                  frame False {
                  }
                  frame True {
                    n406 = invoke class="VI" method="FP.Close"(reference=w701, error in=w702) -> (error out=w703:errorcluster)  [unwired: 1 in, 2 out]
                  }
                }
              }
            }
            n407 = call <vilib>:"Add State(s) to Queue__jki_lib_state_machine.vi"("State(s) in (\"\")"=w683) -> ("States Out"=w682:string)  [unwired: 14 in]
          }
          frame "---------- Macro ----------" {
            # "Do not put any code in this frame.\n(It is a separator no-op. You can make a copy of this frame to create a new Macro frame)"
            n408 = call <vilib>:"Add State(s) to Queue__jki_lib_state_machine.vi"("State(s) in (\"\")"=w707) -> ("States Out"=w706:string)  [unwired: 14 in]
          }
          frame "Macro: Initialize" {
            w714 = "Data: Initialize\nInitialize Core Data\nUI: Initialize\nUI: Front Panel State >> Open\nDevice Ini >> 3000\nnewtdms"  # Data: Initialize Initialize Core Data UI: Initialize UI: Front Panel State >> Open Device Ini >> 3000 newtdms
            # "Initialization Macro\n(This is called once, when the VI starts)"
            n409 = property on="Img to avg" class="DigNum (strict)"() -> ("Value"=w712:i32)  [unwired: 2 in, 2 out]
            n410 = call <vilib>:"Add State(s) to Queue__jki_lib_state_machine.vi"("State(s) in Front (\"\")"=w714, "State(s) in (\"\")"=w717) -> ("States Out"=w709:string)  [unwired: 13 in]
            n411 = Number To Decimal String(number=w712) -> (decimal integer string=w711:string)  [unwired: 1 in]
            n412 = call <vilib>:"Build State String with Arguments__jki_lib_state_machine.vi"("Arguments (\"\")"=w711, "State"="ImgToAvg") -> ("State with Arguments"=w710:string)  [unwired: 4 in]
            n413 = call <vilib>:"Add State(s) to Queue__jki_lib_state_machine.vi"("State(s) in (\"\")"=w709, "State(s) at Back (\"\")"=w710) -> ("States Out"=w708:string)  [unwired: 13 in]
          }
          frame "Macro: Exit" {
            # "Exit Macro\n(This is called once, when the VI exits)"
            n414 = Unbundle By Name(w719) -> ("Core.Close Panel on Exit?"=w718:bool)
            n415 = Select(t="UI: Front Panel State >> Close", s=w718, f="") -> (s? t:f=w722:string)
            n416 = call <vilib>:"Add State(s) to Queue__jki_lib_state_machine.vi"("State(s) in (\"\")"=w722, "State(s) at Back (\"\")"="Data: Cleanup\nExit") -> ("States Out"=w720:string)  [unwired: 13 in]
            n417 = call <vilib>:"Add State(s) to Queue__jki_lib_state_machine.vi"("State(s) in Front (\"\")"=w720, "State(s) in (\"\")"=w727) -> ("States Out"=w726:string)  [unwired: 13 in]
          }
          frame "---------- Ini and Configure ----------" {
            # "Template Separator\n(You can make a copy of, or modify, this frame)"
            n418 = call <vilib>:"Add State(s) to Queue__jki_lib_state_machine.vi"("State(s) in (\"\")"=w731) -> ("States Out"=w730:string)  [unwired: 14 in]
          }
          frame "Device Ini" {
            # "Your code here.\n(You can make a copy of, or modify, this frame)"
            n419 = Empty String/Path?(string/path=w748) -> (empty?=w746:bool)
            n420 = case shown="False" w746 {
              tunnel: w748 -> [w785 _]
              tunnel: [w784 0] -> w747
              frame False {
                n421 = Decimal String To Number(string=w785) -> (number=w784:i32)  [unwired: 2 in, 1 out]
              }
              frame True {
              }
            }
            n422 = flat-sequence {
              tunnel: w752 -> [w788]
              tunnel: [w788] -> w751
              tunnel: w747 -> [w787]
              tunnel: w751 -> [w791]
              tunnel: [w789] -> w737
              frame #0 {
                n423 = Wait (ms)(milliseconds to wait=w787) -> ()  [unwired: 1 out]
              }
              frame #1 {
                n424 = for {
                  tunnel: w791 -> [w793] mode=indexing
                  shift-right: [w794] -> w789
                  shift-left: string[] [] -> [w795]
                  n425 = Empty String/Path?(string/path=w793) -> (empty?=w792:bool)
                  n426 = case shown="False" w792 {
                    tunnel: w795 -> [w798 w804]
                    tunnel: [w797 w804] -> w794
                    tunnel: w793 -> [w796 _]
                    frame False {
                      n427 = call "send command.vi"("Device Name"=w796) -> ("status"=w799:bool)  [unwired: 4 in]
                      n428 = case shown="True" w799 {
                        tunnel: w798 -> [w800 w803]
                        tunnel: [w800 w802] -> w797
                        tunnel: w796 -> [_ w801]
                        frame False {
                        }
                        frame True {
                          n429 = Build Array (concatenate)(w803, w801) -> (w802:string[])
                        }
                      }
                    }
                    frame True {
                    }
                  }
                }
              }
            }
            n430 = Unbundle By Name(w745) -> ("active cams"=w738:string[])
            n431 = call <vilib>:"Add State(s) to Queue__jki_lib_state_machine.vi"("State(s) in (\"\")"=w753) -> ("States Out"=w740:string)  [unwired: 14 in]
            n432 = Empty Array?(array=w738) -> (empty?=w742:bool)
            n433 = Equal?(x=w738, y=w737) -> (x = y?=w743:bool[])
            n434 = Not(x=w742) -> (.not. x?=w741:bool)
            n435 = Build Array (concatenate)(w743, w741) -> (w744:bool[])
            n436 = Array Size(array=w737) -> (size(s)=w735:i32)
            n437 = Array Size(array=w738) -> (size(s)=w736:i32)
            n438 = Equal?(x=w736, y=w735) -> (x = y?=w734:bool)
            n439 = And Array Elements(Boolean array=w744) -> (logical AND=w733:bool)
            n440 = And(x=w734, y=w733) -> (x .and. y?=w732:bool)
            n441 = case shown="False" w732 {
              tunnel: [w770 w783] -> w750
              tunnel: w745 -> [w755 w783]
              tunnel: w737 -> [w756 _]
              tunnel: w740 -> [w765 w782]
              tunnel: [w763 w782] -> w739
              frame False {
                n442 = Bundle By Name(cluster=w755, "active cams"=w756) -> (w771:T37)
                n443 = property on="active CCDs" class="LstBox (strict)"("Item Names"=w756) -> ()  [unwired: 2 in, 2 out]
                n444 = Array Size(array=w756) -> (size(s)=w774:i32)
                n445 = for {
                  N: 1 -> [_]
                  shift-right: [w776] -> w769
                  shift-left: timestamp[][] [] ("Time") -> [w778]
                  n446 = for {
                    N: 12 -> [_]
                    tunnel: w778 -> [w781] mode=indexing
                    tunnel: [w779] -> w776 mode=indexing
                    n447 = Get Date/Time In Seconds() -> (seconds since 1Jan1904=w780:timestamp)
                    n448 = Build Array (concatenate)(w781, w780) -> (w779:timestamp[])
                  }
                }
                n449 = Unbundle By Name(w755) -> ("img to avg"=w754:i32)
                n450 = Initialize Array(0.0 ("element"), w774, 0 ("dimension size")) -> (w772:dbl[][])
                n451 = Initialize Array(0.0 ("element"), 12 ("dimension size"), w754) -> (w757:dbl[][])
                n452 = Bundle By Name(cluster=w771, "Offset X stats"=w772, "Offset Y stats"=w772, "Centroid X"=w757, "Centroid Y"=w757, "Mean Centroid X"=w772, "Mean Centroid Y"=w772, "Offset X"=w772, "Offset Y"=w772, "Size"=w757, "Mean Size"=w772, "Motor X"=w772, "Motor Y"=w772) -> (w770:T37)
                n453 = property on="Time" class="Arr (strict)"("Value"=w769) -> ()  [unwired: 2 in, 2 out]
                n454 = property on="config path" class="Str"() -> ("Value"=w762:string)  [unwired: 2 in, 2 out]
                n455 = call <vilib>:"Add State(s) to Queue__jki_lib_state_machine.vi"("State(s) in Front (\"\")"="newtdms\nMove Config\nDetection Config\nactive\nCenter" ("State(s) in Front (\"\")"), "State(s) in (\"\")"=w765) -> ("States Out"=w764:string)  [unwired: 13 in]
                n456 = call <vilib>:"Build State String with Arguments__jki_lib_state_machine.vi"("Arguments (\"\")"=w762, "State"="Load Config" ("State(s) in Front (\"\")")) -> ("State with Arguments"=w760:string)  [unwired: 4 in]
                n457 = call <vilib>:"Add State(s) to Queue__jki_lib_state_machine.vi"("State(s) in Front (\"\")"=w760, "State(s) in (\"\")"=w764) -> ("States Out"=w763:string)  [unwired: 13 in]
                "name array" <- w756
              }
              frame True {
              }
            }
          }
          frame "Load Config" {
            # "Your code here.\n(You can make a copy of, or modify, this frame)"
            n458 = Unbundle By Name(w807) -> ("detection para"=w850:T3[], "move properties"=w847:T2[], "thresholds"=w842:cluster{"Lower value":sgl, "Upper value":sgl}[])
            n459 = Empty String/Path?(string/path=w806) -> (empty?=w805:bool)
            n460 = property on="Load Config" class="Bool (strict)"("Value"=FALSE ("Load Config")) -> ()  [unwired: 2 in, 2 out]
            n461 = case shown="False" w805 {
              tunnel: [w861 T5 {"CCDs"=[], "move properties"=[], "detection para"=[], "thresholds"=[], "Value"={"Motor CCD 1"=0, "Motor CCD 2"=0, "Motor CCD 3"=0, "Motor CCD 4"=0, "Motor CCD 5"=0, "Motor CCD 6"=0, "Motor CCD 7"=0, "Motor CCD 8"=0, "Motor CCD 9"=0, "Motor CCD 10"=0, "Motor CCD 11"=0, "Motor CCD 12"=0}} ("output cluster 2")] -> w852
              tunnel: [w859 w868] -> w812
              tunnel: w806 -> [w858 _]
              tunnel: w809 -> [w856 w868]
              tunnel: w807 -> [_ _]
              frame False {
                n462 = String To Path(string=w858) -> (path=w857:path)
                n463 = Open/Create/Replace File(file path (use dialog)=w857, error in=w856, operation (0:open)=T20."open or create") -> (refnum out=w863:refnum<file>, error out=w864:errorcluster)  [unwired: 3 in, 1 out]
                n464 = Read from Binary File(5:"output cluster 2", 8:w864, 11:w863) -> (0:w865:errorcluster, 2:w861:T5, 3:w866:refnum<file>)  [unwired: 3 in, 1 out]
                n465 = Close File(refnum=w866, error in=w865) -> (error out=w859:errorcluster)  [unwired: 1 out]
              }
              frame True {
              }
            }
            n466 = Unbundle By Name(w852) -> ("Value"=w839:T7, "CCDs"=w851:string[], "detection para"=w849:T3[], "move properties"=w848:T2[], "thresholds"=w843:cluster{"Lower value":sgl, "Upper value":sgl}[])
            n467 = Cluster To Array(cluster=w839) -> (array=w840:u16[])
            n468 = call <vilib>:"Add State(s) to Queue__jki_lib_state_machine.vi"("State(s) in (\"\")"=w855, "State(s) at Back (\"\")"="Motor Config" ("State(s) at Back (\"\")")) -> ("States Out"=w854:string)  [unwired: 13 in]
            n469 = for {
              tunnel: w851 -> [w884]
              tunnel: w849 -> [w886]
              tunnel: w848 -> [w885]
              shift-right: [w878] -> w846
              shift-left: w850 -> [w883]
              shift-right: [w876] -> w845
              shift-left: w847 -> [w882]
              tunnel: w808 -> [w881] mode=indexing
              tunnel: w843 -> [w877]
              shift-right: [w873] -> w841
              shift-left: w842 -> [w875]
              tunnel: w840 -> [w872]
              tunnel: [w869] -> w838 mode=indexing
              i -> [w870]
              n470 = call-poly <userlib>:"Filter 1D Array__ogtk.vi"("items to filter"=w881, "array"=w884) -> ("filtered item indices"=w887:i32[])  [unwired: 4 in, 1 out]
              n471 = Index Array(array=w887) -> (element=w871:i32)  [unwired: 1 in]
              n472 = Index Array(array=w872, index=w871) -> (element=w869:u16)
              n473 = Index Array(array=w886, index=w871) -> (element=w880:T3)
              n474 = Index Array(array=w885, index=w871) -> (element=w879:T2)
              n475 = Index Array(array=w877, index=w871) -> (element=w874:cluster{"Lower value":sgl, "Upper value":sgl})
              n476 = Replace Array Subset(array=w883, new element=w880, index=w870) -> (w878:T3[])
              n477 = Replace Array Subset(array=w882, new element=w879, index=w870) -> (w876:T2[])
              n478 = Replace Array Subset(array=w875, new element=w874, index=w870) -> (w873:cluster{"Lower value":sgl, "Upper value":sgl}[])
            }
            n479 = Index Array(array=w838, index #1=0 ("index (row)"), index #2=1 ("index (row)"), index #3=2 ("index (row)"), index #4=3 ("index (row)"), index #5=4 ("index (row)"), index #6=5 ("index (row)"), index #7=6 ("index (row)"), index #8=7 ("index (row)"), index #9=8 ("index (row)"), index #10=9 ("index (row)"), index #11=10 ("index (row)"), index #12=11 ("index (row)")) -> (element #1=w825:u16, element #2=w824:u16, element #3=w823:u16, element #4=w822:u16, element #5=w821:u16, element #6=w820:u16, element #7=w819:u16, element #8=w818:u16, element #9=w817:u16, element #10=w816:u16, element #11=w815:u16, element #12=w814:u16)
            n480 = Bundle By Name(cluster=w839, "Motor CCD 1"=w825, "Motor CCD 2"=w824, "Motor CCD 3"=w823, "Motor CCD 4"=w822, "Motor CCD 5"=w821, "Motor CCD 6"=w820, "Motor CCD 7"=w819, "Motor CCD 8"=w818, "Motor CCD 9"=w817, "Motor CCD 10"=w816, "Motor CCD 11"=w815, "Motor CCD 12"=w814) -> (w813:T7)
            n481 = Bundle By Name(cluster=w807, "detection para"=w846, "move properties"=w845, "thresholds"=w841) -> (w844:T37)
            n482 = property on="associated motors" class="Clust (strict)"(error in=w812, "Val(Sgnl)"=w813) -> (error out=w811:errorcluster)  [unwired: 1 in, 1 out]
          }
          frame "Save Config" {
            # "Your code here.\n(You can make a copy of, or modify, this frame)"
            n483 = Unbundle By Name(w906) -> ("move properties"=w893:T2[], "detection para"=w901:T3[], "thresholds"=w890:cluster{"Lower value":sgl, "Upper value":sgl}[])
            n484 = property on="associated motors" class="Clust (strict)"() -> ("Value"=w900:T7)  [unwired: 2 in, 2 out]
            n485 = property on="Save Config" class="Bool (strict)"("Value"=FALSE ("Save Config")) -> ()  [unwired: 2 in, 2 out]
            n486 = local read "CCDs"() -> (w891:string[])
            n487 = call "File Dialog"("error in"=w889, "pattern (all files)"="*.cfg", "pattern label"="config") -> ("selected path"=w895:path, "error out"=w888:errorcluster)  [unwired: 9 in, 2 out]
            n488 = Bundle("CCDs"=w891, "move properties"=w893, "detection para"=w901, "thresholds"=w890, "Value"=w900) -> (w894:T5)  [unwired: 1 in]
            n489 = Open/Create/Replace File(file path (use dialog)=w895, error in=w888, operation (0:open)=T20."replace or create with confirmation") -> (refnum out=w902:refnum<file>, error out=w903:errorcluster)  [unwired: 3 in, 1 out]
            n490 = Write to Binary File(file (use dialog)=w902, data=w894, error in=w903) -> (refnum out=w905:refnum<file>, error out=w904:errorcluster)  [unwired: 3 in, 1 out]
            n491 = Close File(refnum=w905, error in=w904) -> (error out=w898:errorcluster)  [unwired: 1 out]
            n492 = call <vilib>:"Add State(s) to Queue__jki_lib_state_machine.vi"("State(s) in (\"\")"=w908) -> ("States Out"=w907:string)  [unwired: 14 in]
          }
          frame "active" {
            # "Your code here.\n(You can make a copy of, or modify, this frame)"
            n493 = call-poly <userlib>:"Filter 1D Array__ogtk.vi"("items to filter"=w918, "array"=w914) -> ("filtered item indices"=w917:i32[])  [unwired: 4 in, 1 out]
            n494 = Unbundle By Name(w913) -> ("move properties"=w916:T2[], "detection para"=w911:T3[])  [unwired: 1 out]
            n495 = Index Array(array=w917) -> (element=w909:i32)  [unwired: 1 in]
            n496 = Index Array(array=w916, index=w909) -> (element=w915:T2)
            n497 = Index Array(array=w911, index=w909) -> (element=w910:T3)
            n498 = property on="move config" class="Clust (strict)"("Value"=w915) -> ()  [unwired: 2 in, 2 out]
            n499 = property on="beam detection para" class="Clust (strict)"("Value"=w910) -> ()  [unwired: 2 in, 2 out]
            n500 = Bundle By Name(cluster=w913, "active ccd"=w909) -> (w912:T37)
            n501 = call <vilib>:"Add State(s) to Queue__jki_lib_state_machine.vi"("State(s) in (\"\")"=w921) -> ("States Out"=w920:string)  [unwired: 14 in]
          }
          frame "Detection Config" {
            # "Your code here.\n(You can make a copy of, or modify, this frame)"
            n502 = Unbundle By Name(w926) -> ("detection para"=w922:T3[], "active ccd"=w927:i32)
            n503 = Replace Array Subset(array=w922, new element="beam detection para", index=w927) -> (w923:T3[])
            n504 = Bundle By Name(cluster=w926, "detection para"=w923) -> (w925:T37)
            n505 = call <vilib>:"Add State(s) to Queue__jki_lib_state_machine.vi"("State(s) in (\"\")"=w930) -> ("States Out"=w929:string)  [unwired: 14 in]
          }
          frame "Motor Config" {
            # "Your code here.\n(You can make a copy of, or modify, this frame)"
            n506 = Unbundle By Name("associated motors") -> ("Motor CCD 1"=w952:u16, "Motor CCD 2"=w953:u16, "Motor CCD 3"=w954:u16, "Motor CCD 4"=w947:u16, "Motor CCD 5"=w946:u16, "Motor CCD 6"=w945:u16, "Motor CCD 7"=w944:u16, "Motor CCD 8"=w943:u16, "Motor CCD 9"=w942:u16, "Motor CCD 10"=w941:u16, "Motor CCD 11"=w940:u16, "Motor CCD 12"=w939:u16)
            n507 = local read "motor refs"() -> (w950:refnum<vi>[])
            n508 = property on="ActiveMotor" class="Ring (strict)"() -> ("Value"=w933:u16)  [unwired: 2 in, 2 out]
            n509 = property on="ActiveMotor" class="Ring (strict)"() -> ("Strings []"=w935:string[])  [unwired: 2 in, 2 out]
            n510 = Build Array(w952, w953, w954, w947, w946, w945, w944, w943, w942, w941, w940, w939) -> (w938:u16[])
            n511 = Increment(x=w938) -> (x+1=w937:u16[])
            n512 = Index Array(array=w935, index=w933) -> (element=w934:string)
            n513 = for {
              tunnel: w937 -> [w969] mode=indexing
              tunnel: w950 -> [w964]
              tunnel: [w960] -> w936 mode=indexing
              tunnel: [w959] -> w932 mode=indexing
              tunnel: [w958] -> w931 mode=indexing
              n514 = Multiply(x=w969, y=u16 3) -> (x*y=w965:u16)
              n515 = Subtract(x=w965, y=u16 3) -> (x-y=w959:u16)
              n516 = Subtract(x=w965, y=u16 2) -> (x-y=w958:u16)
              n517 = Index Array(array=w964, index=w959) -> (element=w963:refnum<vi>)
              n518 = Index Array(array=w964, index=w958) -> (element=w962:refnum<vi>)
              n519 = Bundle By Name(cluster="active Axis ref", "Ref X"=w963, "Ref Y"=w962) -> (w960:cluster{"Ref X":refnum<vi>, "Ref Y":refnum<vi>})
            }
            "Array" <- w932
            "Array 2" <- w931
            n520 = property on="ActiveMotorName::99" class="Str"("Val(Sgnl)"=w934) -> ()  [unwired: 2 in, 2 out]
            n521 = call <vilib>:"Add State(s) to Queue__jki_lib_state_machine.vi"("State(s) in (\"\")"=w957) -> ("States Out"=w956:string)  [unwired: 14 in]
            n522 = Bundle By Name(cluster=w949, "active axis refs 2"=w936) -> (w948:T37)
          }
          frame "Move Config" {
            # "Your code here.\n(You can make a copy of, or modify, this frame)"
            n523 = Unbundle By Name(w971) -> ("move properties"=w975:T2[], "active ccd"=w974:i32)
            n524 = Replace Array Subset(array=w975, new element="move config", index=w974) -> (w972:T2[])
            n525 = Bundle By Name(cluster=w971, "move properties"=w972) -> (w970:T37)
            n526 = call <vilib>:"Add State(s) to Queue__jki_lib_state_machine.vi"("State(s) in (\"\")"=w978) -> ("States Out"=w977:string)  [unwired: 14 in]
          }
          frame "----------Centroid & Move----------" {
            # "Template Separator\n(You can make a copy of, or modify, this frame)"
            n527 = call <vilib>:"Add State(s) to Queue__jki_lib_state_machine.vi"("State(s) in (\"\")"=w982) -> ("States Out"=w981:string)  [unwired: 14 in]
          }
          frame "detected" {
            n528 = Unbundle By Name(w985) -> ("Offset X"=w1027:dbl[][], "Offset Y"=w1026:dbl[][], "Size"=w1025:dbl[][], "Mean Size"=w1024:dbl[][], "Time"=w1021:timestamp[][], "Motor X"=w999:dbl[][], "active axis refs 2"=w998:T12, "Motor Y"=w997:dbl[][])
            n529 = Spreadsheet String To Array(format string="%s", spreadsheet string=w1003, array type (2D Dbl)=string[] []) -> (array=w992:string[])  [unwired: 1 in]
            n530 = call-poly <userlib>:"Filter 1D Array__ogtk.vi"("items to filter"=w992, "array"=w993) -> ("filtered item indices"=w990:i32[])  [unwired: 4 in, 1 out]
            n531 = for {
              tunnel: w993 -> [w1044] mode=indexing
              tunnel: w992 -> [w1043]
              tunnel: [w1041] -> w994 mode=indexing
              n532 = for {
                tunnel: w1044 -> [w1047]
                tunnel: [w1046] -> w1042 mode=indexing
                tunnel: w1043 -> [w1045] mode=indexing
                n533 = Equal?(x=w1047, y=w1045) -> (x = y?=w1046:bool)
              }
              n534 = Or Array Elements(Boolean array=w1042) -> (logical OR=w1041:bool)
            }
            n535 = for {
              N: 12 -> [_]
              tunnel: w990 -> [w1040]
              tunnel: [w1037] -> w989 mode=indexing
              i -> [w1039]
              n536 = Equal?(x=w1040, y=w1039) -> (x = y?=w1038:bool[])
              n537 = Or Array Elements(Boolean array=w1038) -> (logical OR=w1037:bool)
            }
            "Array 3" <- w989
            n538 = call <vilib>:"Build State String with Arguments__jki_lib_state_machine.vi"("Arguments (\"\")"=w1003, "State"="stats") -> ("State with Arguments"=w1002:string)  [unwired: 4 in]
            n539 = Unbundle By Name(w985) -> ("Mean Centroid X"=w1032:dbl[][], "Mean Centroid Y"=w1031:dbl[][], "Centroid X"=w1034:dbl[][], "Centroid Y"=w1033:dbl[][])
            n540 = call <vilib>:"Add State(s) to Queue__jki_lib_state_machine.vi"("State(s) in (\"\")"=w1001, "State(s) at Back (\"\")"=w1002) -> ("States Out"=w1000:string)  [unwired: 13 in]
            n541 = for {
              tunnel: w1034 -> [w1097]
              tunnel: w1033 -> [w1096]
              tunnel: w1032 -> [w1095]
              tunnel: w1031 -> [w1094]
              tunnel: [w1093] -> w1018 mode=indexing
              tunnel: [w1092] -> w1029 mode=indexing
              tunnel: w1028 -> [w1065] mode=indexing
              tunnel: w1027 -> [w1091]
              tunnel: w1026 -> [w1090]
              tunnel: [w1089] -> w1006 mode=indexing
              tunnel: [w1088] -> w1019 mode=indexing
              tunnel: w1025 -> [w1087]
              tunnel: w1024 -> [w1086]
              tunnel: [w1085] -> w1023 mode=indexing
              tunnel: w1021 -> [w1084]
              tunnel: [w1083] -> w1020 mode=indexing
              tunnel: w999 -> [w1057]
              tunnel: w998 -> [w1056]
              tunnel: w997 -> [w1055]
              tunnel: [w1054] -> w996 mode=indexing
              tunnel: [w1053] -> w995 mode=indexing
              tunnel: w994 -> [w1052]
              i -> [w1051]
              n542 = Unbundle By Name(w1065) -> ("Target.X::12"=w1068:refnum<vi>, "Target.Y::12"=w1067:refnum<vi>)
              n543 = Index Array(array=w1057, index (row)=w1051) -> (element=w1060:dbl[])  [unwired: 1 in]
              n544 = Index Array(array=w1056, index=w1051) -> (element=w1059:cluster{"Ref X":refnum<vi>, "Ref Y":refnum<vi>})
              n545 = Index Array(array=w1055, index (row)=w1051) -> (element=w1064:dbl[])  [unwired: 1 in]
              n546 = Index Array(array=w1095, index (row)=w1051) -> (element=w1079:dbl[])  [unwired: 1 in]
              n547 = Index Array(array=w1094, index (row)=w1051) -> (element=w1080:dbl[])  [unwired: 1 in]
              n548 = Index Array(array=w1097, index (row)=w1051) -> (element=w1082:dbl[])  [unwired: 1 in]
              n549 = Index Array(array=w1096, index (row)=w1051) -> (element=w1081:dbl[])  [unwired: 1 in]
              n550 = Index Array(array=w1091, index (row)=w1051) -> (element=w1076:dbl[])  [unwired: 1 in]
              n551 = Index Array(array=w1090, index (row)=w1051) -> (element=w1075:dbl[])  [unwired: 1 in]
              n552 = Index Array(array=w1087, index (row)=w1051) -> (element=w1073:dbl[])  [unwired: 1 in]
              n553 = Index Array(array=w1086, index (row)=w1051) -> (element=w1072:dbl[])  [unwired: 1 in]
              n554 = Index Array(array=w1084, index (row)=w1051) -> (element=w1069:timestamp[])  [unwired: 1 in]
              n555 = Index Array(array=w1052, index=w1051) -> (element=w1050:bool)
              n556 = Unbundle By Name(w1059) -> ("Ref X"=w1058:refnum<vi>, "Ref Y"=w1062:refnum<vi>)
              n557 = property class="DigNum (strict)"(reference=w1068) -> ("Value"=w1049:dbl)  [unwired: 1 in, 2 out]
              n558 = property class="DigNum (strict)"(reference=w1067) -> ("Value"=w1066:dbl)  [unwired: 1 in, 2 out]
              n559 = call <vilib>:"Std Deviation and Variance.vi"("X"=w1082) -> ("mean"=w1048:dbl)  [unwired: 1 in, 2 out]
              n560 = call <vilib>:"Std Deviation and Variance.vi"("X"=w1081) -> ("mean"=w1078:dbl)  [unwired: 1 in, 2 out]
              n561 = call <vilib>:"Std Deviation and Variance.vi"("X"=w1073) -> ("mean"=w1071:dbl)  [unwired: 1 in, 2 out]
              n562 = Get Date/Time In Seconds() -> (seconds since 1Jan1904=w1070:timestamp)
              n563 = property class="DigNum (strict)"(reference=w1058) -> ("Value"=w1061:dbl)  [unwired: 1 in, 2 out]
              n564 = property class="DigNum (strict)"(reference=w1062) -> ("Value"=w1063:dbl)  [unwired: 1 in, 2 out]
              n565 = Subtract(x=w1049, y=w1048) -> (x-y=w1077:dbl)
              n566 = Subtract(x=w1066, y=w1078) -> (x-y=w1074:dbl)
              n567 = case shown="True" w1050 {
                tunnel: [w1115 w1129] -> w1093
                tunnel: [w1114 w1128] -> w1092
                tunnel: [w1113 w1127] -> w1089
                tunnel: [w1112 w1126] -> w1088
                tunnel: [w1111 w1125] -> w1085
                tunnel: [w1110 w1124] -> w1083
                tunnel: w1080 -> [w1109 w1123]
                tunnel: w1079 -> [w1108 w1122]
                tunnel: w1048 -> [w1107 _]
                tunnel: w1078 -> [w1106 _]
                tunnel: w1077 -> [w1105 _]
                tunnel: w1076 -> [w1104 w1121]
                tunnel: w1075 -> [w1103 w1120]
                tunnel: w1074 -> [w1102 _]
                tunnel: w1072 -> [w1101 w1119]
                tunnel: w1071 -> [w1100 _]
                tunnel: w1070 -> [w1099 w1118]
                tunnel: w1069 -> [w1098 w1117]
                frame True {
                  n568 = Build Array (concatenate)(w1108, w1107) -> (w1115:dbl[])
                  n569 = Build Array (concatenate)(w1109, w1106) -> (w1114:dbl[])
                  n570 = Build Array (concatenate)(w1104, w1105) -> (w1113:dbl[])
                  n571 = Build Array (concatenate)(w1103, w1102) -> (w1112:dbl[])
                  n572 = Build Array (concatenate)(w1101, w1100) -> (w1111:dbl[])
                  n573 = Build Array (concatenate)(w1098, w1099) -> (w1110:timestamp[])
                }
                frame False {
                  w1116 = 0.0
                  n574 = Build Array (concatenate)(w1122, w1116) -> (w1129:dbl[])
                  n575 = Build Array (concatenate)(w1123, w1116) -> (w1128:dbl[])
                  n576 = Build Array (concatenate)(w1121, w1116) -> (w1127:dbl[])
                  n577 = Build Array (concatenate)(w1120, w1116) -> (w1126:dbl[])
                  n578 = Build Array (concatenate)(w1119, w1116) -> (w1125:dbl[])
                  n579 = Build Array (concatenate)(w1117, w1118) -> (w1124:timestamp[])
                }
              }
              n580 = Build Array (concatenate)(w1064, w1063) -> (w1053:dbl[])
              n581 = Build Array (concatenate)(w1060, w1061) -> (w1054:dbl[])
            }
            n582 = local write "Numeric"(0.0 ("Numeric")) -> ()
            n583 = Array Size(array=w1006) -> (size(s)=w1017:i32[])
            n584 = Index Array(array=w1017, index=1) -> (element=w1015:i32)
            "History index" <- w1015
            n585 = call <vilib>:"Add State(s) to Queue__jki_lib_state_machine.vi"("State(s) in (\"\")"=w1000, "State(s) at Back (\"\")"="Check Move\ntdms" ("State(s) at Back (\"\")")) -> ("States Out"=w1009:string)  [unwired: 13 in]
            n586 = Unbundle By Name(w985) -> ("img to avg"=w984:i32)
            n587 = Decrement(x=w984) -> (x-1=w983:i32)
            n588 = Initialize Array(0.0 ("element"), 12 ("dimension size"), w983) -> (w986:dbl[][])
            n589 = Greater?(x=w1015, y="History Size") -> (0:w1013:bool)
            n590 = Bundle By Name(cluster=w985, "Centroid X"=w986, "Centroid Y"=w986, "Mean Centroid X"=w1018, "Mean Centroid Y"=w1029, "Offset X"=w1006, "Offset Y"=w1019, "Mean Size"=w1023, "Size"=w986, "Time"=w1020, "Motor X"=w996, "Motor Y"=w995) -> (w1030:T37)
            n591 = Select(t="history" ("State(s) at Back (\"\")"), s=w1013, f="") -> (s? t:f=w1010:string)
            n592 = call <vilib>:"Add State(s) to Queue__jki_lib_state_machine.vi"("State(s) in (\"\")"=w1009, "State(s) at Back (\"\")"=w1010) -> ("States Out"=w1008:string)  [unwired: 13 in]
          }
          frame "Check Move" {
            (unwired) "Device Ini" ("State(s) in Front (\"\")")
            # "Your code here.\n(You can make a copy of, or modify, this frame)"
            n593 = Unbundle By Name(w1134) -> ("move properties"=w1137:T2[], "Mean Size"=w1160:dbl[][], "move properties"=w1163:T2[], "Offset X"=w1162:dbl[][], "Offset Y"=w1161:dbl[][], "active cams"=w1141:string[])
            n594 = for {
              tunnel: w1163 -> [w1228]
              tunnel: w1162 -> [w1227]
              tunnel: w1161 -> [w1226]
              tunnel: w1160 -> [w1229]
              tunnel: [w1245] -> w1159 mode=indexing
              tunnel: [w1241] -> w1158 mode=indexing
              tunnel: w1141 -> [w1231] mode=indexing
              tunnel: [w1263] -> w1157 mode=indexing
              tunnel: [w1262] -> w1156 mode=indexing
              tunnel: w1137 -> [w1221]
              tunnel: [w1239] -> w1135 mode=indexing
              tunnel: [w1234] -> w1131 mode=indexing
              tunnel: "Speedmode @" -> [w1233]
              tunnel: w1130 -> [w1232]
              n595 = call-poly <userlib>:"Filter 1D Array__ogtk.vi"("items to filter"=w1231, "array"=w1232) -> ("filtered item indices"=w1230:i32[])  [unwired: 4 in, 1 out]
              n596 = Index Array(array=w1230) -> (element=w1220:i32)  [unwired: 1 in]
              n597 = Index Array(array=w1229, index (row)=w1220) -> (element=w1225:dbl[])  [unwired: 1 in]
              n598 = Index Array(array=w1228, index=w1220) -> (element=w1224:T2)
              n599 = Index Array(array=w1227, index (row)=w1220) -> (element=w1223:dbl[])  [unwired: 1 in]
              n600 = Index Array(array=w1221, index=w1220) -> (element=w1219:T2)
              n601 = Index Array(array=w1226, index (row)=w1220) -> (element=w1222:dbl[])  [unwired: 1 in]
              n602 = Unbundle By Name(w1224) -> ("Tolerance [%]"=w1256:dbl)
              n603 = Reverse 1D Array(array=w1223) -> (reversed array=w1261:dbl[])
              n604 = Reverse 1D Array(array=w1222) -> (reversed array=w1260:dbl[])
              n605 = Reverse 1D Array(array=w1225) -> (reversed array=w1255:dbl[])
              n606 = Unbundle By Name(w1219) -> ("enable feedback"=w1244:bool)
              n607 = Index Array(array=w1261) -> (element=w1259:dbl)  [unwired: 1 in]
              n608 = Index Array(array=w1260) -> (element=w1258:dbl)  [unwired: 1 in]
              n609 = Index Array(array=w1255) -> (element=w1254:dbl)  [unwired: 1 in]
              n610 = Absolute Value(x=w1259) -> (abs(x)=w1240:dbl)
              n611 = Absolute Value(x=w1258) -> (abs(x)=w1237:dbl)
              n612 = Square Root(x=w1254) -> (sqrt(x)=w1253:dbl)
              n613 = Divide(x=w1256, y=100.0) -> (x/y=w1252:dbl)
              n614 = Multiply(x=w1253, y=w1252) -> (x*y=w1236:dbl)
              n615 = Not Equal To 0?(x=w1237) -> (x != 0?=w1242:bool)
              n616 = Not Equal To 0?(x=w1240) -> (x != 0?=w1247:bool)
              n617 = Greater Or Equal?(x=w1240, y=w1236) -> (x >= y?=w1246:bool)
              n618 = Greater Or Equal?(x=w1237, y=w1236) -> (x >= y?=w1243:bool)
              n619 = Divide(x=w1240, y=w1236) -> (x/y=w1238:dbl)
              n620 = Divide(x=w1237, y=w1236) -> (x/y=w1235:dbl)
              n621 = Compound Arithmetic op=AND(w1244, w1247, w1246) -> (w1245:bool)
              n622 = Compound Arithmetic op=AND(w1244, w1243, w1242) -> (w1241:bool)
              n623 = Boolean To (0,1)(Boolean=w1241) -> (0, 1=w1248:i16)
              n624 = Greater?(x=w1238, y=w1233) -> (0:w1239:bool)
              n625 = Greater?(x=w1235, y=w1233) -> (0:w1234:bool)
              n626 = Multiply(x=w1248, y=w1237) -> (x*y=w1249:dbl)
              n627 = Boolean To (0,1)(Boolean=w1245) -> (0, 1=w1251:i16)
              n628 = Multiply(x=w1251, y=w1240) -> (x*y=w1250:dbl)
              n629 = Bundle(w1249, "GUIdevice 8"=w1231) -> (w1262:cluster{dbl, "GUIdevice 8":string})  [unwired: 1 in]
              n630 = Bundle(w1250, "GUIdevice 8"=w1231) -> (w1263:cluster{dbl, "GUIdevice 8":string})  [unwired: 1 in]
            }
            "required X" <- w1159
            "required Y" <- w1158
            "speedmode X" <- w1135
            "speedmode Y" <- w1131
            n631 = case shown="True" "Align" {
              tunnel: w1157 -> [w1171 w1176]
              tunnel: w1156 -> [w1170 w1173]
              tunnel: [w1169 w1175] -> w1153
              tunnel: [w1168 w1172] -> w1147
              frame False {
                n632 = Sort 1D Array(array=w1170) -> (sorted array=w1167:cluster{dbl, "GUIdevice 8":string}[])
                n633 = Sort 1D Array(array=w1171) -> (sorted array=w1166:cluster{dbl, "GUIdevice 8":string}[])
                n634 = Reverse 1D Array(array=w1167) -> (reversed array=w1168:cluster{dbl, "GUIdevice 8":string}[])
                n635 = Reverse 1D Array(array=w1166) -> (reversed array=w1169:cluster{dbl, "GUIdevice 8":string}[])
              }
              frame True {
                w1174 = cluster{dbl, "GUIdevice 8":string}[] [] ("Array")
                n636 = for {
                  shift-right: [w1186] -> w1175
                  shift-left: w1174 -> [w1188]
                  tunnel: w1176 -> [w1187] mode=indexing
                  n637 = Unbundle(w1187) -> (w1190:dbl)  [unwired: 1 out]
                  n638 = Not Equal To 0?(x=w1190) -> (x != 0?=w1189:bool)
                  n639 = case shown="True" w1189 {
                    tunnel: w1188 -> [w1191 w1194]
                    tunnel: w1187 -> [_ w1193]
                    tunnel: [w1191 w1192] -> w1186
                    frame False {
                    }
                    frame True {
                      n640 = Build Array (concatenate)(w1194, w1193) -> (w1192:cluster{dbl, "GUIdevice 8":string}[])
                    }
                  }
                }
                n641 = for {
                  shift-right: [w1177] -> w1172
                  shift-left: w1174 -> [w1179]
                  tunnel: w1173 -> [w1178] mode=indexing
                  n642 = Unbundle(w1178) -> (w1181:dbl)  [unwired: 1 out]
                  n643 = Not Equal To 0?(x=w1181) -> (x != 0?=w1180:bool)
                  n644 = case shown="True" w1180 {
                    tunnel: w1179 -> [w1182 w1185]
                    tunnel: w1178 -> [_ w1184]
                    tunnel: [w1182 w1183] -> w1177
                    frame False {
                    }
                    frame True {
                      n645 = Build Array (concatenate)(w1185, w1184) -> (w1183:cluster{dbl, "GUIdevice 8":string}[])
                    }
                  }
                }
              }
            }
            n646 = call <vilib>:"Add State(s) to Queue__jki_lib_state_machine.vi"("State(s) in (\"\")"=w1140) -> ("States Out"=w1139:string)  [unwired: 14 in]
            n647 = Bundle By Name(cluster=w1134, "speedmode X"=w1135, "speedmode Y"=w1131) -> (w1133:T37)
            n648 = Empty Array?(array=w1153) -> (empty?=w1150:bool)
            n649 = Empty Array?(array=w1147) -> (empty?=w1145:bool)
            n650 = Index Array(array=w1153) -> (element=w1143:cluster{dbl, "GUIdevice 8":string})  [unwired: 1 in]
            n651 = Index Array(array=w1147) -> (element=w1142:cluster{dbl, "GUIdevice 8":string})  [unwired: 1 in]
            n652 = Unbundle(w1143) -> (w1152:dbl)  [unwired: 1 out]
            n653 = Unbundle(w1142) -> (w1148:dbl)  [unwired: 1 out]
            n654 = Equal To 0?(x=w1152) -> (x = 0?=w1151:bool)
            n655 = Equal To 0?(x=w1148) -> (x = 0?=w1146:bool)
            n656 = property on="autodetect" class="Bool (strict)"("Value"=FALSE ("autodetect")) -> ()  [unwired: 2 in, 2 out]
            n657 = Unbundle By Name(w1133) -> ("Feedback global"=w1154:bool)
            n658 = Or(x=w1151, y=w1150) -> (x .or. y?=w1149:bool)
            n659 = Or(x=w1146, y=w1145) -> (x .or. y?=w1144:bool)
            n660 = case shown="True" w1154 {
              tunnel: w1149 -> [_ w1202]
              tunnel: w1153 -> [_ w1201]
              tunnel: w1144 -> [_ w1199]
              tunnel: w1147 -> [_ w1198]
              tunnel: w1139 -> [w1195 w1197]
              tunnel: [w1195 w1196] -> w1155
              frame False {
              }
              frame True {
                n661 = case shown="False" w1202 {
                  tunnel: w1201 -> [w1217 _]
                  tunnel: w1197 -> [w1213 w1218]
                  tunnel: [w1211 w1218] -> w1200
                  frame False {
                    n662 = Index Array(array=w1217) -> (element=w1216:cluster{dbl, "GUIdevice 8":string})  [unwired: 1 in]
                    n663 = Unbundle By Name(w1216) -> ("GUIdevice 8"=w1215:string)
                    n664 = call <vilib>:"Build State String with Arguments__jki_lib_state_machine.vi"("Arguments (\"\")"=w1215, "State"="Move X") -> ("State with Arguments"=w1212:string)  [unwired: 4 in]
                    n665 = call <vilib>:"Add State(s) to Queue__jki_lib_state_machine.vi"("State(s) in (\"\")"=w1213, "State(s) at Back (\"\")"=w1212) -> ("States Out"=w1211:string)  [unwired: 13 in]
                  }
                  frame True {
                  }
                }
                n666 = case shown="False" w1199 {
                  tunnel: w1198 -> [w1209 _]
                  tunnel: w1200 -> [w1205 w1210]
                  tunnel: [w1203 w1210] -> w1196
                  frame False {
                    n667 = Index Array(array=w1209) -> (element=w1208:cluster{dbl, "GUIdevice 8":string})  [unwired: 1 in]
                    n668 = Unbundle By Name(w1208) -> ("GUIdevice 8"=w1207:string)
                    n669 = call <vilib>:"Build State String with Arguments__jki_lib_state_machine.vi"("Arguments (\"\")"=w1207, "State"="Move Y") -> ("State with Arguments"=w1204:string)  [unwired: 4 in]
                    n670 = call <vilib>:"Add State(s) to Queue__jki_lib_state_machine.vi"("State(s) in (\"\")"=w1205, "State(s) at Back (\"\")"=w1204) -> ("States Out"=w1203:string)  [unwired: 13 in]
                  }
                  frame True {
                  }
                }
              }
            }
            n671 = call <vilib>:"Add State(s) to Queue__jki_lib_state_machine.vi"("State(s) in (\"\")"=w1139, "State(s) at Back (\"\")"=w1155) -> ("States Out"=w1165:string)  [unwired: 13 in]
          }
          frame "Move X" {
            # "Your code here.\n(You can make a copy of, or modify, this frame)"
            n672 = Unbundle By Name(w1287) -> ("Offset X"=w1264:dbl[][])
            n673 = call-poly <userlib>:"Filter 1D Array__ogtk.vi"("items to filter"=w1272, "array"=w1291) -> ("filtered item indices"=w1276:i32[])  [unwired: 4 in, 1 out]
            n674 = Unbundle By Name(w1287) -> ("speedmode X"=w1271:bool[], "active axis refs 2"=w1290:T12, "move properties"=w1275:T2[])
            n675 = for {
              tunnel: w1276 -> [w1296] mode=indexing
              tunnel: w1275 -> [w1300]
              shift-right: [w1295] -> w1273
              shift-left: i32[] [] ("filtered item indices") -> [w1298]
              n676 = Index Array(array=w1300, index=w1296) -> (element=w1299:T2)
              n677 = Unbundle By Name(w1299) -> ("enable feedback"=w1297:bool)
              n678 = case shown="True" w1297 {
                tunnel: w1298 -> [w1301 w1304]
                tunnel: w1296 -> [_ w1303]
                tunnel: [w1301 w1302] -> w1295
                frame False {
                }
                frame True {
                  n679 = Build Array (concatenate)(w1304, w1303) -> (w1302:i32[])
                }
              }
            }
            n680 = Index Array(array=w1273) -> (element=w1270:i32)  [unwired: 1 in]
            n681 = Index Array(array=w1264, index (row)=w1270) -> (element=w1286:dbl[])  [unwired: 1 in]
            n682 = Reverse 1D Array(array=w1286) -> (reversed array=w1285:dbl[])
            n683 = Index Array(array=w1290, index=w1270) -> (element=w1289:cluster{"Ref X":refnum<vi>, "Ref Y":refnum<vi>})
            n684 = Index Array(array=w1285) -> (element=w1283:dbl)  [unwired: 1 in]
            n685 = Index Array(array=w1275, index=w1270) -> (element=w1288:T2)
            n686 = Unbundle By Name(w1289) -> ("Ref X"=w1280:refnum<vi>, "Ref Y"=w1279:refnum<vi>)
            n687 = Index Array(array=w1271, index=w1270) -> (element=w1269:bool)
            n688 = Unbundle By Name(w1288) -> ("Invert Direction X"=w1281:bool, "Invert Axis"=w1284:bool, "Stepsize"=w1267:dbl, "enable feedback"=w1278:bool)
            n689 = Greater Or Equal To 0?(x=w1283) -> (x >= 0?=w1282:bool)
            n690 = call <vilib>:"Add State(s) to Queue__jki_lib_state_machine.vi"("State(s) in Front (\"\")"="Wait" ("State(s) in Front (\"\")"), "State(s) in (\"\")"=w1294) -> ("States Out"=w1293:string)  [unwired: 13 in]
            n691 = property on="Speedmode @" class="DigNum (strict)"() -> ("Value"=w1266:dbl)  [unwired: 2 in, 2 out]
            n692 = Multiply(x=w1266, y=w1267) -> (x*y=w1268:dbl)
            n693 = Select(t=w1268, s=w1269, f=w1267) -> (s? t:f=w1265:dbl)
            n694 = case shown="True" w1278 {
              tunnel: w1284 -> [_ w1310]
              tunnel: w1282 -> [_ w1309]
              tunnel: w1265 -> [_ w1308]
              tunnel: w1281 -> [_ w1307]
              tunnel: w1280 -> [_ w1306]
              tunnel: w1279 -> [_ w1305]
              frame False {
              }
              frame True {
                n695 = case shown="False" w1309 {
                  tunnel: w1307 -> [w1318 w1340]
                  tunnel: w1308 -> [w1316 w1338]
                  tunnel: w1310 -> [w1315 w1337]
                  tunnel: w1310 -> [w1314 w1336]
                  tunnel: w1306 -> [w1312 w1334]
                  tunnel: w1305 -> [w1311 w1333]
                  frame True {
                    n696 = case shown="False" w1315 {
                      tunnel: [w1329 w1331] -> w1317
                      tunnel: w1312 -> [w1330 _]
                      tunnel: w1311 -> [_ w1332]
                      frame False {
                        n697 = property class="DigNum (strict)"(reference=w1330) -> ("Value"=w1329:dbl)  [unwired: 1 in, 2 out]
                      }
                      frame True {
                        n698 = property class="DigNum (strict)"(reference=w1332) -> ("Value"=w1331:dbl)  [unwired: 1 in, 2 out]
                      }
                    }
                    n699 = case shown="False" w1318 {
                      tunnel: w1317 -> [w1325 w1328]
                      tunnel: w1316 -> [w1324 w1327]
                      tunnel: [w1323 w1326] -> w1313
                      frame False {
                        n700 = Add(x=w1325, y=w1324) -> (x+y=w1323:dbl)
                      }
                      frame True {
                        n701 = Subtract(x=w1328, y=w1327) -> (x-y=w1326:dbl)
                      }
                    }
                    n702 = case shown="False" w1314 {
                      tunnel: w1313 -> [w1319 w1321]
                      tunnel: w1312 -> [w1320 _]
                      tunnel: w1311 -> [_ w1322]
                      frame False {
                        n703 = property class="DigNum (strict)"(reference=w1320, "Val(Sgnl)"=w1319) -> ()  [unwired: 1 in, 2 out]
                      }
                      frame True {
                        n704 = property class="DigNum (strict)"(reference=w1322, "Val(Sgnl)"=w1321) -> ()  [unwired: 1 in, 2 out]
                      }
                    }
                  }
                  frame False {
                    n705 = case shown="False" w1337 {
                      tunnel: [w1351 w1353] -> w1339
                      tunnel: w1334 -> [w1352 _]
                      tunnel: w1333 -> [_ w1354]
                      frame False {
                        n706 = property class="DigNum (strict)"(reference=w1352) -> ("Value"=w1351:dbl)  [unwired: 1 in, 2 out]
                      }
                      frame True {
                        n707 = property class="DigNum (strict)"(reference=w1354) -> ("Value"=w1353:dbl)  [unwired: 1 in, 2 out]
                      }
                    }
                    n708 = case shown="False" w1340 {
                      tunnel: w1339 -> [w1347 w1350]
                      tunnel: w1338 -> [w1346 w1349]
                      tunnel: [w1345 w1348] -> w1335
                      frame False {
                        n709 = Subtract(x=w1347, y=w1346) -> (x-y=w1345:dbl)
                      }
                      frame True {
                        n710 = Add(x=w1350, y=w1349) -> (x+y=w1348:dbl)
                      }
                    }
                    n711 = case shown="False" w1336 {
                      tunnel: w1335 -> [w1341 w1343]
                      tunnel: w1334 -> [w1342 _]
                      tunnel: w1333 -> [_ w1344]
                      frame False {
                        n712 = property class="DigNum (strict)"(reference=w1342, "Val(Sgnl)"=w1341) -> ()  [unwired: 1 in, 2 out]
                      }
                      frame True {
                        n713 = property class="DigNum (strict)"(reference=w1344, "Val(Sgnl)"=w1343) -> ()  [unwired: 1 in, 2 out]
                      }
                    }
                  }
                }
              }
            }
            "Arguments X" <- w1272
            "Moving X" <- w1272
          }
          frame "Move Y" {
            # "Your code here.\n(You can make a copy of, or modify, this frame)"
            n714 = Unbundle By Name(w1378) -> ("Offset Y"=w1377:dbl[][])
            n715 = call-poly <userlib>:"Filter 1D Array__ogtk.vi"("items to filter"=w1362, "array"=w1382) -> ("filtered item indices"=w1367:i32[])  [unwired: 4 in, 1 out]
            n716 = Unbundle By Name(w1378) -> ("speedmode Y"=w1361:bool[], "active axis refs 2"=w1381:T12, "move properties"=w1365:T2[])
            n717 = for {
              tunnel: w1367 -> [w1387] mode=indexing
              tunnel: w1365 -> [w1391]
              shift-right: [w1386] -> w1366
              shift-left: i32[] [] ("filtered item indices") -> [w1389]
              n718 = Index Array(array=w1391, index=w1387) -> (element=w1390:T2)
              n719 = Unbundle By Name(w1390) -> ("enable feedback"=w1388:bool)
              n720 = case shown="True" w1388 {
                tunnel: w1389 -> [w1392 w1395]
                tunnel: w1387 -> [_ w1394]
                tunnel: [w1392 w1393] -> w1386
                frame False {
                }
                frame True {
                  n721 = Build Array (concatenate)(w1395, w1394) -> (w1393:i32[])
                }
              }
            }
            n722 = Index Array(array=w1366) -> (element=w1360:i32)  [unwired: 1 in]
            n723 = Index Array(array=w1377, index (row)=w1360) -> (element=w1376:dbl[])  [unwired: 1 in]
            n724 = Reverse 1D Array(array=w1376) -> (reversed array=w1375:dbl[])
            n725 = Index Array(array=w1381, index=w1360) -> (element=w1380:cluster{"Ref X":refnum<vi>, "Ref Y":refnum<vi>})
            n726 = Index Array(array=w1375) -> (element=w1373:dbl)  [unwired: 1 in]
            n727 = Index Array(array=w1365, index=w1360) -> (element=w1379:T2)
            n728 = Index Array(array=w1361, index=w1360) -> (element=w1359:bool)
            n729 = Unbundle By Name(w1380) -> ("Ref Y"=w1370:refnum<vi>, "Ref X"=w1369:refnum<vi>)
            n730 = Unbundle By Name(w1379) -> ("Invert Direction Y"=w1371:bool, "Invert Axis"=w1374:bool, "Stepsize"=w1357:dbl, "enable feedback"=w1368:bool)
            n731 = Greater Or Equal To 0?(x=w1373) -> (x >= 0?=w1372:bool)
            n732 = call <vilib>:"Add State(s) to Queue__jki_lib_state_machine.vi"("State(s) in Front (\"\")"="Wait" ("State(s) in Front (\"\")"), "State(s) in (\"\")"=w1385) -> ("States Out"=w1384:string)  [unwired: 13 in]
            n733 = property on="Speedmode @" class="DigNum (strict)"() -> ("Value"=w1356:dbl)  [unwired: 2 in, 2 out]
            n734 = Multiply(x=w1356, y=w1357) -> (x*y=w1355:dbl)
            n735 = Select(t=w1355, s=w1359, f=w1357) -> (s? t:f=w1358:dbl)
            n736 = case shown="True" w1368 {
              tunnel: w1374 -> [_ w1401]
              tunnel: w1372 -> [_ w1400]
              tunnel: w1358 -> [_ w1399]
              tunnel: w1371 -> [_ w1398]
              tunnel: w1370 -> [_ w1397]
              tunnel: w1369 -> [_ w1396]
              frame False {
              }
              frame True {
                n737 = case shown="True" w1400 {
                  tunnel: w1398 -> [w1409 w1431]
                  tunnel: w1399 -> [w1407 w1429]
                  tunnel: w1401 -> [w1406 w1428]
                  tunnel: w1401 -> [w1405 w1427]
                  tunnel: w1397 -> [w1403 w1425]
                  tunnel: w1396 -> [w1402 w1424]
                  frame True {
                    n738 = case shown="False" w1406 {
                      tunnel: [w1420 w1422] -> w1408
                      tunnel: w1403 -> [w1421 _]
                      tunnel: w1402 -> [_ w1423]
                      frame False {
                        n739 = property class="DigNum (strict)"(reference=w1421) -> ("Value"=w1420:dbl)  [unwired: 1 in, 2 out]
                      }
                      frame True {
                        n740 = property class="DigNum (strict)"(reference=w1423) -> ("Value"=w1422:dbl)  [unwired: 1 in, 2 out]
                      }
                    }
                    n741 = case shown="False" w1409 {
                      tunnel: w1408 -> [w1416 w1419]
                      tunnel: w1407 -> [w1415 w1418]
                      tunnel: [w1414 w1417] -> w1404
                      frame False {
                        n742 = Add(x=w1416, y=w1415) -> (x+y=w1414:dbl)
                      }
                      frame True {
                        n743 = Subtract(x=w1419, y=w1418) -> (x-y=w1417:dbl)
                      }
                    }
                    n744 = case shown="False" w1405 {
                      tunnel: w1404 -> [w1410 w1412]
                      tunnel: w1403 -> [w1411 _]
                      tunnel: w1402 -> [_ w1413]
                      frame False {
                        n745 = property class="DigNum (strict)"(reference=w1411, "Val(Sgnl)"=w1410) -> ()  [unwired: 1 in, 2 out]
                      }
                      frame True {
                        n746 = property class="DigNum (strict)"(reference=w1413, "Val(Sgnl)"=w1412) -> ()  [unwired: 1 in, 2 out]
                      }
                    }
                  }
                  frame False {
                    n747 = case shown="False" w1428 {
                      tunnel: [w1442 w1444] -> w1430
                      tunnel: w1425 -> [w1443 _]
                      tunnel: w1424 -> [_ w1445]
                      frame False {
                        n748 = property class="DigNum (strict)"(reference=w1443) -> ("Value"=w1442:dbl)  [unwired: 1 in, 2 out]
                      }
                      frame True {
                        n749 = property class="DigNum (strict)"(reference=w1445) -> ("Value"=w1444:dbl)  [unwired: 1 in, 2 out]
                      }
                    }
                    n750 = case shown="False" w1431 {
                      tunnel: w1430 -> [w1438 w1441]
                      tunnel: w1429 -> [w1437 w1440]
                      tunnel: [w1436 w1439] -> w1426
                      frame False {
                        n751 = Subtract(x=w1438, y=w1437) -> (x-y=w1436:dbl)
                      }
                      frame True {
                        n752 = Add(x=w1441, y=w1440) -> (x+y=w1439:dbl)
                      }
                    }
                    n753 = case shown="False" w1427 {
                      tunnel: w1426 -> [w1432 w1434]
                      tunnel: w1425 -> [w1433 _]
                      tunnel: w1424 -> [_ w1435]
                      frame False {
                        n754 = property class="DigNum (strict)"(reference=w1433, "Val(Sgnl)"=w1432) -> ()  [unwired: 1 in, 2 out]
                      }
                      frame True {
                        n755 = property class="DigNum (strict)"(reference=w1435, "Val(Sgnl)"=w1434) -> ()  [unwired: 1 in, 2 out]
                      }
                    }
                  }
                }
              }
            }
            "Arguments Y" <- w1362
            "Moving Y" <- w1362
          }
          frame "Wait" {
            # "Your code here.\n(You can make a copy of, or modify, this frame)"
            n756 = flat-sequence {
              frame #0 {
                n757 = Wait (ms)(milliseconds to wait=u32 300) -> ()  [unwired: 1 out]
              }
              frame #1 {
                n758 = property on="Moving Y" class="Str"("Value"="") -> ()  [unwired: 2 in, 2 out]
                n759 = property on="Moving X" class="Str"("Value"="") -> ()  [unwired: 2 in, 2 out]
              }
            }
            n760 = call <vilib>:"Add State(s) to Queue__jki_lib_state_machine.vi"("State(s) in (\"\")"=w1451) -> ("States Out"=w1450:string)  [unwired: 14 in]
            n761 = local read "Mean Centroid X"() -> (w1446:dbl[][])
            n762 = Bundle By Name(cluster=w1448, "Mean Centroid X"=w1446, "Mean Centroid Y"=w1446) -> (w1447:T37)
          }
          frame "stats" {
            # "Your code here.\n(You can make a copy of, or modify, this frame)"
            n763 = Unbundle By Name(w1460) -> ("Offset X"=w1459:dbl[][], "Offset Y"=w1458:dbl[][], "Time"=w1457:timestamp[][], "Motor X"=w1456:dbl[][], "Motor Y"=w1455:dbl[][])
            n764 = for {
              tunnel: w1458 -> [w1498]
              tunnel: w1457 -> [w1499]
              tunnel: w1459 -> [w1500]
              tunnel: [w1503] -> w1486 mode=indexing
              tunnel: w1456 -> [w1497]
              tunnel: w1455 -> [w1496]
              tunnel: w1461 -> [_] mode=indexing
              i -> [w1490]
              n765 = Index Array(array=w1498, index (row)=w1490) -> (element=w1494:dbl[])  [unwired: 1 in]
              n766 = Index Array(array=w1497, index (row)=w1490) -> (element=w1492:dbl[])  [unwired: 1 in]
              n767 = Index Array(array=w1496, index (row)=w1490) -> (element=w1491:dbl[])  [unwired: 1 in]
              n768 = Index Array(array=w1500, index (row)=w1490) -> (element=w1495:dbl[])  [unwired: 1 in]
              n769 = Index Array(array=w1499, index (row)=w1490) -> (element=w1493:timestamp[])  [unwired: 1 in]
              n770 = Bundle("Time"=w1493, "Motor X"=w1492) -> (w1502:cluster{"Time":timestamp[], "Motor X":dbl[]})  [unwired: 1 in]
              n771 = Bundle("Time"=w1493, "Motor Y"=w1491) -> (w1501:cluster{"Time":timestamp[], "Motor Y":dbl[]})  [unwired: 1 in]
              n772 = Bundle("Time"=w1493, "Offset X"=w1495) -> (w1504:cluster{"Time":timestamp[], "Offset X":dbl[]})  [unwired: 1 in]
              n773 = Bundle("Time"=w1493, "Offset Y"=w1494) -> (w1505:cluster{"Time":timestamp[], "Offset Y":dbl[]})  [unwired: 1 in]
              n774 = Build Array(w1505, w1504, w1502, w1501) -> (w1503:cluster{"Time":timestamp[], "Motor Y":dbl[]}[])
            }
            n775 = call <vilib>:"Add State(s) to Queue__jki_lib_state_machine.vi"("State(s) in (\"\")"=w1489) -> ("States Out"=w1488:string)  [unwired: 14 in]
            n776 = Index Array(array=w1486, index (row) #1=0 ("index (row)"), index (row) #2=1 ("index (row)"), index (row) #3=2 ("index (row)"), index (row) #4=3 ("index (row)"), index (row) #5=4 ("index (row)"), index (row) #6=5 ("index (row)"), index (row) #7=6 ("index (row)"), index (row) #8=7 ("index (row)"), index (row) #9=8 ("index (row)"), index (row) #10=9 ("index (row)"), index (row) #11=10 ("index (row)"), index (row) #12=11 ("index (row)")) -> (element #1=→"CCD 1":cluster{"Time":timestamp[], "Motor Y":dbl[]}[], element #2=→"CCD 2":cluster{"Time":timestamp[], "Motor Y":dbl[]}[], element #3=→"CCD 3":cluster{"Time":timestamp[], "Motor Y":dbl[]}[], element #4=→"CCD 4":cluster{"Time":timestamp[], "Motor Y":dbl[]}[], element #5=→"CCD 5":cluster{"Time":timestamp[], "Motor Y":dbl[]}[], element #6=→"CCD 6":cluster{"Time":timestamp[], "Motor Y":dbl[]}[], element #7=→"CCD 7":cluster{"Time":timestamp[], "Motor Y":dbl[]}[], element #8=→"CCD 8":cluster{"Time":timestamp[], "Motor Y":dbl[]}[], element #9=→"CCD 9":cluster{"Time":timestamp[], "Motor Y":dbl[]}[], element #10=→"CCD 10":cluster{"Time":timestamp[], "Motor Y":dbl[]}[], element #11=→"CCD 11":cluster{"Time":timestamp[], "Motor Y":dbl[]}[], element #12=→"CCD 12":cluster{"Time":timestamp[], "Motor Y":dbl[]}[])  [unwired: 12 in]
          }
          frame "---------------Statistics--------------" {
            # "Template Separator\n(You can make a copy of, or modify, this frame)"
            n777 = call <vilib>:"Add State(s) to Queue__jki_lib_state_machine.vi"("State(s) in (\"\")"=w1509) -> ("States Out"=w1508:string)  [unwired: 14 in]
          }
          frame "Save Stats" {
            # "Your code here.\n(You can make a copy of, or modify, this frame)"
            n778 = property on="CCD 1" class="XYGraph (strict)"() -> ("Value"=w1519:cluster{timestamp[], dbl[]}[])  [unwired: 2 in, 2 out]
            n779 = property on="CCD 2" class="XYGraph (strict)"() -> ("Value"=w1518:cluster{timestamp[], dbl[]}[])  [unwired: 2 in, 2 out]
            n780 = property on="CCD 3" class="XYGraph (strict)"() -> ("Value"=w1517:cluster{timestamp[], dbl[]}[])  [unwired: 2 in, 2 out]
            n781 = property on="CCD 4" class="XYGraph (strict)"() -> ("Value"=w1516:cluster{timestamp[], dbl[]}[])  [unwired: 2 in, 2 out]
            n782 = property on="CCD 5" class="XYGraph (strict)"() -> ("Value"=w1515:cluster{timestamp[], dbl[]}[])  [unwired: 2 in, 2 out]
            n783 = property on="CCD 6" class="XYGraph (strict)"() -> ("Value"=w1514:cluster{timestamp[], dbl[]}[])  [unwired: 2 in, 2 out]
            n784 = property on="CCD 7" class="XYGraph (strict)"() -> ("Value"=w1513:cluster{timestamp[], dbl[]}[])  [unwired: 2 in, 2 out]
            n785 = property on="CCD 8" class="XYGraph (strict)"() -> ("Value"=w1512:cluster{timestamp[], dbl[]}[])  [unwired: 2 in, 2 out]
            n786 = Build Array(w1519, w1518, w1517, w1516, w1515, w1514, w1513, w1512) -> (w1511:cluster{timestamp[], dbl[]}[][])
            n787 = for {
              tunnel: w1511 -> [w1527] mode=indexing
              tunnel: w1510 -> [w1526] mode=indexing
              n788 = Empty String/Path?(string/path=w1526) -> (empty?=w1525:bool)
              n789 = case shown="False" w1525 {
                tunnel: w1527 -> [w1533 _]
                tunnel: w1526 -> [w1531 _]
                frame False {
                  n790 = Index Array(array=w1533, index #1=0 ("index"), index #2=1 ("index"), index #3=2 ("index"), index #4=3 ("index")) -> (element #1=w1568:cluster{timestamp[], dbl[]}, element #2=w1562:cluster{timestamp[], dbl[]}, element #3=w1561:cluster{timestamp[], dbl[]}, element #4=w1560:cluster{timestamp[], dbl[]})  [unwired: 1 in, 1 out]
                  n791 = Concatenate Strings(w1531, ".dat" ("string")) -> (w1529:string)
                  n792 = Unbundle(w1568) -> (w1567:timestamp[], w1545:dbl[])
                  n793 = Unbundle(w1562) -> (w1536:dbl[])  [unwired: 1 out]
                  n794 = Unbundle(w1561) -> (w1535:dbl[])  [unwired: 1 out]
                  n795 = Unbundle(w1560) -> (w1534:dbl[])  [unwired: 1 out]
                  n796 = Build Path(base path="save path", name or relative path=w1529) -> (appended path=w1528:path)
                  n797 = for {
                    tunnel: w1567 -> [w1570] mode=indexing
                    tunnel: [w1569] -> w1543 mode=indexing
                    n798 = Format Date/Time String(time format string (%c)="%Y%m%d%H%M%S", seconds (now)=w1570) -> (date/time string=w1569:string)  [unwired: 1 in]
                  }
                  n799 = Array Size(array=w1545) -> (size(s)=w1546:i32)
                  n800 = Number To Fractional String(number=w1545) -> (F-format string=w1542:string[])  [unwired: 3 in]
                  n801 = Number To Fractional String(number=w1536) -> (F-format string=w1539:string[])  [unwired: 3 in]
                  n802 = Number To Fractional String(number=w1535) -> (F-format string=w1538:string[])  [unwired: 3 in]
                  n803 = Number To Fractional String(number=w1534) -> (F-format string=w1537:string[])  [unwired: 3 in]
                  n804 = Initialize Array("", w1546, 5 ("dimension size")) -> (w1544:string[][])
                  n805 = Insert Into Array(array=w1544, index (col)=0 ("disabled index (col)"), new element=w1543) -> (w1554:string[][])  [unwired: 1 in]
                  n806 = Insert Into Array(array=w1554, index (col)=1 ("disabled index (col)"), new element=w1542) -> (w1553:string[][])  [unwired: 1 in]
                  n807 = Insert Into Array(array=w1553, index (col)=2 ("disabled index (col)"), new element=w1539) -> (w1557:string[][])  [unwired: 1 in]
                  n808 = Insert Into Array(array=w1557, index (col)=3 ("disabled index (col)"), new element=w1538) -> (w1558:string[][])  [unwired: 1 in]
                  n809 = Insert Into Array(array=w1558, index (col)=4 ("disabled index (col)"), new element=w1537) -> (w1559:string[][])  [unwired: 1 in]
                  n810 = Insert Into Array(array=w1559, index (row)=0, new element=string[] ["time", "Centroid X", "Centroid Y", "Motor Axis 1", "Motor Axis 2"] ("new element/subarray 2")) -> (w1541:string[][])  [unwired: 1 in]
                  n811 = call-poly <vilib>:"Write To Spreadsheet File.vi"("2D data"=w1541, "file path (dialog if empty)"=w1528) -> ()  [unwired: 6 in, 1 out]
                }
                frame True {
                }
              }
            }
            n812 = call <vilib>:"Add State(s) to Queue__jki_lib_state_machine.vi"("State(s) in (\"\")"=w1524) -> ("States Out"=w1523:string)  [unwired: 14 in]
            n813 = property on="Save Stats" class="Bool (strict)"("Value"=FALSE ("Save Stats")) -> ()  [unwired: 2 in, 2 out]
          }
          frame "tdms" {
            w1597 = 21600.0 ("new tdms")
            # "Your code here.\n(You can make a copy of, or modify, this frame)"
            n814 = Unbundle By Name(w1587) -> ("Data Value Reference out"=w1610:refnum<k34>, "Offset X"=w1612:dbl[][], "Offset Y"=w1607:dbl[][], "active axis refs 2"=w1609:T12)
            n815 = for {
              tunnel: w1612 -> [w1656]
              tunnel: w1607 -> [w1655]
              tunnel: w1611 -> [w1619] mode=indexing
              tunnel: w1610 -> [w1620]
              tunnel: w1609 -> [w1641]
              tunnel: w1608 -> [w1625]
              tunnel: [w1623] -> w1606
              i -> [w1642]
              n816 = Index Array(array=w1656, index (row)=w1642) -> (element=w1654:dbl[])  [unwired: 1 in]
              n817 = Index Array(array=w1655, index (row)=w1642) -> (element=w1653:dbl[])  [unwired: 1 in]
              n818 = Index Array(array=w1641, index=w1642) -> (element=w1640:cluster{"Ref X":refnum<vi>, "Ref Y":refnum<vi>})
              n819 = Reverse 1D Array(array=w1653) -> (reversed array=w1651:dbl[])
              n820 = Reverse 1D Array(array=w1654) -> (reversed array=w1652:dbl[])
              n821 = Unbundle By Name(w1640) -> ("Ref X"=w1639:refnum<vi>, "Ref Y"=w1638:refnum<vi>)
              n822 = Index Array(array=w1652) -> (element=w1650:dbl)  [unwired: 1 in]
              n823 = Index Array(array=w1651) -> (element=w1649:dbl)  [unwired: 1 in]
              n824 = property class="DigNum (strict)"(reference=w1639, error in=w1625) -> (error out=w1624:errorcluster, "Value"=w1633:dbl)  [unwired: 1 out]
              n825 = Build Array(w1650) -> (w1622:dbl[])
              n826 = Build Array(w1649) -> (w1644:dbl[])
              n827 = Get Date/Time In Seconds() -> (seconds since 1Jan1904=w1621:timestamp)
              n828 = Build Array(w1621) -> (w1617:timestamp[])
              n829 = property class="DigNum (strict)"(reference=w1638, error in=w1624) -> (error out=w1615:errorcluster, "Value"=w1627:dbl)  [unwired: 1 out]
              n830 = Build Array(w1633) -> (w1632:dbl[])
              n831 = TDMS Write(0:w1620, 5:w1619, 7:"time", 9:w1617, 11:w1615) -> (4:w1616:refnum<k34>, 15:w1614:errorcluster)  [unwired: 1 in, 2 out]
              n832 = Build Array(w1627) -> (w1626:dbl[])
              n833 = TDMS Write(0:w1616, 5:w1619, 7:"centroid X", 9:w1622, 11:w1614) -> (4:w1647:refnum<k34>, 6:w1646:string, 15:w1645:errorcluster)  [unwired: 1 in, 1 out]
              n834 = TDMS Write(0:w1647, 5:w1646, 7:"centroid Y", 9:w1644, 11:w1645) -> (4:w1636:refnum<k34>, 6:w1635:string, 15:w1637:errorcluster)  [unwired: 1 in, 1 out]
              n835 = TDMS Write(0:w1636, 5:w1635, 7:"Motor Axis 1", 9:w1632, 11:w1637) -> (4:w1631:refnum<k34>, 6:w1630:string, 15:w1628:errorcluster)  [unwired: 1 in, 1 out]
              n836 = TDMS Write(0:w1631, 5:w1630, 7:"Motor Axis 2", 9:w1626, 11:w1628) -> (15:w1623:errorcluster)  [unwired: 1 in, 3 out]
            }
            n837 = Unbundle By Name(w1587) -> ("img to avg"=w1585:i32)
            n838 = property on="millisecond timer value" class="DigNum (strict)"() -> ("Value"=w1574:u32)  [unwired: 2 in, 2 out]
            n839 = local read "millisecond timer 2"() -> (w1603:u32)
            n840 = Tick Count (ms)() -> (millisecond timer value=w1588:u32)
            n841 = call <userlib>:"Tick Count (ms)__ogtk.vi"("error in (no error)"=w1606) -> ("error out"=w1573:errorcluster, "millisecond timer value"=w1605:u32)  [unwired: 9 in]
            n842 = Subtract(x=w1588, y=w1574) -> (x-y=w1602:u32)
            n843 = Subtract(x=w1588, y=w1574) -> (x-y=w1589:u32)
            n844 = Subtract(x=w1605, y=w1603) -> (x-y=→"Waveform Chart":u32)
            n845 = Multiply(x=5.0 ("new tdms"), y=w1585) -> (x*y=w1583:dbl)
            n846 = Divide(x=w1602, y=u32 1000) -> (x/y=w1600:dbl)
            n847 = Divide(x=w1589, y=u32 1000) -> (x/y=w1591:dbl)
            n848 = Quotient & Remainder(x=w1600, y=w1597) -> (x-y*floor(x/y)=w1599:dbl)  [unwired: 1 out]
            n849 = Quotient & Remainder(x=w1591, y=w1583) -> (x-y*floor(x/y)=w1584:dbl)  [unwired: 1 out]
            "x-y*floor(x/y)" <- w1584
            n850 = Subtract(x=w1583, y=2.0) -> (x-y=w1581:dbl)
            n851 = Greater?(x=w1584, y=w1581) -> (0:w1580:bool)
            n852 = call <vilib>:"Clear Errors.vi"("error in (no error)"=w1573) -> ("error out"=w1572:errorcluster)  [unwired: 5 in, 1 out]
            n853 = Subtract(x=w1597, y=20.0) -> (x-y=w1595:dbl)
            n854 = Greater?(x=w1599, y=w1595) -> (0:w1598:bool)
            n855 = Select(t="Device Ini", s=w1580, f="") -> (s? t:f=w1577:string)
            n856 = Select(t="newtdms", s=w1598, f="") -> (s? t:f=w1592:string)
            n857 = call <vilib>:"Add State(s) to Queue__jki_lib_state_machine.vi"("State(s) in (\"\")"=w1613, "State(s) at Back (\"\")"=w1592) -> ("States Out"=w1576:string)  [unwired: 13 in]
            n858 = call <vilib>:"Add State(s) to Queue__jki_lib_state_machine.vi"("State(s) in Front (\"\")"=w1577, "State(s) in (\"\")"=w1576) -> ("States Out"=w1575:string)  [unwired: 13 in]
          }
          frame "Reset History" {
            # "Your code here.\n(You can make a copy of, or modify, this frame)"
            n859 = for {
              N: 1 -> [_]
              shift-right: [w1666] -> w1658
              shift-left: timestamp[][] [] ("Time") -> [w1668]
              n860 = for {
                N: 12 -> [_]
                tunnel: w1668 -> [w1671] mode=indexing
                tunnel: [w1669] -> w1666 mode=indexing
                n861 = Get Date/Time In Seconds() -> (seconds since 1Jan1904=w1670:timestamp)
                n862 = Build Array (concatenate)(w1671, w1670) -> (w1669:timestamp[])
              }
            }
            n863 = local read "Offset X"() -> (w1657:dbl[][])
            n864 = Bundle By Name(cluster=w1662, "Offset X"=w1657, "Offset Y"=w1657, "Time"=w1658, "Motor X"=w1657) -> (w1661:T37)
            n865 = call <vilib>:"Add State(s) to Queue__jki_lib_state_machine.vi"("State(s) in (\"\")"=w1665) -> ("States Out"=w1664:string)  [unwired: 14 in]
          }
          frame "New Category: 2" {
            # "Your code here.\n(You can make a copy of, or modify, this frame)"
            n866 = call <vilib>:"Add State(s) to Queue__jki_lib_state_machine.vi"("State(s) in (\"\")"=w1675) -> ("States Out"=w1674:string)  [unwired: 14 in]
          }
          frame "ImgToAvg" {
            # "Your code here.\n(You can make a copy of, or modify, this frame)"
            n867 = Decimal String To Number(string=w1679) -> (number=w1676:i32)  [unwired: 2 in, 1 out]
            n868 = Bundle By Name(cluster=w1678, "img to avg"=w1676) -> (w1677:T37)
            n869 = call <vilib>:"Add State(s) to Queue__jki_lib_state_machine.vi"("State(s) in (\"\")"=w1682) -> ("States Out"=w1681:string)  [unwired: 14 in]
          }
          frame "newtdms" {
            # "Your code here.\n(You can make a copy of, or modify, this frame)"
            n870 = Unbundle By Name(w1703) -> ("Data Value Reference out"=w1702:refnum<k34>, "active cams"=w1697:string[])
            n871 = TDMS Close(8:w1701, 11:w1702) -> (0:w1684:errorcluster)  [unwired: 1 out]
            n872 = Get Date/Time In Seconds() -> (seconds since 1Jan1904=w1695:timestamp)
            n873 = Format Date/Time String(time format string (%c)="%Y%m%d", seconds (now)=w1695) -> (date/time string=w1693:string)  [unwired: 1 in]
            n874 = Format Date/Time String(time format string (%c)="%Y%m%d%H%M", seconds (now)=w1695) -> (date/time string=w1705:string)  [unwired: 1 in]
            n875 = call <vilib>:"Clear Errors.vi"("error in (no error)"=w1684) -> ("error out"=w1683:errorcluster)  [unwired: 5 in, 1 out]
            n876 = Build Path(base path=w1694, name or relative path=w1693) -> (appended path=w1692:path)
            n877 = Concatenate Strings(w1705, "Beampointing_Pico.tdms" ("string")) -> (w1711:string)
            n878 = String To Path(string=w1711) -> (path=w1712:path)
            n879 = call <vilib>:"Check if File or Folder Exists.vi"("error in (no error)"=w1683, "path"=w1692) -> ("error out"=w1688:errorcluster, "file or folder exists?"=w1691:bool, "dup path"=w1690:path)  [unwired: 7 in]
            n880 = case shown="False" w1691 {
              tunnel: w1690 -> [w1719 w1721]
              tunnel: [w1718 w1721] -> w1689
              tunnel: w1688 -> [w1717 w1720]
              tunnel: [w1716 w1720] -> w1687
              frame False {
                n881 = Create Folder(path (use dialog)=w1719, error in=w1717) -> (created path=w1718:path, error out=w1716:errorcluster)  [unwired: 1 in, 1 out]
              }
              frame True {
              }
            }
            n882 = call <vilib>:"Add State(s) to Queue__jki_lib_state_machine.vi"("State(s) in (\"\")"=w1715) -> ("States Out"=w1714:string)  [unwired: 14 in]
            n883 = Build Path(base path=w1689, name or relative path=w1712) -> (appended path=w1706:path)
            n884 = TDMS Open(6:FALSE ("disable buffering (T)"), 7:enum16{"1.0", "2.0"}."2.0" ("file format version (2.0)"), 8:w1687, 10:T18."create or replace" ("operation"), 11:w1706) -> (0:w1698:errorcluster, 3:w1700:refnum<k34>)  [unwired: 2 in]
            n885 = call "TDMSbuffersize.vi"("error in (no error)"=w1698, "group names"=w1697, "Data Value Reference in"=w1700) -> ("error out"=w1686:errorcluster, "Data Value Reference out"=w1699:refnum<k34>)  [unwired: 7 in]
            n886 = Bundle By Name(cluster=w1703, "Data Value Reference out"=w1699) -> (w1704:T37)
            n887 = call <vilib>:"Clear Errors.vi"("error in (no error)"=w1686) -> ("error out"=w1685:errorcluster)  [unwired: 5 in, 1 out]
          }
          frame "Center" {
            # "Your code here.\n(You can make a copy of, or modify, this frame)"
            n888 = property on="Center" class="Bool (strict)"("Value"=FALSE ("Center")) -> ()  [unwired: 2 in, 2 out]
            n889 = control-ref of="image::1"() -> (w1736:refnum<vi>)
            n890 = control-ref of="image::2"() -> (w1735:refnum<vi>)
            n891 = control-ref of="image::3"() -> (w1734:refnum<vi>)
            n892 = control-ref of="image::4"() -> (w1733:refnum<vi>)
            n893 = control-ref of="image::5"() -> (w1732:refnum<vi>)
            n894 = control-ref of="image::6"() -> (w1731:refnum<vi>)
            n895 = control-ref of="image::7"() -> (w1730:refnum<vi>)
            n896 = control-ref of="image::8"() -> (w1729:refnum<vi>)
            n897 = control-ref of="image::9"() -> (w1728:refnum<vi>)
            n898 = control-ref of="image::10"() -> (w1727:refnum<vi>)
            n899 = control-ref of="image::11"() -> (w1726:refnum<vi>)
            n900 = control-ref of="image::12"() -> (w1725:refnum<vi>)
            n901 = for {
              tunnel: w1722 -> [w1749] mode=indexing
              tunnel: [w1744] -> w1737 mode=indexing
              n902 = Unbundle By Name(w1749) -> ("Target.X::12"=w1748:refnum<vi>, "Target.Y::12"=w1747:refnum<vi>)
              n903 = property class="DigNum (strict)"(reference=w1748) -> ("Value"=w1746:dbl)  [unwired: 1 in, 2 out]
              n904 = property class="DigNum (strict)"(reference=w1747) -> ("Value"=w1745:dbl)  [unwired: 1 in, 2 out]
              n905 = Bundle("Value"=w1746, "Value"=w1745) -> (w1744:cluster{"Value":dbl, "Value":dbl})  [unwired: 1 in]
            }
            n906 = call <vilib>:"Add State(s) to Queue__jki_lib_state_machine.vi"("State(s) in (\"\")"=w1741) -> ("States Out"=w1740:string)  [unwired: 14 in]
            n907 = Build Array(w1736, w1735, w1734, w1733, w1732, w1731, w1730, w1729, w1728, w1727, w1726, w1725) -> (w1724:refnum<vi>[])
            n908 = for {
              tunnel: w1724 -> [w1743] mode=indexing
              tunnel: w1737 -> [w1742] mode=indexing
              n909 = property class="ImageControl"(reference=w1743, "Image Center Position"=w1742) -> ()  [unwired: 1 in, 2 out]
            }
          }
          frame "history" {
            # "Your code here.\n(You can make a copy of, or modify, this frame)"
            n910 = Unbundle By Name(w1759) -> ("Offset X"=w1765:dbl[][], "Offset Y"=w1764:dbl[][], "Mean Centroid X"=w1763:dbl[][], "Mean Centroid Y"=w1762:dbl[][], "Motor X"=w1761:dbl[][], "Motor Y"=w1760:dbl[][], "Time"=w1751:timestamp[][])
            n911 = for {
              tunnel: w1765 -> [w1783] mode=indexing
              tunnel: w1764 -> [w1781] mode=indexing
              tunnel: w1763 -> [w1780] mode=indexing
              tunnel: w1762 -> [w1779] mode=indexing
              tunnel: w1761 -> [w1778] mode=indexing
              tunnel: w1760 -> [w1777] mode=indexing
              tunnel: [w1782] -> w1757 mode=indexing
              tunnel: [w1776] -> w1756 mode=indexing
              tunnel: [w1772] -> w1755 mode=indexing
              tunnel: [w1775] -> w1754 mode=indexing
              tunnel: [w1774] -> w1753 mode=indexing
              tunnel: [w1773] -> w1752 mode=indexing
              tunnel: w1751 -> [w1771] mode=indexing
              tunnel: [w1769] -> w1750 mode=indexing
              w1770 = 0
              n912 = Delete From Array(array=w1778, index=w1770) -> (array with subset deleted=w1774:dbl[])  [unwired: 1 in, 1 out]
              n913 = Delete From Array(array=w1777, index=w1770) -> (array with subset deleted=w1773:dbl[])  [unwired: 1 in, 1 out]
              n914 = Delete From Array(array=w1771, index=w1770) -> (array with subset deleted=w1769:timestamp[])  [unwired: 1 in, 1 out]
              n915 = Delete From Array(array=w1780, index=w1770) -> (array with subset deleted=w1772:dbl[])  [unwired: 1 in, 1 out]
              n916 = Delete From Array(array=w1779, index=w1770) -> (array with subset deleted=w1775:dbl[])  [unwired: 1 in, 1 out]
              n917 = Delete From Array(array=w1781, index=w1770) -> (array with subset deleted=w1776:dbl[])  [unwired: 1 in, 1 out]
              n918 = Delete From Array(array=w1783, index=w1770) -> (array with subset deleted=w1782:dbl[])  [unwired: 1 in, 1 out]
            }
            n919 = call <vilib>:"Add State(s) to Queue__jki_lib_state_machine.vi"("State(s) in (\"\")"=w1768) -> ("States Out"=w1767:string)  [unwired: 14 in]
            n920 = Bundle By Name(cluster=w1759, "Offset X"=w1757, "Offset Y"=w1756, "Mean Centroid X"=w1755, "Mean Centroid Y"=w1754, "Motor X"=w1753, "Motor Y"=w1752, "Time"=w1750) -> (w1758:T37)
          }
        }
        n921 = property on="Box" class="Arr (strict)"() -> ("Value"=w265:T6)  [unwired: 2 in, 2 out]
        n922 = for {
          tunnel: w267 -> [w293]
          tunnel: w266 -> [w294]
          tunnel: w259 -> [w288] mode=indexing
          tunnel: w265 -> [w289] mode=indexing
          tunnel: w256 -> [w285]
          (unwired) cluster{"xhair size":dbl, "xhair size 2":dbl} {"xhair size"=25.0, "xhair size 2"=25.0} ("size")
          (unwired) u32 16774656 ("Color")
          n923 = call-poly <userlib>:"Filter 1D Array__ogtk.vi"("items to filter"=w288, "array"=w294) -> ("filtered item indices"=w295:i32[])  [unwired: 4 in, 1 out]
          n924 = Index Array(array=w295) -> (element=w291:i32)  [unwired: 1 in]
          n925 = Index Array(array=w293, index=w291) -> (element=w292:T31)
          n926 = Unbundle By Name(w292) -> ("Target.X::12"=w297:refnum<vi>, "Target.Y::12"=w296:refnum<vi>)
          n927 = property class="DigNum (strict)"(reference=w297) -> ("Value"=w284:dbl)  [unwired: 1 in, 2 out]
          n928 = property class="DigNum (strict)"(reference=w296) -> ("Value"=w282:dbl)  [unwired: 1 in, 2 out]
          n929 = Bundle By Name(cluster=w285, "Target.x"=w284, "Target.y"=w282) -> (w283:T14)
          n930 = call "draw crosshair imaq.vi"("Crosshair"=w283, "Bounding Rectangle"=T16 {"Left"=0, "Top"=0, "Right"=0, "Bottom"=0}, "image in"=w288) -> ("error out"=→"error out":errorcluster, "image out"=w287:T9)  [unwired: 7 in]
          n931 = call "draw box imaq.vi"("Color"=u32 4336383, "Rectangle"=w289, "image in"=w287) -> ()  [unwired: 7 in, 2 out]
        }
        n932 = property on="ActiveMotor" class="Ring (strict)"() -> ("Strings []"=w261:string[])  [unwired: 2 in, 2 out]
        n933 = Index Array(array=w261, index="ActiveMotor") -> (element=w262:string)
        n934 = Not Equal?(x=w255, y=w262) -> (x != y?=w263:bool)
        n935 = case shown="True" w263 {
          tunnel: w261 -> [_ w281]
          tunnel: w255 -> [_ w280]
          frame False {
          }
          frame True {
            n936 = Search 1D Array(1D array=w281, element=w280) -> (index of element=w279:i32)  [unwired: 1 in]
            n937 = property on="ActiveMotor" class="Ring (strict)"("Value"=w279) -> ()  [unwired: 2 in, 2 out]
          }
        }
      }
      n938 = control-ref of="This Application"() -> (w246:refnum<vi>)
      n939 = control-ref of="This VI"() -> (w250:refnum<vi>)
      n940 = Current VI's Menubar() -> (w249:refnum<k9>)
      n941 = call "GUI_Master_subvi_reentrant_queues.vi"("STOP Queue in"=w33, "This Application"=w246, "error in (no error)"=w247, "tcp data event"=w245, "Caller menu reference"=w249, "Caller VI ref"=w250) -> ("error out"=→"error IO 2":errorcluster)  [unwired: 5 in]
      n942 = Unbundle By Name(w135) -> ("Data Value Reference out"=w134:refnum<k34>)
      n943 = for {
        tunnel: w164 -> [w254] mode=indexing
        tunnel: w163 -> [w253]
        tunnel: [w252] -> w133
        n944 = call "IMAQ Dispose"("Image"=w254, "error in (no error)"=w253) -> ("error out"=w252:errorcluster)  [unwired: 4 in]
      }
      n945 = TDMS Close(8:w133, 11:w134) -> (0:→"error out 2":errorcluster)  [unwired: 1 out]
    }
  }
